vi "AO_master_DM_WFS_v2.vi"() -> ()   [LabVIEW 2018]
uses:
  <userlib>/WaveKit.lib/Controls/Image information.ctl
  <userlib>/WaveKit.lib/Controls/Image general information.ctl
  <userlib>/WaveKit.lib/Controls/Image acquisition information.ctl
  <userlib>/WaveKit.lib/Controls/Point2D.ctl
  <userlib>/WaveKit.lib/Controls/Data alignment enum.ctl
  <userlib>/WaveKit.lib/Controls/StatisticsData.ctl
  <userlib>/WaveKit.lib/Controls/Wavefront Corrector states - ONE.ctl
  Drivers and controls/ASI/ASI_VIs/ASI Library/Shared_Serial/Axis Name.ctl
  <userlib>/WaveKit.lib/Classes/Camera/Camera.lvclass
  <userlib>/WaveKit.lib/Classes/CameraSet/CameraSet.lvclass
  <userlib>/WaveKit.lib/Classes/Image/Image.lvclass
  <userlib>/WaveKit.lib/Classes/Phase/Phase.lvclass
  <userlib>/WaveKit.lib/Controls/HasoSlopes.lvclass
  <userlib>/WaveKit.lib/Controls/Pupil.lvclass
  <userlib>/WaveKit.lib/Classes/WavefrontCorrector/WavefrontCorrector.lvclass
  <userlib>/WaveKit.lib/Classes/WavefrontCorrectorSet/WavefrontCorrectorSet.lvclass
  <userlib>/WaveKit.lib/Classes/HasoEngine/HasoEngine.lvclass
  <userlib>/WaveKit.lib/Controls/SlopesEngineSetup.ctl
  <userlib>/WaveKit.lib/Controls/WavefrontReconstructionMode.ctl
  <vilib>/Utility/file.llb/Read From Spreadsheet File (DBL).vi
  <vilib>/Analysis/1siggen.llb/Ramp Pattern by Delta.vi
  <userlib>/WaveKit.lib/Classes/ModalCoef/ModalCoef.lvclass
  <vilib>/Analysis/NI_AALBase.lvlib
panel:
  in  "File Type":enum16{"TIFF", "Sif"}(ring)
  in  "Spool":bool=TRUE caption="Cameras Live Display"
  in  "Device Status":enum32{"DM", "WFS", "Camera", "Others"}(tab)=enum."Camera"
  out "DM Actuator Values":sgl[](graph)
  out "Initial State":T1[](array[typedef])
  out "ActuatorsNumber":i32
  out "Initial Positions":sgl[](array[numeric])
  out "Final Positions":sgl[](array[numeric])
  in  "Coef Min":dbl=-0.5 min=1.0
  in  "Coef Max":dbl=0.5 min=1.0
  out "Zernike Measured":dbl[](graph)
  out "Phase statistics":T2
  out "Phase values":sgl[][](graph)=[[nan, nan, nan, nan, nan, nan, nan, nan, nan, nan, nan, nan, nan, nan, nan, nan, nan, nan, nan, nan, nan, nan, nan, nan, nan, nan, nan, nan, nan, nan, nan, nan, nan, nan, nan, nan, nan, nan, nan, nan], [nan, nan, nan, nan, nan, nan, nan, nan, nan, nan, nan, nan, nan, nan, nan, nan, nan, nan, nan, nan, nan, nan, nan, nan, nan, nan, nan, nan, nan, nan, nan, nan, nan, nan, nan, nan, nan, nan, nan, nan], [nan, nan, nan, nan, nan, nan, nan, nan, nan, nan, nan, nan, nan, nan, nan, nan, nan, nan, nan, nan, nan, nan, nan, nan, nan, nan, nan, nan, nan, nan, nan, nan, nan, nan, nan, nan, nan, nan, nan, nan], [nan, nan, nan, nan, nan, nan, nan, nan, nan, nan, nan, nan, nan, nan, nan, nan, nan, nan, nan, nan, nan, nan, nan, nan, nan, nan, nan, nan, nan, nan, nan, nan, nan, nan, nan, nan, nan, nan, nan, nan], [nan, nan, nan, nan, nan, nan, nan, nan, nan, nan, nan, nan, nan, nan, -0.14441992, nan, 0.1501734, 0.22490476, 0.2674259, 0.28415325, 0.2792031, 0.2552752, 0.21375881, 0.15405469, nan, nan, nan, nan, nan, nan, nan, nan, nan, nan, nan, nan, nan, nan, nan, nan], [nan, nan, nan, nan, nan, nan, nan, nan, nan, nan, nan, nan, nan, nan, 0.19143742, 0.2795512, 0.33646506, 0.37099743, 0.3877919, 0.3894302, 0.37774685, 0.35447162, 0.3212538, 0.27904776, 0.22675864, 0.15897867, nan, nan, nan, nan, nan, nan, nan, nan, nan, nan, nan, nan, nan, nan], [nan, nan, nan, nan, nan, nan, nan, nan, nan, nan, nan, nan, nan, 0.22618562, 0.290776, 0.33285964, 0.36044422, 0.3767934, 0.38285175, 0.37884915, 0.3652757, 0.3433441, 0.3149789, 0.28229773, 0.2464756, 0.20580466, 0.15268901, 0.06923797, nan, nan, nan, nan, nan, nan, nan, nan, nan, nan, nan, nan], [nan, nan, nan, nan, nan, nan, nan, nan, nan, nan, nan, nan, 0.19992779, 0.24616541, 0.27565512, 0.29675642, 0.31222007, 0.32191983, 0.32467726, 0.31943765, 0.30597392, 0.2852214, 0.25927368, 0.2309889, 0.20308714, 0.17653626, 0.14795627, 0.10568966, 0.024115691, nan, nan, nan, nan, nan, nan, nan, nan, nan, nan, nan], [nan, nan, nan, nan, nan, nan, nan, nan, nan, nan, nan, 0.14862825, 0.18219855, 0.20114602, 0.21551609, 0.22862102, 0.24014233, 0.24817906, 0.2505626, 0.24567793, 0.23295718, 0.21313797, 0.18829979, 0.16161954, 0.1367108, 0.11633411, 0.10019377, 0.081457645, 0.04156301, -0.057204023, nan, nan, nan, nan, nan, nan, nan, nan, nan, nan], [nan, nan, nan, nan, nan, nan, nan, nan, nan, nan, 0.08899155, 0.117771566, 0.12948777, 0.13732892, 0.14631097, 0.15688494, 0.16728252, 0.17497937, 0.17758016, 0.17335457, 0.16157834, 0.14275661, 0.11873307, 0.09261118, 0.06834036, 0.04974218, 0.038678437, 0.031985473, 0.016725859, -0.03676957, nan, nan, nan, nan, nan, nan, nan, nan, nan, nan], [nan, nan, nan, nan, nan, nan, nan, nan, nan, nan, 0.058377307, 0.069048055, 0.0725615, 0.07683456, 0.0840318, 0.09335055, 0.10271386, 0.1097376, 0.11226265, 0.10867052, 0.09812171, 0.08078306, 0.058033932, 0.032565817, 0.008214329, -0.010712444, -0.020921554, -0.022825297, -0.02489755, -0.05023362, -0.14592764, nan, nan, nan, nan, nan, nan, nan, nan, nan], [nan, nan, nan, nan, nan, nan, nan, nan, nan, -0.0018393314, 0.018310271, 0.023098737, 0.024714457, 0.027986258, 0.033823933, 0.041292578, 0.048749834, 0.054400377, 0.056548227, 0.05374936, 0.04499338, 0.029967438, 0.009379062, -0.014759185, -0.03905803, -0.059140373, -0.070816256, -0.0724436, -0.06894927, -0.07806298, -0.1393881, nan, nan, nan, nan, nan, nan, nan, nan, nan], [nan, nan, nan, nan, nan, nan, nan, nan, nan, -0.03322208, -0.017045017, -0.0123043535, -0.010394985, -0.007970343, -0.0042642877, 0.0003761826, 0.005164365, 0.009095938, 0.010986101, 0.009512841, 0.0033822758, -0.008344227, -0.02579559, -0.047820807, -0.071688615, -0.09321856, -0.107681155, -0.11187886, -0.10789668, -0.10908524, -0.14891545, -0.29341945, nan, nan, nan, nan, nan, nan, nan, nan], [nan, nan, nan, nan, nan, nan, nan, nan, nan, nan, -0.043187555, -0.03622458, -0.033755217, -0.03278728, -0.03198469, -0.030707732, -0.028716512, -0.026208155, -0.023933899, -0.023217455, -0.025771504, -0.03328519, -0.04682974, -0.06620631, -0.08943447, -0.1126552, -0.13079928, -0.13944486, -0.13836564, -0.13734597, -0.16491348, -0.2807172, nan, nan, nan, nan, nan, nan, nan, nan], [nan, nan, nan, nan, nan, nan, nan, nan, -0.13038255, -0.08328184, -0.060542934, -0.050779276, -0.048053104, -0.048984695, -0.05126809, -0.053124577, -0.05330209, -0.051303368, -0.04760214, -0.04368073, -0.041799206, -0.04448101, -0.05377527, -0.07043236, -0.09320336, -0.118551016, -0.14113419, -0.15550357, -0.15952203, -0.16009864, -0.18189941, -0.27977645, nan, nan, nan, nan, nan, nan, nan, nan], [nan, nan, nan, nan, nan, nan, nan, nan, -0.15416794, -0.09987456, -0.07151361, -0.05893044, -0.056102008, -0.058817875, -0.063637674, -0.067669004, -0.06878706, -0.06599128, -0.059670344, -0.051622536, -0.044753395, -0.042448726, -0.04769562, -0.062100213, -0.08502676, -0.11315687, -0.14084403, -0.16171429, -0.1720384, -0.17647736, -0.19687745, -0.284868, -0.53908885, -1.12795, nan, nan, nan, nan, nan, nan], [nan, nan, nan, nan, nan, nan, nan, nan, -0.17633308, -0.1131372, -0.07876157, -0.06330658, -0.060116876, -0.063924976, -0.07015394, -0.07493687, -0.07548633, -0.07052183, -0.060539607, -0.047784284, -0.035856243, -0.028966732, -0.030924596, -0.044017438, -0.06802279, -0.099662215, -0.13288532, -0.16044727, -0.17731819, -0.18653797, -0.20820689, -0.29237592, -0.5366785, nan, nan, nan, nan, nan, nan, nan], [nan, nan, nan, nan, nan, nan, nan, nan, -0.19826387, -0.12505035, -0.08430402, -0.06564974, -0.061443567, -0.06527472, -0.07152294, -0.07554153, -0.07411167, -0.0658889, -0.05163869, -0.034133032, -0.017655006, -0.0071354215, -0.007018423, -0.020031396, -0.046107426, -0.08178567, -0.12048963, -0.15415914, -0.17678727, -0.19048853, -0.21480094, -0.2999987, -0.54526997, nan, nan, nan, nan, nan, nan, nan], [nan, nan, nan, nan, nan, nan, nan, nan, -0.2214154, -0.13693352, -0.08914254, -0.06661926, -0.06048554, -0.06317037, -0.0681367, -0.07015528, -0.065784656, -0.053790003, -0.035310905, -0.013662348, 0.0062713036, 0.01901285, 0.01972933, 0.005542416, -0.023349542, -0.06307545, -0.10643376, -0.14466219, -0.17119798, -0.18806857, -0.21562657, -0.30642, -0.5640642, nan, nan, nan, nan, nan, nan, nan], [nan, nan, nan, nan, nan, nan, nan, nan, -0.24718054, -0.14940841, -0.093277775, -0.0658183, -0.056708053, -0.05720259, -0.059951056, -0.05929426, -0.051715773, -0.036192447, -0.014265999, 0.010266874, 0.032073133, 0.04536258, 0.04520398, 0.028878966, -0.0030008797, -0.045963787, -0.092160165, -0.13235793, -0.16002774, -0.17817038, -0.20961209, -0.31157303, -0.5953845, nan, nan, nan, nan, nan, nan, nan], [nan, nan, nan, nan, nan, nan, nan, nan, -0.27748746, -0.16290864, -0.09610232, -0.062047683, -0.048735943, -0.04617936, -0.046241976, -0.042900223, -0.03261665, -0.014586102, 0.009311387, 0.03494107, 0.05674191, 0.068891875, 0.0666744, 0.04783368, 0.0136316735, -0.030755527, -0.0769404, -0.115639456, -0.14119013, -0.15893419, -0.19620675, -0.31774768, nan, nan, nan, nan, nan, nan, nan, nan], [nan, nan, nan, nan, nan, nan, nan, nan, -0.31623095, -0.17884897, -0.09729818, -0.0539262, -0.03469713, -0.028198741, -0.025418447, -0.019910373, -0.008048305, 0.010862423, 0.034768496, 0.05942371, 0.07931873, 0.0889112, 0.08400761, 0.06307276, 0.028166434, -0.014867521, -0.057410896, -0.09080534, -0.111413695, -0.12868427, -0.17697167, -0.3319423, nan, nan, nan, nan, nan, nan, nan, nan], [nan, nan, nan, nan, nan, nan, nan, nan, nan, -0.20170604, -0.09850275, -0.0411539, -0.0131010795, -0.0011654077, 0.0047943285, 0.01185911, 0.023955166, 0.041901454, 0.06374147, 0.08542206, 0.1018104, 0.10796184, 0.10047772, 0.0787158, 0.04554086, 0.007227666, -0.027947046, -0.052963093, -0.06777905, -0.08820889, -0.15871821, nan, nan, nan, nan, nan, nan, nan, nan, nan], [nan, nan, nan, nan, nan, nan, nan, nan, nan, -0.24239759, -0.10614249, -0.026831074, 0.015322472, 0.03581071, 0.046350636, 0.05505173, 0.06651187, 0.08204405, 0.10016226, 0.11737824, 0.12928592, 0.13183476, 0.12261822, 0.10192663, 0.073240966, 0.042765103, 0.017522467, 0.0014635092, -0.0110412, -0.045025453, -0.15884721, nan, nan, nan, nan, nan, nan, nan, nan, nan], [nan, nan, nan, nan, nan, nan, nan, nan, nan, nan, -0.13597216, -0.021381527, 0.04426403, 0.07956008, 0.09847209, 0.110732496, 0.122154154, 0.13505057, 0.14887714, 0.16113368, 0.16849175, 0.16803522, 0.1584293, 0.14075197, 0.118653886, 0.09743117, 0.0815231, 0.06987105, 0.048498146, -0.020404778, nan, nan, nan, nan, nan, nan, nan, nan, nan, nan], [nan, nan, nan, nan, nan, nan, nan, nan, nan, nan, nan, -0.04876471, 0.05625415, 0.117832564, 0.15310521, 0.17423762, 0.18897903, 0.20128381, 0.21210447, 0.22038196, 0.22418612, 0.221881, 0.21311647, 0.19937092, 0.1836943, 0.16922635, 0.15598845, 0.13537171, 0.081669986, nan, nan, nan, nan, nan, nan, nan, nan, nan, nan, nan], [nan, nan, nan, nan, nan, nan, nan, nan, nan, nan, nan, nan, 0.014031529, 0.121263236, 0.18738765, 0.22803904, 0.25380248, 0.2710389, 0.28282017, 0.2899857, 0.29225817, 0.2892868, 0.28139976, 0.26978248, 0.25571787, 0.23844866, 0.21115, 0.15442081, nan, nan, nan, nan, nan, nan, nan, nan, nan, nan, nan, nan], [nan, nan, nan, nan, nan, nan, nan, nan, nan, nan, nan, nan, nan, nan, 0.15212902, 0.2306162, 0.28129596, 0.31381333, 0.33402625, 0.3450995, 0.34855807, 0.34515002, 0.33529556, 0.31882071, 0.29360068, 0.25266168, nan, nan, nan, nan, nan, nan, nan, nan, nan, nan, nan, nan, nan, nan], [nan, nan, nan, nan, nan, nan, nan, nan, nan, nan, nan, nan, nan, nan, nan, nan, 0.1979487, 0.2623494, 0.30271748, 0.32490522, 0.33223343, 0.3261181, 0.30614072, 0.26925305, nan, nan, nan, nan, nan, nan, nan, nan, nan, nan, nan, nan, nan, nan, nan, nan], [nan, nan, nan, nan, nan, nan, nan, nan, nan, nan, nan, nan, nan, nan, nan, nan, nan, nan, nan, nan, nan, nan, nan, nan, nan, nan, nan, nan, nan, nan, nan, nan, nan, nan, nan, nan, nan, nan, nan, nan], [nan, nan, nan, nan, nan, nan, nan, nan, nan, nan, nan, nan, nan, nan, nan, nan, nan, nan, nan, nan, nan, nan, nan, nan, nan, nan, nan, nan, nan, nan, nan, nan, nan, nan, nan, nan, nan, nan, nan, nan], [nan, nan, nan, nan, nan, nan, nan, nan, nan, nan, nan, nan, nan, nan, nan, nan, nan, nan, nan, nan, nan, nan, nan, nan, nan, nan, nan, nan, nan, nan, nan, nan, nan, nan, nan, nan, nan, nan, nan, nan]] caption="Wavefront"
  out "HASO intensity":u32[][](graph)
  out "Intensity Graph":i32[][](graph)
  in  "Intensity Max":dbl=10000.0 min=1.0
  in  "Intensity Min":dbl=200.0 min=1.0
  in  "Auto Scale":bool=TRUE caption="PD Correction"
  out "Detector X Pixels":i32
  out "Detector Y Pixels":i32
  out "Current Temp":i32
  out "FOV X Pixels":i32
  out "FOV Y Pixels":i32
  out "Running Status":T3(ring) caption="Camera FOV"
  out "EMCCD Status":bool
  out "Return from Start Acquisition":u32
  out "Return from GetAcquiredData":u32
  out "Return from SetSpool":i32=1
  out "Return from GetStatus":u32
  out "Get Exposure Time":sgl format="%.4f"
  out "Return from CheckTimings":u32
  out "Get Accum Time":sgl format="%.4f"
  out "Get Kinetic Time":sgl format="%.4f"
  out "Get EMCCD Gain":i32=1
  out "Get Kinetic Num":i32=1
  out "Return from CheckProcess":u32
  in  "error in (no error)":errorcluster
  out "Current error":errorcluster
  out "AO output":path=path "D:/Data"
  out "nb_images (get)":u32=10
  out "exposure_duration_us (get)":u32
  out "Base Path":path=path "D:/Data"
  out "EMCCD output":path=path "D:/Data"
  in  "Current status":string="Test1"
  out "HASO ready":bool
  in  "Live Wavefront":bool
  in  "Update DM":bool
  in  "Tab Control":T4(tab)
  in  "EMCCD trigger port":tag="Dev1/port0/line0"
  in  "strPalette":string="C:\\Program Files\\Andor SOLIS\\GREY.PAL"
  in  "Initial haso file":path=path "D:/SystemAlignment/system_aberration_residual_20220406.has"
  in  "interaction matrix file":path=path "D:/SystemAlignment/IM_20220407_1p5sx2_0p5um.aomi"
  in  "DM configuration file":path=path "C:/Program Files (x86)/Imagine Optic/Configuration Files/WaveFrontCorrector_mirao52-e_0326.dat"
  in  "Haso configuration file":path=path "C:/Program Files (x86)/Imagine Optic/Configuration Files/HASO3_first_7364.dat"
  in  "Main Path":path=path "D:/Data"
  in  "Folder Name":string="Test"
  in  "Abort":bool
  in  "Snap":bool
  in  "Acquire":bool
  in  "Enable EMCCD":bool caption="PD Correction"
  in  "TurnOFFCooler":bool caption="PD Correction"
  in  "Shutdown EMCCD when exit":bool caption="PD Correction"
  in  "VISA Stage":refnum<visa-resource-name>="COM5"
  in  "Update FOV":bool
  in  "Yend":i32=1002
  in  "Xend":i32=1004
  in  "Ystart":i32=2
  in  "Xstart":i32=2
  in  "Ybin":i32=1
  in  "Xbin":i32=1
  in  "Camera FOV":T5(ring)=enum."Full FOV"
  in  "Update AcqSetting":bool
  in  "Exposure time (s)":dbl=0.02
  in  "Kinetic Num":u32=1
  in  "Accum Num":u32=1
  in  "Aquisition Mode":T6(ring)=enum."Single Scan" caption="Camera FOV"
  in  "Trigger Mode":enum16{"Internal", "External"}(ring) caption="Camera FOV"
  in  "Gain Value":sgl=20.0 format="%.2f"
  in  "Gain On":bool=TRUE caption="Cameras Live Display"
  in  "488 shutter":refnum<k7>(container)
  in  "Live EMCCD":bool
  in  "Initialize EMCCD":bool=TRUE caption="PD Correction"
  in  "CoolToTargetTemp":bool=TRUE caption="PD Correction"
  in  "Set Temp":i32=-60
  in  "Current Z as Center":bool=TRUE caption="PD Correction"
  in  "Subfolder EMCCD":string="test"
  in  "File Name":string="test"
  in  "Z Step Num":i32=7
  in  "Z Step Size (um)":dbl=0.2
  in  "right":bool
  in  "left":bool
  in  "front":bool
  in  "back":bool
  in  "XY step":dbl=1.0
  in  "down":bool
  in  "up":bool
  in  "Z step":dbl=1.0
  in  "flip mirror button":bool
  out "Response:":string="0\r"
  out "Position (um)":dbl[](array[numeric])=[0.0, 0.0, 0.0, -92.0, nan, nan] format="%#.1f"
  in  "Axis":T7[](array[typedef])=[enum."X", enum."Y", enum."Z", enum."Z", enum."F", enum."V"]
  in  "Command":string="W X"
  in  "Get Position":bool
  in  "Send":bool
  in  "Record Batch Actuator":bool
  in  "Coef value":dbl=0.5 min=1.0
  in  "Idx end":u32=20 min=1
  in  "Idx start":u32=1 min=1
  in  "Subfolder":string="Test1"
  in  "Net Rp":bool
  in  "Input type":T8(ring)=enum."Zernike Coef"
  in  "Additional Command":bool=TRUE
  in  "Offset command file":path=path "D:/SystemAlignment/system_aberration_20220414.dat"
  in  "Initial offset":bool=TRUE
  in  "Additional file":path=path "D:/SystemAlignment/system_aberration_20191029.dat"
  out "Coef out":sgl[](array[numeric])
  out "Index out":i32[](array[numeric])
  in  "Zern/DM index in":i32[](array[numeric])
  in  "Zern/DM coef in":sgl[](array[numeric])
  in  "idxType":enum16{"Wyant", "ANSI"}(ring)=enum."ANSI"
  in  "Filter":u8[](array[numeric])
  in  "exposure_duration_s (set)":dbl=1.0 min=1.0
  in  "nb_images (set)":u32=1 min=1
  in  "Save File":bool
  in  "File Base Name":string="Test"
  in  "Record Response":bool
  in  "Record Batch Zern":bool
  out "Acquisition information":T9={"Image general information"={"Camera serial number"="", "Smearing removed"=FALSE, "Background image removed"=FALSE, "Time Stamp"=timestamp(0 s since 1904-01-01), "Comment"="", "Camera_MAX_Level"=0}, "Acquisition information"={"Exposure duration (us)"=0, "Exposure duration specified (us)"=0, "Gain"=0.0, "Number of summed images"=0, "Trigger type"=""}, "Number of pixels"={"X"=0, "Y"=0}, "Number of bits"=enum."16"}
  in  "Init":bool
  in  "Reset error":bool
  in  "Exit":bool
  in  "Stop HASO":bool
  in  "Start HASO":bool
  # "AO_master_DM_WFS_v2.vi: (last update: 20220425)\nControl deformable mirror and wavefront sensor, check DM response, EMCCD preview and acquisition\n1, Add ASI stage and laser shutter control;\n2, Incorporate EMCCD control: 1) preview, 2) snap,  3) stack acquisition (by moving relative Z position);\n3,  Current bugs: 1) error --> shut down devices; 2) exit --> next initialization fails\na) DM ocuppied due to last unnormal exit; b) wavefront measure error: no laser, wrong slopes;"
  # "um"
  # "Available only if \"Live Wavefront\" is OFF"
  # "Not work well"
  # "Sample Stage"
  # "It takes some time to cool down the camera before it shutdowns"
  # "WF switch"
  # "Tilt 1/X: +"
  # "Defocus: +"
  # "C"
  # "Tilt 2/Y: -"
  # "1um = 10"
  # "Acquisition Settings"
  # "WFS no tilt: X502, Y520 @EMCCD"
  # "HASO Parameters"
  # "Check DM Response"
  # "Need to turn OFF live wavefront"
  # "Batch Range"
  # "Show in Wyant convention"
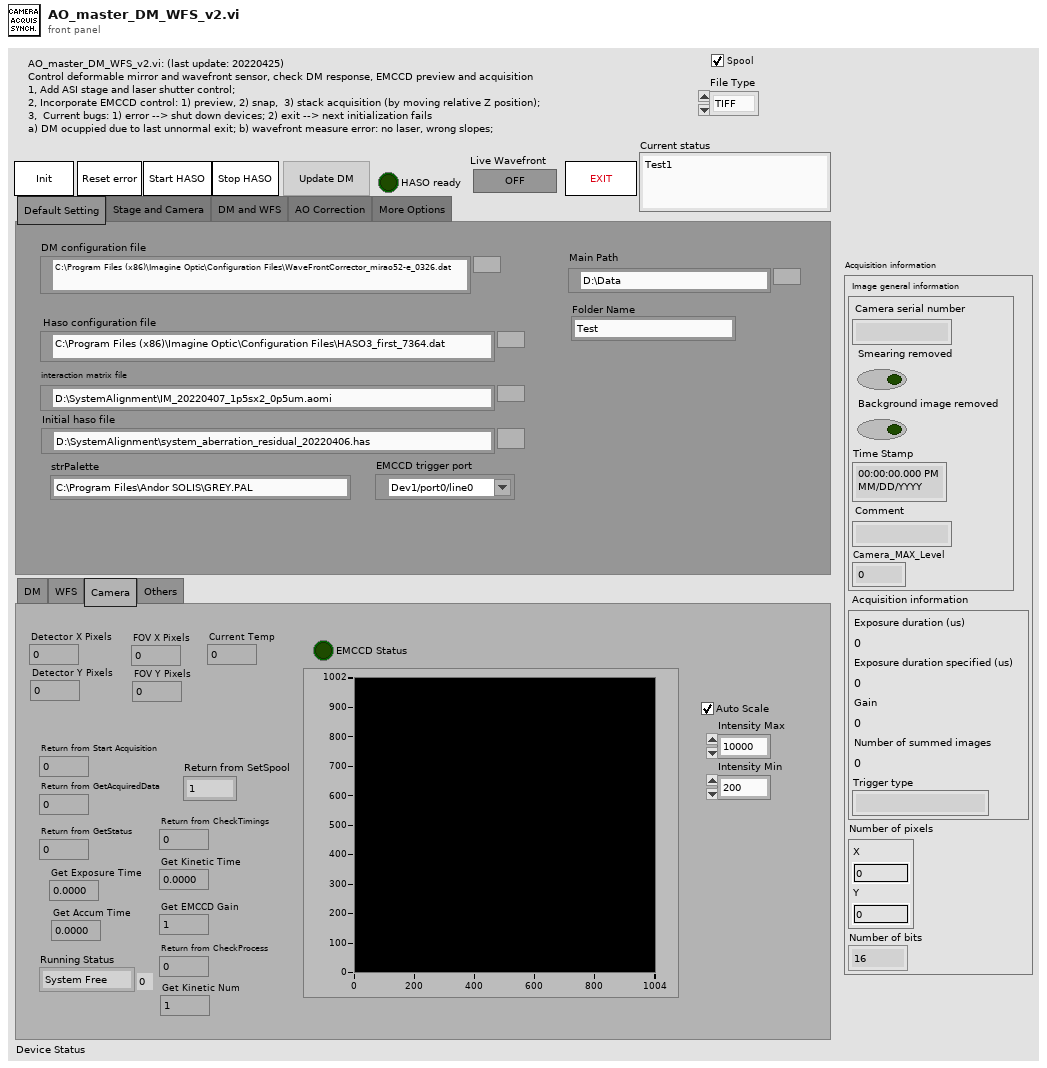
[diagram p1: front panel]
types:
  T1 = typedef "Wavefront Corrector states - ONE.ctl" = cluster{"Max":sgl, "Min":sgl, "Validity":enum16{"valid", "fixed", "invalid"}, "Fixed_Position":sgl}
  T2 = typedef "StatisticsData.ctl" = cluster{"PV":sgl, "RMS":dbl, "Max":sgl, "Min":sgl}
  T3 = enum16{"System Free", "Live Preview", "Snap", " Acquisition", ""}
  T4 = enum32{"Default Setting", "Stage and Camera", "DM and WFS", "AO Correction", "More Options"}
  T5 = enum16{"Custom FOV", "Full FOV", "FOV: 768x768", "FOV: 512x512", "FOV: 320x320", "FOV: 256x256", ""}
  T6 = enum16{"None", "Single Scan", "Accumulate", "Kinetics", "Fast Kinetics", "Run till abort"}
  T7 = typedef "Axis Name.ctl" = enum8{"undefined", "A", "B", "C", "D", "E", "F", "G", "H", "I", "J", "K", "L", "M", "N", "O", "P", "Q", "R", "S", "T", "U", "V", "W", "X", "Y", "Z"}
  T8 = enum16{"Zero Input", "Command File", "Zernike Coef", "Zernike File", "DM actuators"}
  T9 = typedef "Image information.ctl" = cluster{"Image general information":T10, "Acquisition information":T11, "Number of pixels":T12, "Number of bits":T13}
  T10 = typedef "Image general information.ctl" = cluster{"Camera serial number":string, "Smearing removed":bool, "Background image removed":bool, "Time Stamp":timestamp, "Comment":string, "Camera_MAX_Level":i32}
  T11 = typedef "Image acquisition information.ctl" = cluster{"Exposure duration (us)":i32, "Exposure duration specified (us)":i32, "Gain":sgl, "Number of summed images":i32, "Trigger type":string}
  T12 = typedef "Point2D.ctl" = cluster{"X":u32, "Y":u32}
  T13 = typedef "Data alignment enum.ctl" = enum16{"8", "16", "32"}
  T14 = typedef "SlopesEngineSetup.ctl" = cluster{"Start sub-aperture":T12, "Pupil average":dbl}
  T15 = typedef "CameraSpecifications.ctl" = cluster{"Grabber name":string, "Camera name":string, "Camera sn":string, "Pixels_um":T16, "Maximum level":u32, "Data alignment":T13, "Is signed":bool, "Acquisition start":T12, "Acquisition length":T12, "MaxFrameRate_Hz":sgl, "Chip type":enum16{"Progressive scan", "Frame transfert"}}
  T16 = typedef "General dimensions definition.ctl" = cluster{"Size":T12, "Step":T17}
  T17 = typedef "Point2Df.ctl" = cluster{"X":sgl, "Y":sgl}
  T18 = typedef "Wavefront Corrector Position.ctl" = sgl[]
  T19 = typedef "WavefrontReconstructionMode.ctl" = enum16{"None", "Modal_Legendre", "Modal_Zernike", "Zonal", "Modal_Zonal_Zernike", "Modal_Zonal_Legendre"}
  T20 = typedef "Error Code Enum typedef.ctl" = enum32{"N/A (0)", "DRV_ERROR_CODES", "DRV_SUCCESS", "DRV_VXDNOTINSTALLED", "DRV_ERROR_SCAN", "DRV_ERROR_CHECK_SUM", "DRV_ERROR_FILELOAD", "DRV_UNKNOWN_FUNC", "DRV_ERROR_VXD_INIT", "DRV_ERROR_ADDRESS", "DRV_ERROR_PAGELOCK", "DRV_ERROR_PAGEUNLOCK", "DRV_ERROR_BOARDTEST", "DRV_ERROR_ACK", "DRV_ERROR_UP_FIFO", "DRV_ERROR_PATTERN", "N/A (16)", "DRV_ACQUISITION_ERRORS", "DRV_ACQ_BUFFER", "DRV_ACQ_DOWNFIFO_FULL", "DRV_PROC_UNKONWN_INSTRUCTION", "DRV_ILLEGAL_OP_CODE", "DRV_KINETIC_TIME_NOT_MET", "DRV_ACCUM_TIME_NOT_MET", "DRV_NO_NEW_DATA", "N/A (25)", "DRV_SPOOLERROR", "N/A (27)", "N/A (28)", "N/A (29)", "N/A (30)", "N/A (31)", "N/A (32)", "DRV_TEMPERATURE_CODES", "DRV_TEMPERATURE_OFF", "DRV_TEMPERATURE_NOT_STABILIZED", "DRV_TEMPERATURE_STABILIZED", "DRV_TEMPERATURE_NOT_REACHED", "DRV_TEMPERATURE_OUT_RANGE", "DRV_TEMPERATURE_NOT_SUPPORTED", "DRV_TEMPERATURE_DRIFT", "N/A (41)", "N/A (42)", "N/A (43)", "N/A (44)", "N/A (45)", "N/A (46)", "N/A (47)", "N/A (48)", "DRV_GENERAL_ERRORS", "DRV_INVALID_AUX", "DRV_COF_NOTLOADED", "DRV_FPGAPROG", "DRV_FLEXERROR", "DRV_GPIBERROR", "N/A (55)", "N/A (56)", "N/A (57)", "N/A (58)", "N/A (59)", "N/A (60)", "N/A (61)", "N/A (62)", "N/A (63)", "DRV_DATATYPE", "DRV_DRIVER_ERRORS", "DRV_P1INVALID", "DRV_P2INVALID", "DRV_P3INVALID", "DRV_P4INVALID", "DRV_INIERROR", "DRV_COFERROR", "DRV_ACQUIRING", "DRV_IDLE", "DRV_TEMPCYCLE", "DRV_NOT_INITIALIZED", "DRV_P5INVALID", "DRV_P6INVALID", "DRV_INVALID_MODE", "DRV_INVALID_FILTER", "DRV_I2CERRORS", "DRV_I2CDEVNOTFOUND", "DRV_I2CTIMEOUT", "DRV_P7INVALID", "N/A (84)", "N/A (85)", "N/A (86)", "N/A (87)", "N/A (88)", "N/A (89)", "DRV_IOCERROR", "DRV_VRMVERSIONERROR"}
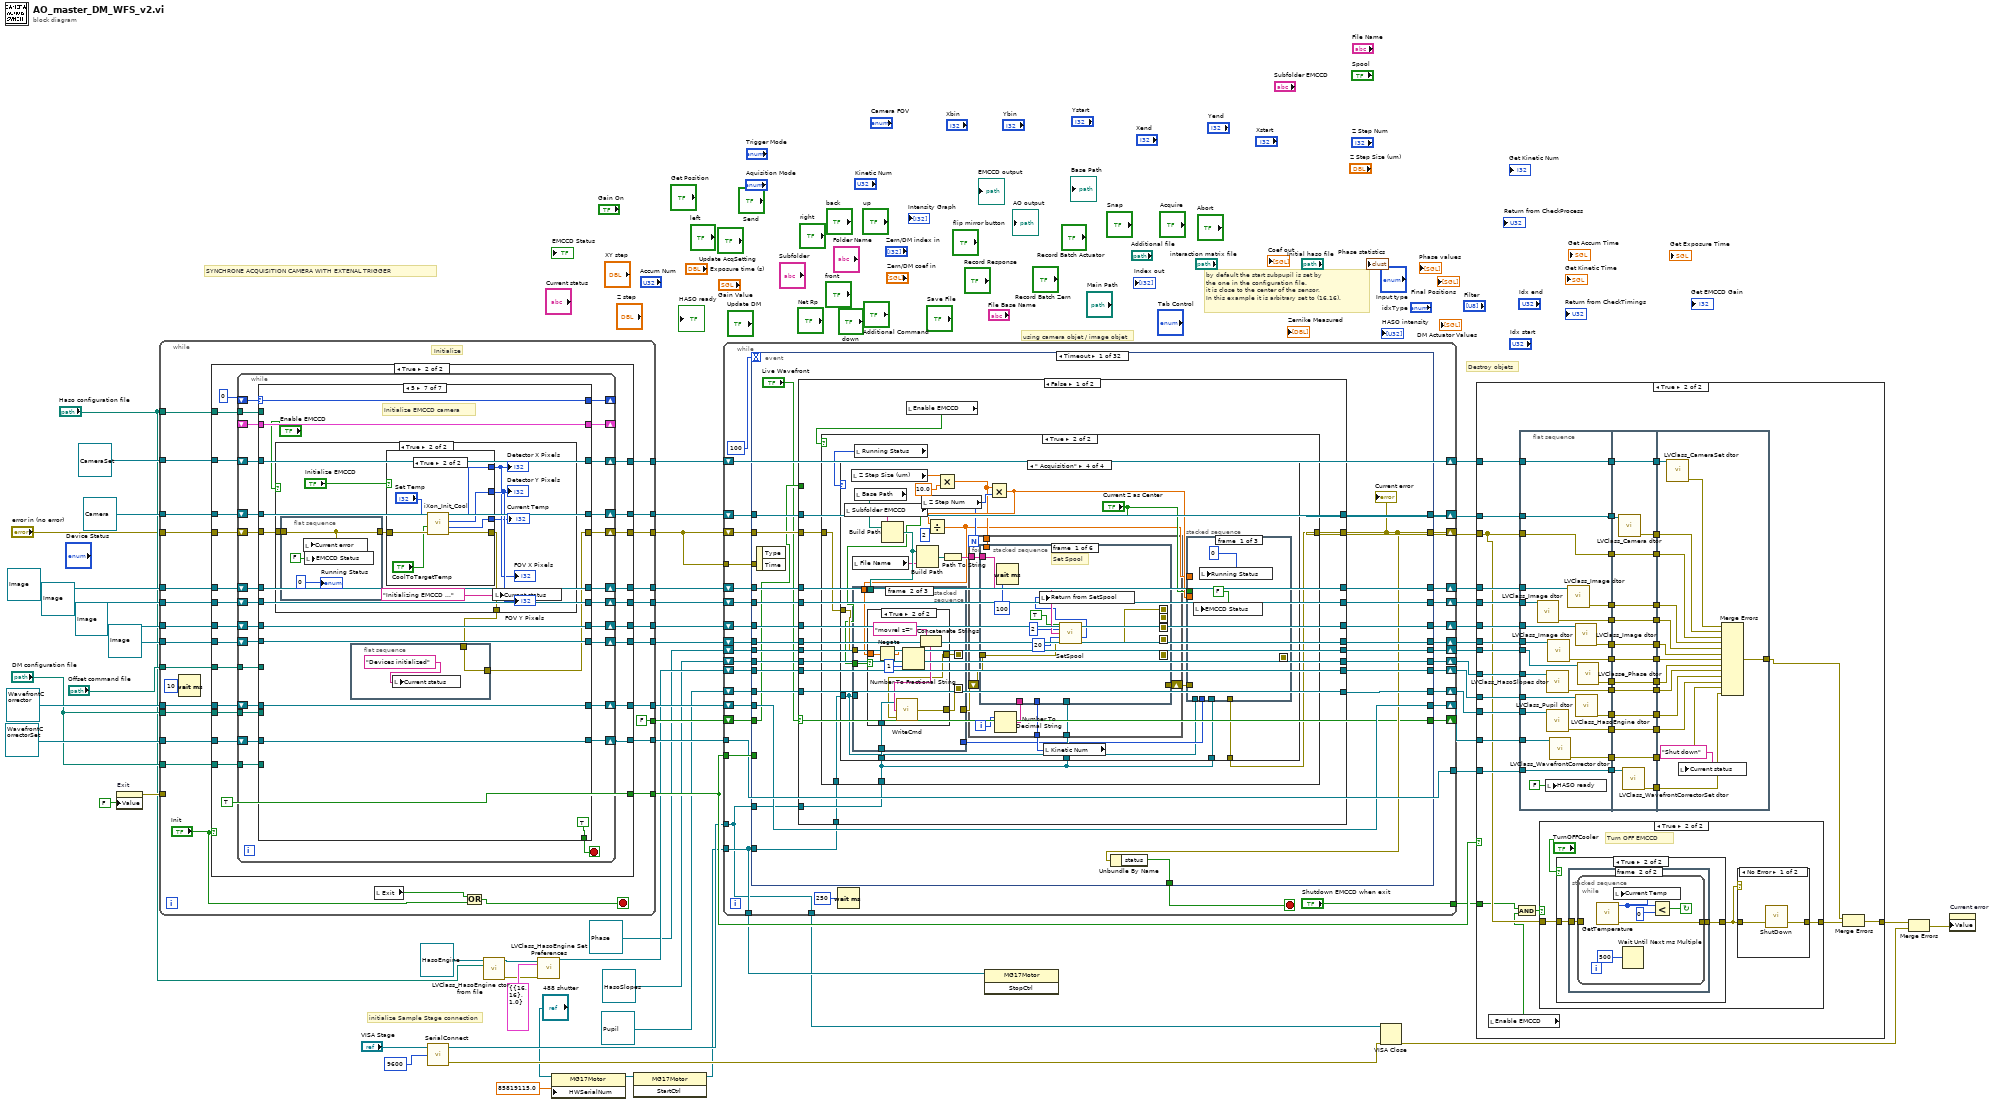
[diagram p0: block diagram]
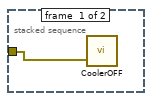
[diagram p5: hidden frame]
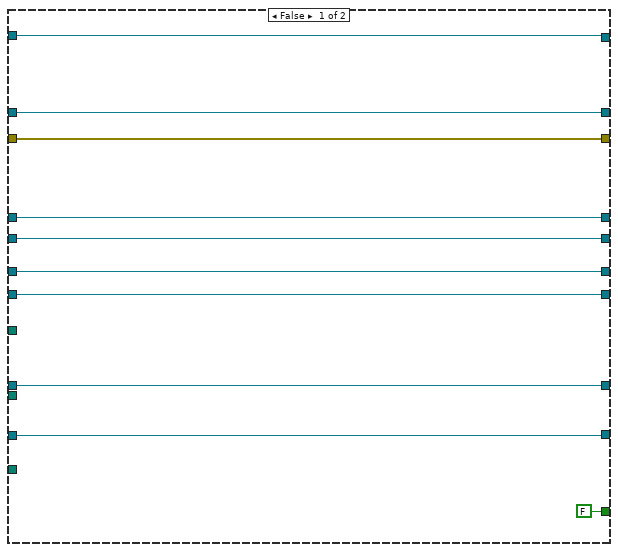
[diagram p7: hidden frame]
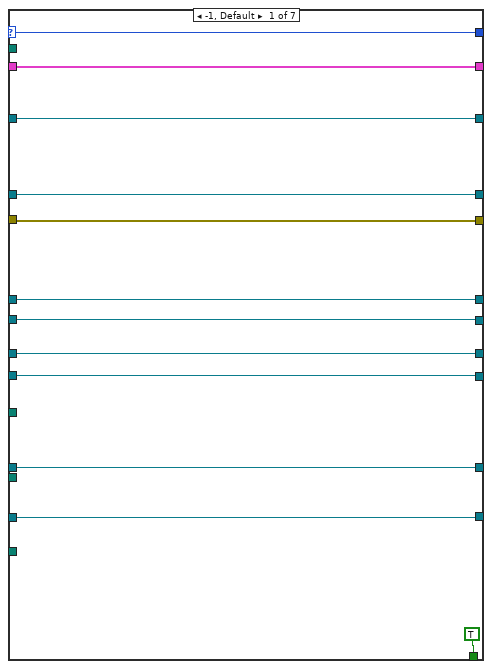
[diagram p8: hidden frame]
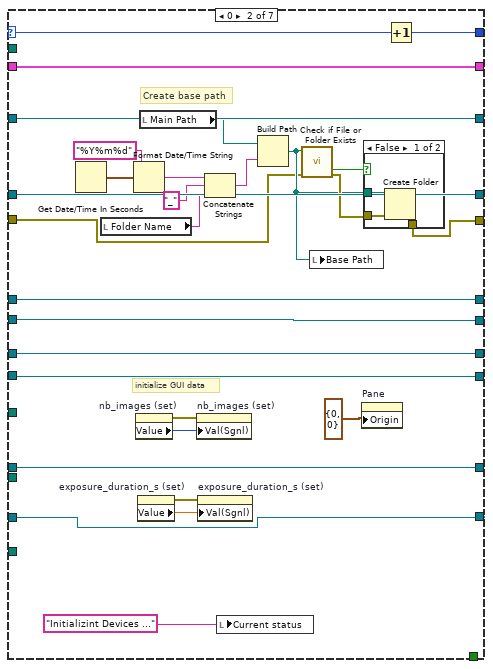
[diagram p9: hidden frame]
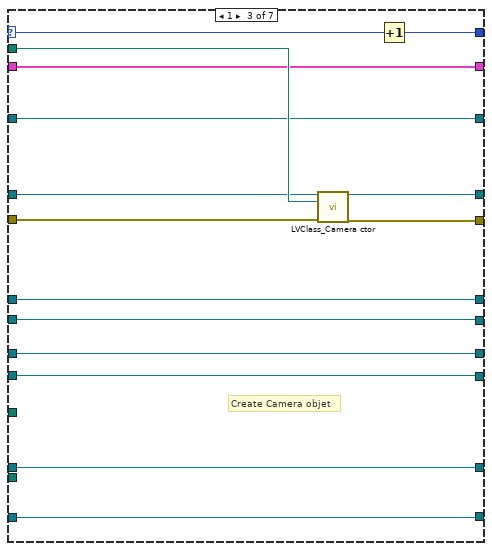
[diagram p11: hidden frame]
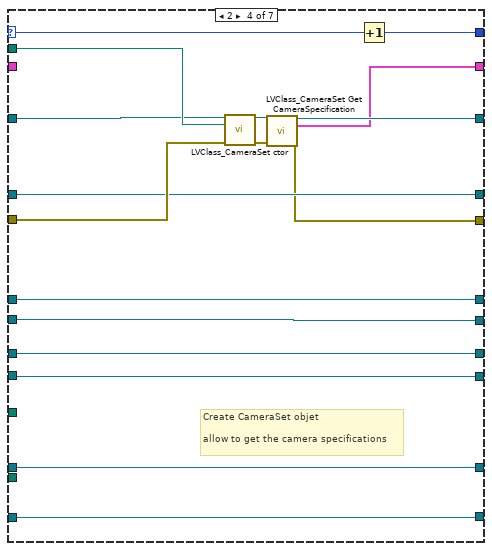
[diagram p12: hidden frame]
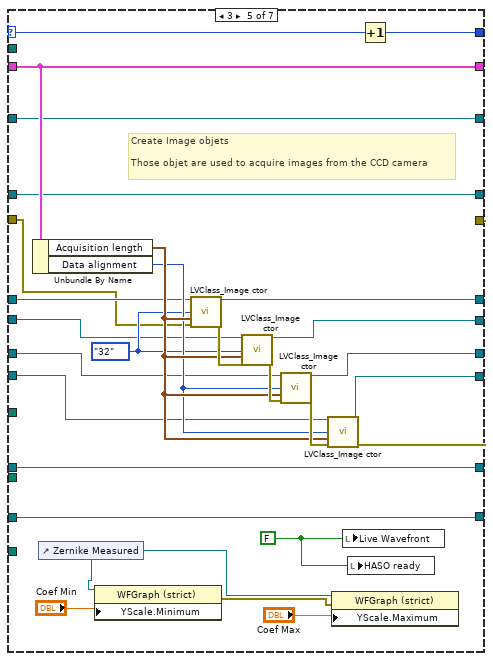
[diagram p13: hidden frame]
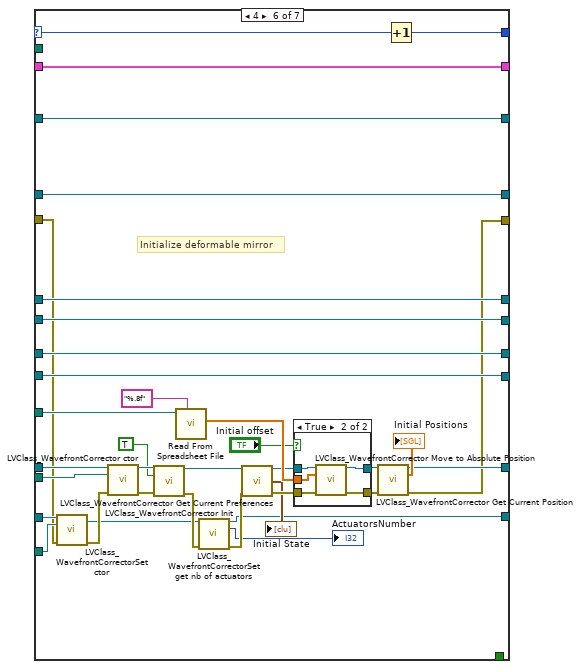
[diagram p14: hidden frame]
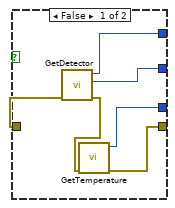
[diagram p17: hidden frame]
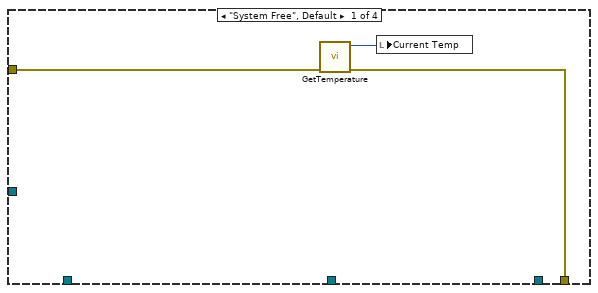
[diagram p19: hidden frame]
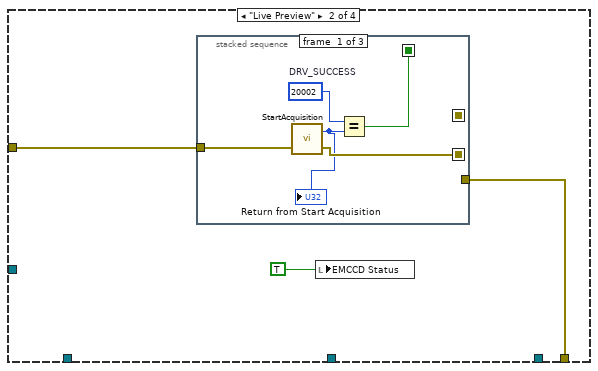
[diagram p20: hidden frame]
diagram:
  # "initialize Sample Stage connection"
  # "by default the start subpupil is set by \nthe one in the configuration file. \nit is close to the center of the sensor.\nIn this example it is arbitrary set to (16,16)."
  # "Destroy objets"
  # "using camera objet / image objet"
  # "SYNCHRONE ACQUISITION CAMERA WITH EXTENAL TRIGGER"
  n1 = property on="Exit" class="Bool (strict)"("Value"=FALSE ("Exit")) -> (error out=w37:errorcluster)  [unwired: 2 in, 1 out]
  n2 = while {
    tunnel: [FALSE] -> w53
    tunnel: [w87] -> w52
    tunnel: [w86] -> w51
    tunnel: [w85] -> w50
    tunnel: [w84] -> w49
    tunnel: [w83] -> w48
    tunnel: [w82] -> w47
    tunnel: refnum<class "Camera.lvclass"> refnum ("Camera.lvclass") -> [w81]
    tunnel: refnum<class "CameraSet.lvclass"> refnum ("CameraSet.lvclass") -> [w80]
    tunnel: refnum<class "Image.lvclass"> refnum ("Image in") -> [w79]
    tunnel: refnum<class "Image.lvclass"> refnum ("Image in") -> [w78]
    tunnel: refnum<class "Image.lvclass"> refnum ("Image in") -> [w77]
    tunnel: refnum<class "Image.lvclass"> refnum ("Image in") -> [w76]
    tunnel: "error in (no error)" -> [w75]
    tunnel: [w74] -> w40
    tunnel: [w72] -> w39
    tunnel: w37 -> [_]
    tunnel: "Haso configuration file" -> [w68]
    tunnel: "Offset command file" -> [w67]
    tunnel: refnum<class "WavefrontCorrectorSet.lvclass"> refnum ("WavefrontCorrectorSet in") -> [w66]
    tunnel: "DM configuration file" -> [w65]
    tunnel: refnum<class "WavefrontCorrector.lvclass"> refnum ("WavefrontCorrector in") -> [w64]
    tunnel: "DM configuration file" -> [w63]
    tunnel: [w62] -> w32
    tunnel: [w61] -> w31
    stop <- w69 stop-if-true
    # "Initialize"
    n3 = Wait (ms)(milliseconds to wait=u32 10) -> ()  [unwired: 1 out]
    n4 = case shown="True" "Init" {
      tunnel: [w98 w122] -> w87
      tunnel: [w97 w121] -> w86
      tunnel: [w95 w120] -> w85
      tunnel: [w94 w119] -> w84
      tunnel: [w93 w118] -> w83
      tunnel: [w92 w117] -> w82
      tunnel: w81 -> [w98 w116]
      tunnel: w80 -> [w97 w114]
      tunnel: w79 -> [w95 w113]
      tunnel: w78 -> [w94 w112]
      tunnel: w77 -> [w93 w111]
      tunnel: w76 -> [w92 w110]
      tunnel: w75 -> [w96 w109]
      tunnel: [w96 w108] -> w74
      tunnel: [FALSE TRUE] -> w72
      tunnel: w68 -> [_ w106]
      tunnel: w67 -> [_ w105]
      tunnel: w66 -> [w89 w99]
      tunnel: w65 -> [_ w104]
      tunnel: w64 -> [w90 w100]
      tunnel: w63 -> [_ w103]
      tunnel: [w90 w102] -> w62
      tunnel: [w89 w101] -> w61
      frame False {
      }
      frame True {
        n5 = while {
          tunnel: w106 -> [w147]
          shift-right: [w149] -> w122
          shift-left: w116 -> [w141]
          shift-right: [w131] -> _
          shift-left: 0 -> [w130]
          shift-right: [w148] -> w121
          shift-left: w114 -> [w140]
          shift-right: [w139] -> _
          shift-left: _ -> [w137]
          shift-right: [w146] -> w120
          shift-left: w113 -> [w138]
          shift-right: [w145] -> w119
          shift-left: w112 -> [w136]
          shift-right: [w144] -> w118
          shift-left: w111 -> [w134]
          shift-right: [w143] -> w117
          shift-left: w110 -> [w135]
          shift-right: [w142] -> w108
          shift-left: w109 -> [w132]
          tunnel: w105 -> [w129]
          tunnel: w104 -> [w128]
          tunnel: w103 -> [w127]
          shift-right: [w126] -> w102
          shift-left: w100 -> [w124]
          shift-right: [w125] -> w101
          shift-left: w99 -> [w123]
          stop <- w133 stop-if-true
          n6 = case shown="5" w130 {
            tunnel: [w161 w177 w209 w219 w241 w290 w312] -> w149
            tunnel: w147 -> [_ _ w208 w223 _ _ _]
            tunnel: [w160 w181 w206 w224 w242 w289 w311] -> w148
            tunnel: [w153 w182 w200 w214 w248 w284 w305] -> w146
            tunnel: [w154 w183 w201 w215 w247 w285 w306] -> w145
            tunnel: [w155 w184 w202 w216 w246 w286 w307] -> w144
            tunnel: [w156 w185 w203 w217 w245 w287 w308] -> w143
            tunnel: [w157 w163 w205 w218 w244 w258 w298] -> w142
            selector: w130 -> [w152 w179 w198 w213 w236 w256 w304]
            tunnel: w141 -> [w161 w177 w207 w219 w241 w290 w312]
            tunnel: w140 -> [w160 w181 w206 w222 w242 w289 w311]
            tunnel: [w158 w178 w204 w221 w243 w288 w309] -> w139
            tunnel: w138 -> [w153 w182 w200 w214 w240 w284 w305]
            tunnel: w137 -> [w158 w178 w204 _ w243 w288 w309]
            tunnel: w136 -> [w154 w183 w201 w215 w239 w285 w306]
            tunnel: w135 -> [w156 w185 w203 w217 w238 w287 w308]
            tunnel: w134 -> [w155 w184 w202 w216 w237 w286 w307]
            tunnel: [TRUE _ _ _ _ _ TRUE] -> w133
            tunnel: w132 -> [w157 w164 w197 w220 w234 w259 w301]
            tunnel: [w152 w180 w199 w212 w235 w255 w304] -> w131
            tunnel: w129 -> [_ _ _ _ _ w266 _]
            tunnel: w123 -> [w150 w175 w195 w210 w232 w264 w302]
            tunnel: w128 -> [_ _ _ _ _ w263 _]
            tunnel: w124 -> [w151 w176 w196 w211 w233 w262 w303]
            tunnel: w127 -> [_ _ _ _ _ w261 _]
            tunnel: [w151 w176 w196 w211 w233 w260 w303] -> w126
            tunnel: [w150 w175 w195 w210 w232 w257 w302] -> w125
            frame -1, Default {
            }
            frame 0 {
              # "Create base path"
              # "initialize GUI data"
              n7 = Get Date/Time In Seconds() -> (seconds since 1Jan1904=w169:timestamp)
              n8 = local read "Folder Name"() -> (w173:string)
              n9 = Format Date/Time String(time format string (%c)="%Y%m%d", seconds (now)=w169) -> (date/time string=w170:string)  [unwired: 1 in]
              n10 = property on="nb_images (set)" class="DigNum (strict)"() -> (error out=w190:errorcluster, "Value"=w189:u32)  [unwired: 2 in, 1 out]
              n11 = property on="exposure_duration_s (set)" class="DigNum (strict)"() -> (error out=w186:errorcluster, "Value"=w188:dbl)  [unwired: 2 in, 1 out]
              n12 = local read "Main Path"() -> (w172:path)
              n13 = property on="nb_images (set)" class="DigNum (strict)"(error in=w190, "Val(Sgnl)"=w189) -> ()  [unwired: 1 in, 2 out]
              n14 = property on="exposure_duration_s (set)" class="DigNum (strict)"(error in=w186, "Val(Sgnl)"=w188) -> ()  [unwired: 1 in, 2 out]
              n15 = Concatenate Strings(w170, "_", w173) -> (w171:string)
              n16 = local write "Current status"("Initializint Devices ...") -> ()
              n17 = Build Path(base path=w172, name or relative path=w171) -> (appended path=w165:path)
              n18 = call <vilib>:"Check if File or Folder Exists.vi"("error in (no error)"=w164, "path"=w165) -> ("error out"=w174:errorcluster, "file or folder exists?"=w168:bool)  [unwired: 7 in, 1 out]
              n19 = local write "Base Path"(w165) -> ()
              n20 = property on="Pane" class="Pane"("Origin"=cluster{"Horizontal":i16, "Vertical":i16} {"Horizontal"=0, "Vertical"=0} ("Front Panel Window:Origin")) -> ()  [unwired: 2 in, 2 out]
              n21 = case shown="False" w168 {
                tunnel: w165 -> [w193 _]
                tunnel: w174 -> [w192 w194]
                tunnel: [w191 w194] -> w163
                frame False {
                  n22 = Create Folder(path (use dialog)=w193, error in=w192) -> (error out=w191:errorcluster)  [unwired: 1 in, 2 out]
                }
                frame True {
                }
              }
              n23 = Increment(x=w179) -> (x+1=w180:i32)
            }
            frame 1 {
              # "Create Camera objet"
              n24 = call <userlib>:"LVClass_Camera ctor.vi"("Camera"=w207, "Configuration file path"=w208, "error in (no error)"=w197) -> ("Camera (new)"=w209:refnum<class "Camera.lvclass">, "error out"=w205:errorcluster)  [unwired: 11 in]
              n25 = Increment(x=w198) -> (x+1=w199:i32)
            }
            frame 2 {
              # "Create CameraSet objet\n\nallow to get the camera specifications"
              n26 = call <userlib>:"LVClass_CameraSet ctor.vi"("CameraSet.lvclass"=w222, "Configuration file path"=w223, "error in (no error)"=w220) -> ("CameraSet.lvclass"=w226:refnum<class "CameraSet.lvclass">, "error out"=w225:errorcluster)  [unwired: 11 in]
              n27 = call <userlib>:"LVClass_CameraSet Get CameraSpecification.vi"("CameraSet.lvclass"=w226, "error in (no error)"=w225) -> ("CameraSet.lvclass"=w224:refnum<class "CameraSet.lvclass">, "Camera Config"=w221:T15, "error out"=w218:errorcluster)  [unwired: 11 in]
              n28 = Increment(x=w213) -> (x+1=w212:i32)
            }
            frame 3 {
              w231 = FALSE
              w249 = Data_alignment_enum."32" ("Data alignment")
              # "Create Image objets\n\nThose objet are used to acquire images from the CCD camera"
              n29 = Unbundle By Name(w243) -> ("Acquisition length"=w251:T12, "Data alignment"=w250:T13)
              n30 = control-ref of="Zernike Measured"() -> (w228:refnum<vi>)
              n31 = property on="Property Node" class="WFGraph (strict)"(reference=w228, "YScale.Minimum"="Coef Min") -> (error out=w227:errorcluster)  [unwired: 1 in, 1 out]
              n32 = call <userlib>:"LVClass_Image ctor.vi"("Image in"=w240, "Data alignment"=w249, "Size"=w251, "error in (no error)"=w234) -> ("Image out"=w248:refnum<class "Image.lvclass">, "error out"=w252:errorcluster)  [unwired: 10 in]
              n33 = call <userlib>:"LVClass_Image ctor.vi"("Image in"=w239, "Data alignment"=w249, "Size"=w251, "error in (no error)"=w252) -> ("Image out"=w247:refnum<class "Image.lvclass">, "error out"=w253:errorcluster)  [unwired: 10 in]
              n34 = call <userlib>:"LVClass_Image ctor.vi"("Image in"=w237, "Data alignment"=w250, "Size"=w251, "error in (no error)"=w253) -> ("Image out"=w246:refnum<class "Image.lvclass">, "error out"=w254:errorcluster)  [unwired: 10 in]
              n35 = call <userlib>:"LVClass_Image ctor.vi"("Image in"=w238, "Data alignment"=w250, "Size"=w251, "error in (no error)"=w254) -> ("Image out"=w245:refnum<class "Image.lvclass">, "error out"=w244:errorcluster)  [unwired: 10 in]
              n36 = property on="Property Node" class="WFGraph (strict)"(reference=w228, error in=w227, "YScale.Maximum"="Coef Max") -> ()  [unwired: 2 out]
              n37 = local write "Live Wavefront"(w231) -> ()
              n38 = local write "HASO ready"(w231) -> ()
              n39 = Increment(x=w236) -> (x+1=w235:i32)
            }
            frame 4 {
              (unwired) "DM "
              (unwired) "DM "
              # "Initialize deformable mirror"
              n40 = call <userlib>:"LVClass_WavefrontCorrectorSet ctor.vi"("WavefrontCorrectorSet in"=w264, "PathToWavefrontCorrectorSetupFile"=w263, "error in (no error)"=w259) -> ("WavefrontCorrectorSet out"=w271:refnum<class "WavefrontCorrectorSet.lvclass">, "error out"=w280:errorcluster)  [unwired: 11 in]
              n41 = call <userlib>:"LVClass_WavefrontCorrector ctor.vi"("WavefrontCorrector in"=w262, "PathToWavefrontCorrectorSetupFile"=w261, "error in (no error)"=w280) -> ("WavefrontCorrector out"=w268:refnum<class "WavefrontCorrector.lvclass">, "error out"=w269:errorcluster)  [unwired: 11 in]
              n42 = call <userlib>:"LVClass_WavefrontCorrector Init.vi"("WavefrontCorrector in"=w268, "set_init_state_from_config_file"=TRUE, "error in (no error)"=w269) -> ("WavefrontCorrector out"=w272:refnum<class "WavefrontCorrector.lvclass">, "error out"=w281:errorcluster)  [unwired: 11 in]
              n43 = call-poly <vilib>:"Read From Spreadsheet File.vi"("format (%.3f)"="%.8f", "file path (dialog if empty)"=w266) -> ("first row"=w283:dbl[])  [unwired: 5 in, 4 out]
              n44 = call <userlib>:"LVClass_WavefrontCorrectorSet get nb of actuators.vi"("WavefrontCorrectorSet in"=w271, "error in (no error)"=w281) -> ("WavefrontCorrectorSet out"=w257:refnum<class "WavefrontCorrectorSet.lvclass">, "ActuatorsNumber"=→"ActuatorsNumber":i32, "error out"=w282:errorcluster)  [unwired: 11 in]
              n45 = call <userlib>:"LVClass_WavefrontCorrector Get Current Preferences.vi"("WavefrontCorrector in"=w272, "error in (no error)"=w282) -> ("WavefrontCorrector out"=w277:refnum<class "WavefrontCorrector.lvclass">, "Mirror preferences.Wavefront Corrector State"=→"Initial State":T1[], "error out"=w278:errorcluster)  [unwired: 10 in, 1 out]
              n46 = case shown="True" "Initial offset" {
                tunnel: w283 -> [_ w297]
                tunnel: [w292 w296] -> w275
                tunnel: [w291 w295] -> w276
                tunnel: w277 -> [w292 w294]
                tunnel: w278 -> [w291 w293]
                frame False {
                }
                frame True {
                  n47 = call <userlib>:"LVClass_WavefrontCorrector Move to Absolute Position.vi"("WavefrontCorrector in"=w294, "Absolute Positions"=w297, "error in (no error)"=w293) -> ("WavefrontCorrector out"=w296:refnum<class "WavefrontCorrector.lvclass">, "error out"=w295:errorcluster)  [unwired: 11 in]
                }
              }
              n48 = call <userlib>:"LVClass_WavefrontCorrector Get Current Position.vi"("WavefrontCorrector in"=w275, "error in (no error)"=w276) -> ("WavefrontCorrector out"=w260:refnum<class "WavefrontCorrector.lvclass">, "Wavefront Corrector Position"=→"Initial Positions":T18, "error out"=w258:errorcluster)  [unwired: 11 in]
              n49 = Increment(x=w256) -> (x+1=w255:i32)
            }
            frame 5 {
              # "Initialize EMCCD camera"
              n50 = case shown="True" "Enable EMCCD" {
                tunnel: w301 -> [w315 w318]
                tunnel: [w315 w316] -> w299
                frame False {
                }
                frame True {
                  n51 = flat-sequence {
                    tunnel: w318 -> [w326]
                    tunnel: [w326] -> w323
                    frame #0 {
                      n52 = local write "Current error"(w326) -> ()
                      n53 = local write "EMCCD Status"(FALSE) -> ()
                      "Running Status" <- u16 0
                    }
                  }
                  n54 = case shown="True" "Initialize EMCCD" {
                    tunnel: w323 -> [w331 w338]
                    tunnel: [w329 w336] -> w321
                    tunnel: [w328 w335] -> w322
                    tunnel: [w332 w334] -> w320
                    tunnel: [w327 w333] -> w316
                    frame False {
                      n55 = call <userlib>:"GetDetector.vi"("error in (no error)"=w331) -> ("error out"=w330:errorcluster, "ypixels"=w328:i32, "xpixels"=w329:i32)  [unwired: 3 in, 1 out]
                      n56 = call <userlib>:"GetTemperature.vi"("error in (no error)"=w330) -> ("error out"=w327:errorcluster, "temperature"=w332:i32)  [unwired: 3 in, 2 out]
                    }
                    frame True {
                      n57 = call "iXon_Init_Cool.vi"("error in (no error)"=w338, "CoolToTargetTemp"="CoolToTargetTemp", "Set Temp"="Set Temp") -> ("error out"=w333:errorcluster, "Current Temp"=w334:i32, "Detector Y Pixels"=w335:i32, "Detector X Pixels"=w336:i32)  [unwired: 5 in]
                    }
                  }
                  "Detector X Pixels" <- w321
                  "Detector Y Pixels" <- w322
                  "Current Temp" <- w320
                  "FOV X Pixels" <- w321
                  "FOV Y Pixels" <- w322
                  n58 = local write "Current status"("Initializing EMCCD ...") -> ()
                }
              }
              n59 = flat-sequence {
                tunnel: w299 -> [w313]
                tunnel: [w313] -> w298
                frame #0 {
                  n60 = local write "Current status"("Devices initialized") -> ()
                }
              }
            }
          }
        }
      }
    }
    n61 = local read "Exit"() -> (w71:bool)
    n62 = Or(x=w71, y="Init") -> (x .or. y?=w69:bool)
  }
  n63 = call "SerialConnect.vi"("baud rate (9600)"=9600, "VISA resource name"="VISA Stage") -> ("error out"=w6:errorcluster, "VISA out"=w12:refnum<visa-resource-name>)  [unwired: 1 in, 1 out]
  n64 = call <userlib>:"LVClass_HasoEngine ctor from file.vi"("HasoEngine in"=refnum<class "HasoEngine.lvclass"> refnum, "Configuration file path"="Haso configuration file") -> ("HasoEngine out"=w28:refnum<class "HasoEngine.lvclass">, "error out"=w29:errorcluster)  [unwired: 12 in]
  n65 = call <userlib>:"LVClass_HasoEngine Set Preferences.vi"("HasoEngine in"=w28, "Slopes_HasoEngine_Setup"=T14 {"Start sub-aperture"={"X"=16, "Y"=16}, "Pupil average"=1.0}, "error in (no error)"=w29) -> ("HasoEngine out"=w25:refnum<class "HasoEngine.lvclass">)  [unwired: 11 in, 1 out]
  n66 = property class="MG17Motor"(reference="488 shutter", "HWSerialNum"=85819115.0) -> (reference out=w4:refnum<k7>)  [unwired: 1 in, 1 out]
  n67 = invoke class="MG17Motor" method="StartCtrl"(reference=w4) -> (reference out=w1:refnum<k7>)  [unwired: 2 in, 2 out]
  n68 = while {
    shift-right: [w370] -> w60
    shift-left: w40 -> [w372]
    shift-right: [w368] -> w59
    shift-left: w52 -> [w369]
    shift-right: [w362] -> w58
    shift-left: w50 -> [w367]
    shift-right: [w361] -> w57
    shift-left: w49 -> [w366]
    shift-right: [w360] -> w56
    shift-left: w48 -> [w365]
    shift-right: [w359] -> w55
    shift-left: w47 -> [w364]
    shift-right: [w358] -> _
    shift-left: w53 -> [w363]
    shift-right: [w357] -> w54
    shift-left: w51 -> [w357]
    tunnel: w40 -> [w356]
    tunnel: w39 -> [w355]
    tunnel: w31 -> [w344]
    shift-right: [w352] -> w24
    shift-left: refnum<class "HasoSlopes.lvclass"> refnum ("HasoSlopes in") -> [w351]
    shift-right: [w350] -> w19
    shift-left: w25 -> [w353]
    shift-right: [w347] -> w20
    shift-left: refnum<class "Phase.lvclass"> refnum ("Phase in") -> [w349]
    shift-right: [w346] -> w18
    shift-left: refnum<class "Pupil.lvclass"> refnum ("Pupil in") -> [w348]
    tunnel: [w344] -> w17
    shift-right: [w343] -> w16
    shift-left: w32 -> [w345]
    tunnel: w12 -> [w341]
    tunnel: w1 -> [w342]
    tunnel: [w342] -> w11
    tunnel: [w341] -> w10
    tunnel: ["Shutdown EMCCD when exit"] -> w5
    stop <- w371 stop-if-true
    n69 = event shown="[0] Timeout" {
      selector: _ -> [_ _ _ _ _ _ _ _ _ _ _ _ _ _ _ _ _ _ _ _ _ _ _ _ _ _ _ _ _ _ _ _]
      dyn-events: _ -> [_ _ _ _ _ _ _ _ _ _ _ _ _ _ _ _ _ _ _ _ _ _ _ _ _ _ _ _ _ _ _ _]
      timeout: 100 -> [_ _ _ _ _ _ _ _ _ _ _ _ _ _ _ _ _ _ _ _ _ _ _ _ _ _ _ _ _ _ _ _]
      tunnel: w372 -> [w391 w780 w783 w796 _ w843 w859 w877 w905 w1025 w1067 w1180 w1201 w1209 w1217 w1225 w1233 w1241 w1250 w1264 w1278 w1292 w1306 w1320 w1333 w1363 w1376 w1404 w1961 w2490 _ w3244]
      tunnel: [w378 _ _ _ _ _ _ _ w906 _ _ _ _ _ _ _ _ _ _ _ _ _ _ _ _ _ _ w1405 w1962 w2491 "Exit" TRUE ("Exit")] -> w371
      tunnel: [w379 w778 w783 w796 w814 w838 w857 w883 w904 w1024 w1068 w1179 w1201 w1209 w1217 w1225 w1233 w1241 w1249 w1263 w1277 w1291 w1305 w1319 w1332 w1362 w1375 w1403 w1960 w2489 w3228 w3249] -> w370
      tunnel: w369 -> [w396 w779 w784 w797 w816 w842 w860 w884 w900 w1023 w1089 w1178 w1203 w1211 w1219 w1227 w1235 w1243 w1253 w1267 w1281 w1295 w1309 w1323 w1340 w1369 w1382 w1392 w1949 w2478 w3229 w3251]
      tunnel: [w395 w777 w784 w797 w816 w839 w858 w885 w900 w1023 w1089 w1178 w1203 w1211 w1219 w1227 w1235 w1243 w1253 w1267 w1281 w1295 w1309 w1323 w1340 w1369 w1382 w1392 w1949 w2478 w3227 w3250] -> w368
      tunnel: w367 -> [w399 w770 w791 w804 w818 w832 w855 w879 w916 w1048 w1094 w1188 w1207 w1215 w1223 w1231 w1239 w1247 w1261 w1275 w1289 w1303 w1317 w1331 w1344 w1373 w1386 w1399 w1956 w2485 w3223 w3245]
      tunnel: w366 -> [w398 w771 w792 w805 w819 w833 w854 w880 w915 w1047 w1093 w1187 w1206 w1214 w1222 w1230 w1238 w1246 w1260 w1274 w1288 w1302 w1316 w1330 w1343 w1372 w1385 w1398 w1955 w2484 w3224 w3246]
      tunnel: w365 -> [w397 w772 w793 w806 w820 w834 w853 w881 w914 w1046 w1092 w1186 w1205 w1213 w1221 w1229 w1237 w1245 w1259 w1273 w1287 w1301 w1315 w1329 w1342 w1371 w1384 w1397 w1954 w2483 w3225 w3247]
      tunnel: w364 -> [w392 w773 w794 w807 w821 w835 w852 w882 w913 w1045 w1091 w1185 w1204 w1212 w1220 w1228 w1236 w1244 w1258 w1272 w1286 w1300 w1314 w1328 w1341 w1370 w1383 w1396 w1953 w2482 w3226 w3248]
      tunnel: w363 -> [w377 w769 w790 w803 w817 w831 _ _ w901 w1022 w1090 w1177 w1202 w1210 w1218 w1226 w1234 w1242 w1251 w1265 w1279 w1293 w1307 w1321 w1339 w1368 w1381 w1401 w1958 w2487 _ _]
      tunnel: [w394 w770 w791 w804 w818 w832 w855 w879 w916 w1048 w1094 w1188 w1207 w1215 w1223 w1231 w1239 w1247 w1261 w1275 w1289 w1303 w1317 w1331 w1344 w1373 w1386 w1399 w1956 w2485 w3223 w3245] -> w362
      tunnel: [w393 w771 w792 w805 w819 w833 w854 w880 w915 w1047 w1093 w1187 w1206 w1214 w1222 w1230 w1238 w1246 w1260 w1274 w1288 w1302 w1316 w1330 w1343 w1372 w1385 w1398 w1955 w2484 w3224 w3246] -> w361
      tunnel: [w390 w772 w793 w806 w820 w834 w853 w881 w914 w1046 w1092 w1186 w1205 w1213 w1221 w1229 w1237 w1245 w1259 w1273 w1287 w1301 w1315 w1329 w1342 w1371 w1384 w1397 w1954 w2483 w3225 w3247] -> w360
      tunnel: [w389 w773 w794 w807 w821 w835 w852 w882 w913 w1045 w1091 w1185 w1204 w1212 w1220 w1228 w1236 w1244 w1258 w1272 w1286 w1300 w1314 w1328 w1341 w1370 w1383 w1396 w1953 w2482 w3226 w3248] -> w359
      tunnel: ["Live Wavefront" w769 w790 w803 w817 w831 TRUE FALSE w901 w1022 w1090 w1177 w1202 w1210 w1218 w1226 w1234 w1242 w1251 w1265 w1279 w1293 w1307 w1321 w1339 w1368 w1381 w1401 w1958 w2487 FALSE FALSE] -> w358
      tunnel: w356 -> [_ _ _ _ w813 _ _ _ _ _ _ _ _ _ _ _ _ _ _ _ _ _ _ _ _ _ _ _ _ _ _ _]
      tunnel: w355 -> [_ _ _ _ _ _ _ _ _ _ _ _ _ _ _ _ _ _ _ _ _ _ _ _ _ _ _ _ _ _ w3221 _]
      tunnel: w351 -> [w388 w767 w788 w801 w811 w825 w850 w875 w897 _ _ _ _ _ _ _ _ _ _ _ _ _ _ _ _ _ _ w1394 w1951 w2480 w3219 w3241]
      tunnel: w353 -> [w387 w766 w787 w800 w810 w824 w849 w874 w896 _ _ _ _ _ _ _ _ _ _ _ _ _ _ _ _ _ _ w1393 w1950 w2479 w3218 w3240]
      tunnel: [w386 w767 w788 w801 w811 w825 w850 w875 w897 _ _ _ _ _ _ _ _ _ _ _ _ _ _ _ _ _ _ w1391 w1948 w2477 w3219 w3241] -> w352
      tunnel: [w385 w766 w787 w800 w810 w824 w849 w874 w896 _ _ _ _ _ _ _ _ _ _ _ _ _ _ _ _ _ _ w1393 w1950 w2479 w3218 w3240] -> w350
      tunnel: w349 -> [w384 w768 w789 w802 w812 w826 w851 w876 w898 _ _ _ _ _ _ _ _ _ _ _ _ _ _ _ _ _ _ w1395 w1952 w2481 w3220 w3242]
      tunnel: w348 -> [w383 w765 w786 w799 w809 w823 w848 w873 w895 _ _ _ _ _ _ _ _ _ _ _ _ _ _ _ _ _ _ w1389 w1946 w2475 w3217 w3239]
      tunnel: [w382 w768 w789 w802 w812 w826 w851 w876 w898 _ _ _ _ _ _ _ _ _ _ _ _ _ _ _ _ _ _ w1390 w1947 w2476 w3220 w3242] -> w347
      tunnel: [w381 w765 w786 w799 w809 w823 w848 w873 w895 _ _ _ _ _ _ _ _ _ _ _ _ _ _ _ _ _ _ w1388 w1945 w2474 w3217 w3239] -> w346
      tunnel: w345 -> [w380 w764 w785 w798 w808 w822 w847 w872 w903 _ _ _ _ _ _ _ _ _ _ _ _ _ _ _ _ _ _ w1402 w1959 w2488 w3216 w3238]
      tunnel: [w380 w764 w785 w798 w808 w822 w847 w872 w899 _ _ _ _ _ _ _ _ _ _ _ _ _ _ _ _ _ _ w1400 w1957 w2486 w3216 w3238] -> w343
      tunnel: w341 -> [w375 _ _ _ _ _ _ _ _ _ _ _ _ _ _ _ _ _ w1252 w1266 w1280 w1294 w1308 w1322 _ w1361 w1374 _ _ _ _ _]
      tunnel: w342 -> [w374 _ _ _ _ _ _ _ _ _ _ _ _ _ _ _ _ _ _ _ _ _ _ _ _ _ _ _ _ _ _ _]
      event Timeout {
        n70 = event-data() -> ()  [unwired: 1 in, 2 out]
        n71 = case shown="False" "Live Wavefront" {
          tunnel: [w402 w676] -> w379
          tunnel: w399 -> [w413 w679]
          tunnel: [w413 w679] -> w394
          tunnel: [w409 w675] -> w393
          tunnel: w397 -> [w412 w678]
          tunnel: w392 -> [w411 w677]
          tunnel: [w412 w678] -> w390
          tunnel: [w411 w677] -> w389
          tunnel: w398 -> [w409 w675]
          tunnel: w396 -> [w410 w673]
          tunnel: [w410 w674] -> w395
          tunnel: w391 -> [w403 w672]
          tunnel: w388 -> [w407 w671]
          tunnel: w387 -> [w406 w670]
          tunnel: [w407 w669] -> w386
          tunnel: [w406 w668] -> w385
          tunnel: w384 -> [w408 w667]
          tunnel: w383 -> [w405 w666]
          tunnel: [w408 w665] -> w382
          tunnel: [w405 w664] -> w381
          tunnel: w377 -> [_ w661]
          tunnel: w375 -> [w401 _]
          tunnel: w374 -> [w400 _]
          frame False {
            n72 = local read "Enable EMCCD"() -> (w404:bool)
            n73 = case shown="True" w404 {
              tunnel: w403 -> [w414 w418]
              tunnel: [w414 w417] -> w402
              tunnel: w401 -> [_ w416]
              tunnel: w400 -> [_ w415]
              frame False {
              }
              frame True {
                n74 = local read "Running Status"() -> (w419:T3)
                n75 = case shown="\" Acquisition\"" w419 {
                  tunnel: [w420 w425 w460 w541] -> w417
                  tunnel: w418 -> [w421 w424 w459 w540]
                  tunnel: w416 -> [_ _ _ w529]
                  tunnel: w416 -> [_ _ _ w527]
                  tunnel: w416 -> [_ _ _ w526]
                  tunnel: w415 -> [_ _ _ w521]
                  frame "System Free", Default {
                    n76 = call <userlib>:"GetTemperature.vi"("error in (no error)"=w421) -> ("error out"=w420:errorcluster, "temperature"=w422:i32)  [unwired: 3 in, 2 out]
                    n77 = local write "Current Temp"(w422) -> ()
                  }
                  frame "Live Preview" {
                    n78 = stacked-sequence {
                      seq-local: [w428 _ _] -> [_ w433 _]
                      seq-local: [_ w432 _] -> [_ _ w447]
                      seq-local: [w427 _ _] -> [_ w431 _]
                      tunnel: w424 -> [w429 _ _]
                      tunnel: [_ _ w446] -> w425
                      frame #0 {
                        w430 = 20002  # DRV_SUCCESS
                        n79 = call <userlib>:"StartAcquisition.vi"("error in (no error)"=w429) -> ("error out"=w428:errorcluster, "DLL error code"=w426:u32)  [unwired: 1 in]
                        "Return from Start Acquisition" <- w426
                        n80 = Equal?(x=w430, y=w426) -> (x = y?=w427:bool)
                      }
                      frame #1 {
                        n81 = case shown="False" w431 {
                          tunnel: w433 -> [w434 w436]
                          tunnel: [w434 w435] -> w432
                          frame False {
                          }
                          frame True {
                            n82 = while {
                              tunnel: w436 -> [w438]
                              tunnel: [w437] -> w435
                              stop <- w439 continue-if-true
                              w441 = u16 72  # DRV ACQUIRING
                              n83 = call <userlib>:"GetStatus.vi"("error in (no error)"=w438) -> ("error out"=w437:errorcluster, "status"=w440:T20)  [unwired: 2 in, 1 out]
                              n84 = Equal?(x=w440, y=w441) -> (x = y?=w439:bool)
                            }
                          }
                        }
                      }
                      frame #2 {
                        n85 = local read "FOV X Pixels"() -> (w450:i32)
                        n86 = local read "FOV Y Pixels"() -> (w449:i32)
                        n87 = Multiply(x=w449, y=w450) -> (x*y=w451:i32)
                        n88 = call <userlib>:"GetAcquiredData.vi"("error in (no error)"=w447, "size"=w451) -> ("error out"=w446:errorcluster, "DLL error code"=→"Return from GetAcquiredData":u32, "array"=w442:i32[])  [unwired: 1 in]
                        n89 = Multiply(x=1, y=w442) -> (x*y=w443:i32[])
                        n90 = Reshape Array(w443, w449, w450) -> (w448:i32[][])
                        n91 = local write "Intensity Graph"(w448) -> ()
                      }
                    }
                    n92 = local write "EMCCD Status"(TRUE) -> ()
                  }
                  frame "Snap" {
                    n93 = flat-sequence {
                      tunnel: [w506] -> w462
                      tunnel: w459 -> [w508]
                      tunnel: w461 -> [w509]
                      frame #0 {
                        # "Create folder"
                        n94 = local write "EMCCD Status"(TRUE) -> ()
                        n95 = call <vilib>:"Check if File or Folder Exists.vi"("error in (no error)"=w508, "path"=w509) -> ("error out"=w507:errorcluster, "file or folder exists?"=w511:bool, "dup path"=w510:path)  [unwired: 7 in]
                        n96 = case shown="False" w511 {
                          tunnel: w510 -> [w516 w518]
                          tunnel: [w515 w518] -> _
                          tunnel: w507 -> [w514 w517]
                          tunnel: [w513 w517] -> w506
                          frame False {
                            n97 = Create Folder(path (use dialog)=w516, error in=w514) -> (created path=w515:path, error out=w513:errorcluster)  [unwired: 1 in, 1 out]
                          }
                          frame True {
                          }
                        }
                      }
                    }
                    n98 = local read "File Name"() -> (w452:string)
                    n99 = local read "Base Path"() -> (w454:path)
                    n100 = local read "Subfolder EMCCD"() -> (w453:string)
                    n101 = Build Path(base path=w454, name or relative path=w453) -> (appended path=w461:path)
                    n102 = Build Path(base path=w461, name or relative path=w452) -> (appended path=w458:path)
                    n103 = Path To String(path=w458) -> (string=w457:string)
                    n104 = local read "Kinetic Num"() -> (w456:u32)
                    n105 = stacked-sequence {
                      seq-local: [_ w472 _ _ _] -> [_ _ w475 _ _]
                      seq-local: [_ _ w474 _ _] -> [_ _ _ w481 _]
                      seq-local: [w467 _ _ _ _] -> [_ w471 _ _ _]
                      seq-local: [_ _ _ w482 _] -> [_ _ _ _ w501]
                      tunnel: w462 -> [w468 _ _ _ _]
                      tunnel: w457 -> [w469 _ _ w483 w499]
                      tunnel: w456 -> [_ _ _ _ w502]
                      tunnel: [_ _ _ _ w500] -> w455
                      frame #0 {
                        # "Set Spool"
                        n106 = call <userlib>:"SetSpool.vi"("active"=TRUE, "method"=2, "name"=w469, "framebuffersize (10)"=20, "error in (no error)"=w468) -> ("DLL error code"=→"Return from SetSpool":u32, "error out"=w467:errorcluster)  [unwired: 9 in]
                      }
                      frame #1 {
                        w473 = 20002  # DRV_SUCCESS
                        n107 = call <userlib>:"StartAcquisition.vi"("error in (no error)"=w471) -> ("error out"=w472:errorcluster, "DLL error code"=w470:u32)  [unwired: 1 in]
                        n108 = local write "Return from Start Acquisition"(w470) -> ()
                        n109 = Equal?(x=w473, y=w470) -> ()  [unwired: 1 out]
                      }
                      frame #2 {
                        n110 = while {
                          tunnel: w475 -> [w478]
                          tunnel: [w477] -> w474
                          stop <- w479 continue-if-true
                          w480 = u16 72  # DRV ACQUIRING
                          n111 = call <userlib>:"GetStatus.vi"("error in (no error)"=w478) -> ("error out"=w477:errorcluster, "status"=w476:T20)  [unwired: 2 in, 1 out]
                          "Return from GetStatus" <- w476
                          n112 = Equal?(x=w476, y=w480) -> (x = y?=w479:bool)
                        }
                      }
                      frame #3 {
                        # "Save acquisition"
                        n113 = case shown="\"TIFF\", Default" "File Type" {
                          tunnel: "C:\\Program Files\\Andor SOLIS\\GREY.PAL" -> [w489 _]
                          tunnel: w483 -> [w492 w498]
                          tunnel: w481 -> [w490 w495]
                          tunnel: [w491 w494] -> w482
                          frame "TIFF", Default {
                            w486 = 1
                            n114 = Concatenate Strings(w492, ".tif") -> (w488:string)
                            n115 = call <userlib>:"SaveAsTiffEx.vi"("path"=w488, "palette"=w489, "position"=0, "type"=w486, "mode"=w486, "error in (no error)"=w490) -> ("error out"=w491:errorcluster)  [unwired: 12 in, 1 out]
                          }
                          frame "Sif" {
                            n116 = Concatenate Strings(w498, ".sif") -> (w496:string)
                            n117 = call <userlib>:"SaveAsSif.vi"("error in (no error)"=w495, "path"=w496) -> ("error out"=w494:errorcluster)  [unwired: 1 out]
                          }
                        }
                      }
                      frame #4 {
                        # "Clearn Spool Files"
                        n118 = call "cleanSpool.vi"("error in (no error)"=w501, "Total Img Num"=w502, "strPath"=w499) -> ("error out"=w500:errorcluster)  [unwired: 8 in]
                      }
                    }
                    n119 = flat-sequence {
                      tunnel: w455 -> [w504]
                      tunnel: [w504] -> w460
                      frame #0 {
                        n120 = local write "EMCCD Status"(FALSE) -> ()
                        n121 = local write "Running Status"(0) -> ()
                      }
                    }
                  }
                  frame " Acquisition" {
                    n122 = local read "Subfolder EMCCD"() -> (w535:string)
                    n123 = local read "Z Step Size (um)"() -> (w533:dbl)
                    n124 = local read "File Name"() -> (w534:string)
                    n125 = local read "Base Path"() -> (w536:path)
                    n126 = Build Path(base path=w536, name or relative path=w535) -> (appended path=w542:path)
                    n127 = Build Path(base path=w542, name or relative path=w534) -> (appended path=w539:path)
                    n128 = local read "Z Step Num"() -> (w523:i32)
                    n129 = Multiply(x=w533, y=10.0) -> (x*y=w520:dbl)
                    n130 = Path To String(path=w539) -> (string=w538:string)
                    n131 = Multiply(x=w520, y=w523) -> (x*y=w530:dbl)
                    n132 = Divide(x=w530, y=2) -> (x/y=w519:dbl)
                    n133 = stacked-sequence {
                      seq-local: [w627 _ _] -> [_ w641 _]
                      seq-local: [_ w640 _] -> [_ _ w659]
                      tunnel: w540 -> [w629 _ _]
                      tunnel: w542 -> [w630 _ _]
                      tunnel: [_ _ w657] -> w528
                      tunnel: w519 -> [_ w644 _]
                      tunnel: w527 -> [_ w643 _]
                      tunnel: "Current Z as Center" -> [_ w642 _]
                      tunnel: w521 -> [_ _ w658]
                      tunnel: [_ _ w656] -> w522
                      frame #0 {
                        # "Create folder"
                        n134 = local write "EMCCD Status"(TRUE) -> ()
                        n135 = call <vilib>:"Check if File or Folder Exists.vi"("error in (no error)"=w629, "path"=w630) -> ("error out"=w628:errorcluster, "file or folder exists?"=w632:bool, "dup path"=w631:path)  [unwired: 7 in]
                        n136 = case shown="True" w632 {
                          tunnel: w631 -> [w637 w639]
                          tunnel: [w636 w639] -> _
                          tunnel: w628 -> [w635 w638]
                          tunnel: [w634 w638] -> w627
                          frame False {
                            n137 = Create Folder(path (use dialog)=w637, error in=w635) -> (created path=w636:path, error out=w634:errorcluster)  [unwired: 1 in, 1 out]
                          }
                          frame True {
                          }
                        }
                      }
                      frame #1 {
                        n138 = case shown="True" w642 {
                          tunnel: [w645 w650] -> w640
                          tunnel: w644 -> [_ w649]
                          tunnel: w643 -> [_ w648]
                          tunnel: w641 -> [w645 w647]
                          frame False {
                          }
                          frame True {
                            n139 = Negate(x=w649) -> (-x=w654:dbl)
                            n140 = Number To Fractional String(number=w654, precision (6)=1) -> (F-format string=w653:string)  [unwired: 2 in]
                            n141 = Concatenate Strings("movrel z=", w653) -> (w652:string)
                            n142 = call "WriteCmd.vi"("error IO"=w647, "Command"=w652, "VISA resource name"=w648) -> ("error"=w650:errorcluster)
                          }
                        }
                      }
                      frame #2 {
                        # "Turn on laser"
                        n143 = invoke class="MG17Motor" method="SC_Enable"(reference=w658, error in=w659, "lChanID"=0) -> (error out=w657:errorcluster, "lChanID"=w656:i32)  [unwired: 1 in, 2 out]
                        n144 = Wait (ms)(milliseconds to wait=u32 1000) -> ()  [unwired: 1 out]
                      }
                    }
                    n145 = local read "Kinetic Num"() -> (w537:u32)
                    n146 = for {
                      N: w523 -> [_]
                      tunnel: w538 -> [w550]
                      tunnel: w537 -> [w549]
                      tunnel: w526 -> [w547]
                      tunnel: w520 -> [w545]
                      shift-right: [w546] -> w525
                      shift-left: w528 -> [w548]
                      i -> [w544]
                      n147 = Number To Decimal String(number=w544) -> (decimal integer string=w543:string)  [unwired: 1 in]
                      n148 = stacked-sequence {
                        seq-local: [_ w560 _ _ _ _] -> [_ _ w564 _ _ _]
                        seq-local: [_ _ w563 _ _ _] -> [_ _ _ w570 _ _]
                        seq-local: [w556 _ _ _ _ _] -> [_ w559 _ _ _ _]
                        seq-local: [_ _ _ w576 _ _] -> [_ _ _ _ w596 _]
                        seq-local: [_ _ _ _ w595 _] -> [_ _ _ _ _ w598]
                        tunnel: w548 -> [w557 _ _ _ _ _]
                        tunnel: w550 -> [w558 _ _ w573 w592 _]
                        tunnel: w549 -> [_ _ _ _ w597 _]
                        tunnel: w547 -> [_ _ _ _ _ w603]
                        tunnel: [_ _ _ _ _ w602] -> w546
                        tunnel: w545 -> [_ _ _ _ _ w601]
                        tunnel: w543 -> [_ _ _ w571 w593 _]
                        frame #0 {
                          # "Set Spool"
                          n149 = Wait (ms)(milliseconds to wait=u32 100) -> ()  [unwired: 1 out]
                          n150 = call <userlib>:"SetSpool.vi"("active"=TRUE, "method"=2, "name"=w558, "framebuffersize (10)"=20, "error in (no error)"=w557) -> ("DLL error code"=w551:u32, "error out"=w556:errorcluster)  [unwired: 9 in]
                          n151 = local write "Return from SetSpool"(w551) -> ()
                        }
                        frame #1 {
                          w561 = 20002  # DRV_SUCCESS
                          n152 = call <userlib>:"StartAcquisition.vi"("error in (no error)"=w559) -> ("error out"=w560:errorcluster, "DLL error code"=w562:u32)  [unwired: 1 in]
                          n153 = Equal?(x=w561, y=w562) -> ()  [unwired: 1 out]
                        }
                        frame #2 {
                          n154 = while {
                            tunnel: w564 -> [w566]
                            tunnel: [w565] -> w563
                            stop <- w567 continue-if-true
                            w569 = u16 72  # DRV ACQUIRING
                            n155 = call <userlib>:"GetStatus.vi"("error in (no error)"=w566) -> ("error out"=w565:errorcluster, "status"=w568:T20)  [unwired: 2 in, 1 out]
                            n156 = Equal?(x=w568, y=w569) -> (x = y?=w567:bool)
                          }
                        }
                        frame #3 {
                          # "Save acquisition"
                          n157 = local read "File Type"() -> (w575:enum16{"TIFF", "Sif"})
                          n158 = Concatenate Strings(w573, "_", w571) -> (w574:string)
                          n159 = case shown="\"TIFF\", Default" w575 {
                            tunnel: "C:\\Program Files\\Andor SOLIS\\GREY.PAL" -> [w581 _]
                            tunnel: w574 -> [w584 w590]
                            tunnel: w570 -> [w582 w587]
                            tunnel: [w583 w586] -> w576
                            frame "TIFF", Default {
                              w578 = 1
                              n160 = Concatenate Strings(w584, ".tif") -> (w580:string)
                              n161 = call <userlib>:"SaveAsTiffEx.vi"("path"=w580, "palette"=w581, "position"=0, "type"=w578, "mode"=w578, "error in (no error)"=w582) -> ("error out"=w583:errorcluster)  [unwired: 12 in, 1 out]
                            }
                            frame "Sif" {
                              n162 = Concatenate Strings(w590, ".sif") -> (w588:string)
                              n163 = call <userlib>:"SaveAsSif.vi"("error in (no error)"=w587, "path"=w588) -> ("error out"=w586:errorcluster)  [unwired: 1 out]
                            }
                          }
                        }
                        frame #4 {
                          # "Clearn Spool Files"
                          n164 = Concatenate Strings(w592, "_", w593) -> (w594:string)
                          n165 = call "cleanSpool.vi"("error in (no error)"=w596, "Total Img Num"=w597, "strPath"=w594) -> ("error out"=w595:errorcluster)  [unwired: 8 in]
                        }
                        frame #5 {
                          n166 = Wait (ms)(milliseconds to wait=u32 100) -> ()  [unwired: 1 out]
                          n167 = Number To Fractional String(number=w601, precision (6)=1) -> (F-format string=w606:string)  [unwired: 2 in]
                          n168 = Concatenate Strings("movrel z=", w606) -> (w604:string)
                          n169 = call "WriteCmd.vi"("Command"=w604, "VISA resource name"=w603) -> ("error"=w602:errorcluster)  [unwired: 1 in]
                          n170 = local write "Current error"(w598) -> ()
                        }
                      }
                    }
                    n171 = stacked-sequence {
                      seq-local: [_ w610 _] -> [_ _ w626]
                      tunnel: [_ _ w625] -> w541
                      tunnel: w530 -> [_ w614 _]
                      tunnel: w529 -> [_ w617 _]
                      tunnel: w525 -> [_ w615 _]
                      tunnel: "Current Z as Center" -> [_ w612 _]
                      tunnel: w519 -> [_ w611 _]
                      tunnel: w522 -> [_ _ w624]
                      tunnel: w521 -> [_ _ w623]
                      frame #0 {
                        n172 = local write "EMCCD Status"(FALSE) -> ()
                        n173 = local write "Running Status"(0) -> ()
                      }
                      frame #1 {
                        n174 = case shown="True" w612 {
                          tunnel: w614 -> [w621 _]
                          tunnel: [w621 w622] -> w613
                          tunnel: w611 -> [_ w622]
                          frame False {
                          }
                          frame True {
                          }
                        }
                        n175 = Negate(x=w613) -> (-x=w616:dbl)
                        n176 = Number To Fractional String(number=w616, precision (6)=1) -> (F-format string=w619:string)  [unwired: 2 in]
                        n177 = Concatenate Strings("movrel z=", w619) -> (w620:string)
                        n178 = call "WriteCmd.vi"("error IO"=w615, "Command"=w620, "VISA resource name"=w617) -> ("error"=w610:errorcluster)
                      }
                      frame #2 {
                        # "Turn off laser"
                        n179 = invoke class="MG17Motor" method="SC_Disable"(reference=w623, error in=w626, "lChanID"=w624) -> (error out=w625:errorcluster)  [unwired: 1 in, 3 out]
                      }
                    }
                  }
                }
              }
            }
          }
          frame True {
            # "Acqure Wavefront Images"
            n180 = local read "HASO ready"() -> (w662:bool)
            n181 = And(x=w661, y=w662) -> (x .and. y?=w663:bool)
            n182 = case shown="True" w663 {
              tunnel: w679 -> [_ w709]
              tunnel: w678 -> [_ w708]
              tunnel: w677 -> [_ w707]
              tunnel: [w680 w704] -> w676
              tunnel: w675 -> [_ w701]
              tunnel: [w685 w700] -> w674
              tunnel: w673 -> [w685 w686]
              tunnel: w672 -> [w680 w687]
              tunnel: w671 -> [w683 w699]
              tunnel: w670 -> [w682 w698]
              tunnel: [w683 w697] -> w669
              tunnel: [w682 w696] -> w668
              tunnel: w667 -> [w684 w695]
              tunnel: w666 -> [w681 w694]
              tunnel: [w684 w693] -> w665
              tunnel: [w681 w692] -> w664
              frame False {
              }
              frame True {
                n183 = property on="nb_images (set)" class="DigNum (strict)"() -> ("Value"=w710:u32)  [unwired: 2 in, 2 out]
                n184 = case shown="1" w710 {
                  tunnel: [w761 w763] -> w711
                  tunnel: w701 -> [w760 _]
                  tunnel: w709 -> [w761 _]
                  tunnel: [w760 w762] -> w706
                  tunnel: w708 -> [_ w763]
                  tunnel: w707 -> [_ w762]
                  frame 2, Default {
                  }
                  frame 1 {
                  }
                }
                n185 = while {
                  tunnel: w686 -> [w716]
                  tunnel: [w715] -> w688
                  tunnel: w687 -> [w713]
                  tunnel: [w712] -> w689
                  stop <- w714 stop-if-true
                  n186 = call <userlib>:"LVClass_Camera asynchroneImageReady.vi"("Camera in"=w716, "error in (no error)"=w713) -> ("Camera out"=w715:refnum<class "Camera.lvclass">, "ready"=w714:bool, "error out"=w712:errorcluster)  [unwired: 11 in]
                }
                n187 = call <userlib>:"LVClass_Camera get image.vi"("Camera in"=w688, "Image"=w711, "Image RAW"=w706, "remove_background"=FALSE, "error in (no error)"=w689) -> ("Camera out"=w700:refnum<class "Camera.lvclass">, "Image (dup)"=w705:refnum<class "Image.lvclass">, "error out"=w702:errorcluster)  [unwired: 7 in, 1 out]
                n188 = case shown="No Error" w702 {
                  selector: w702 -> [w757 w758]
                  tunnel: w705 -> [w754 w759]
                  tunnel: [w752 w759] -> w691
                  tunnel: [w751 w758] -> w690
                  frame No Error {
                    # "get image"
                    n189 = call <userlib>:"LVClass_Image get image data.vi"("Image in"=w754, "error in (no error)"=w757) -> ("Image out"=w756:refnum<class "Image.lvclass">, "Image data out"=w750:u32[][], "error out"=w755:errorcluster)  [unwired: 11 in]
                    n190 = call <userlib>:"LVClass_Image get image information.vi"("Image in"=w756, "error in (no error)"=w755) -> ("Image out"=w752:refnum<class "Image.lvclass">, "Acquisition information"=→"Acquisition information":T9, "error out"=w751:errorcluster)  [unwired: 11 in]
                    n191 = local write "HASO intensity"(w750) -> ()
                  }
                  frame Error {
                  }
                }
                n192 = case shown="No Error" w690 {
                  selector: w690 -> [w737 w749]
                  tunnel: [w743 w749] -> w704
                  tunnel: w691 -> [w736 _]
                  tunnel: [w741 w745] -> w692
                  tunnel: [w740 w748] -> w693
                  tunnel: w699 -> [w733 w747]
                  tunnel: w698 -> [w732 w746]
                  tunnel: [w721 w747] -> w697
                  tunnel: [w731 w746] -> w696
                  tunnel: w695 -> [w729 w748]
                  tunnel: w694 -> [w727 w745]
                  frame No Error {
                    # "phaseout"
                    n193 = call "image2slopes.vi"("error in (no error)"=w737, "Image in"=w736, "HasoEngine in"=w732, "HasoSlopes in"=w733) -> ("error out"=w730:errorcluster, "HasoEngine out"=w731:refnum<class "HasoEngine.lvclass">, "HasoSlopes out"=w723:refnum<class "HasoSlopes.lvclass">)  [unwired: 4 in, 1 out]
                    n194 = local read "Filter"() -> (w726:u8[])
                    n195 = call "slopes2phase.vi"("TypePhase"=WavefrontReconstructionMode."Modal_Zernike", "Number of coefficients"=u8 32, "error in (no error)"=w730, "Filter"=w726, "HasoSlopes in"=w723, "Phase in"=w729) -> ("error out"=w720:errorcluster, "HasoSlopes out"=w722:refnum<class "HasoSlopes.lvclass">, "Phase out"=w728:refnum<class "Phase.lvclass">)  [unwired: 3 in]
                    n196 = local read "idxType"() -> (w717:enum16{"Wyant", "ANSI"})
                    n197 = call "slopes2zern.vi"("HasoSlopes in"=w722, "error in (no error)"=w720, "idxType"=w717) -> ("HasoSlopes out"=w721:refnum<class "HasoSlopes.lvclass">, "Zernike Coefficients"=w718:dbl[], "error out"=w719:errorcluster)  [unwired: 3 in, 2 out]
                    n198 = call <userlib>:"LVClass_Pupil ctor from HasoSlopes.vi"("Pupil in"=w727, "HasoSlopes.lvclass"=w723, "error in (no error)"=w719) -> ("Pupil out"=w738:refnum<class "Pupil.lvclass">, "error out"=w739:errorcluster)  [unwired: 11 in]
                    n199 = call <userlib>:"LVClasse_Phase GetStatisticDatas.vi"("Phase in"=w728, "error in (no error)"=w739) -> ("Phase out"=w744:refnum<class "Phase.lvclass">, "StatisticsData"=w724:T2, "error out"=w742:errorcluster)  [unwired: 11 in]
                    n200 = local write "Phase statistics"(w724) -> ()
                    n201 = call <userlib>:"LVClasse_Phase Get Data.vi"("Phase in"=w744, "Pupil"=w738, "error in (no error)"=w742) -> ("Phase out"=w740:refnum<class "Phase.lvclass">, "data"=w725:sgl[][], "Pupil (dup)"=w741:refnum<class "Pupil.lvclass">, "error out"=w743:errorcluster)  [unwired: 9 in]
                    n202 = local write "Zernike Measured"(w718) -> ()
                    n203 = local write "Phase values"(w725) -> ()
                  }
                  frame Error {
                  }
                }
              }
            }
          }
        }
        "Current error" <- w379
        n204 = Unbundle By Name(w379) -> ("status"=w378:bool)
      }
      event "nb_images (set)": Value Change {
        # "SET IMAGE NUMBER"
        n205 = event-data() -> ("NewVal"=w781:u32)  [unwired: 1 in]
        n206 = call <userlib>:"LVClass_Camera set nbImagesToSum.vi"("Camera in"=w779, "nb_image"=w781, "error in (no error)"=w780) -> ("Camera out"=w776:refnum<class "Camera.lvclass">, "error out"=w775:errorcluster)  [unwired: 11 in]
        n207 = call <userlib>:"LVClass_Camera get nbImagesToSum.vi"("Camera in"=w776, "error in (no error)"=w775) -> ("Camera out"=w777:refnum<class "Camera.lvclass">, "nb_image"=→"nb_images (get)":u32, "error out"=w778:errorcluster)  [unwired: 11 in]
      }
      event "Coef Min": Value Change {
        # "Set coeff display scale: min"
        n208 = event-data() -> ()  [unwired: 1 in, 1 out]
        n209 = local read "Coef Min"() -> (w782:dbl)
        n210 = property on="Zernike Measured" class="WFGraph (strict)"("YScale.Minimum"=w782) -> ()  [unwired: 2 in, 2 out]
      }
      event "Coef Max": Value Change {
        # "Set coeff display scale: min"
        n211 = event-data() -> ()  [unwired: 1 in, 1 out]
        n212 = local read "Coef Max"() -> (w795:dbl)
        n213 = property on="Zernike Measured" class="WFGraph (strict)"("YScale.Maximum"=w795) -> ()  [unwired: 2 in, 2 out]
      }
      event "Reset error": Mouse Up {
        n214 = event-data() -> ()  [unwired: 1 in, 8 out]
        n215 = Select(t=w813, s=w813, f=errorcluster {"status"=FALSE, "code"=0, "source"=""} ("error out")) -> (s? t:f=w814:errorcluster)
      }
      event "exposure_duration_s (set)": Value Change {
        # "CHANGE EXPOSURE DURATION"
        n216 = event-data() -> ()  [unwired: 1 in, 1 out]
        n217 = Multiply(x=1000000.0, y="exposure_duration_s (set)") -> (x*y=w829:dbl)
        n218 = To Unsigned Long Integer(number=w829) -> (unsigned 32bit integer=w828:u32)
        n219 = call <userlib>:"LVClass_Camera set Parameter Int.vi"("Camera in"=w842, "parameter_name"="exposure_duration_us", "value"=w828, "error in (no error)"=w843) -> ("Camera out"=w841:refnum<class "Camera.lvclass">, "error out"=w840:errorcluster)  [unwired: 10 in]
        n220 = call <userlib>:"LVClass_Camera get Parameter Int.vi"("Camera in"=w841, "parameter_name"="exposure_duration_us", "error in (no error)"=w840) -> ("Camera out"=w839:refnum<class "Camera.lvclass">, "value"=→"exposure_duration_us (get)":i32, "error out"=w838:errorcluster)  [unwired: 10 in]
      }
      event "Start HASO": Mouse Up {
        # "Start acquisition in SYNCRHONOUS mode\n\nonly one acquisition mode is available :\nLast image"
        n221 = event-data() -> ()  [unwired: 1 in, 8 out]
        n222 = flat-sequence {
          tunnel: w860 -> [w866]
          tunnel: w859 -> [w865]
          tunnel: [w864] -> w846
          tunnel: [w863] -> w845
          tunnel: [w868] -> w857
          tunnel: [w869] -> w858
          tunnel: w846 -> [w869]
          tunnel: w845 -> [w868]
          frame #0 {
            n223 = call <userlib>:"LVClass_Camera start acquisition.vi"("Camera in"=w866, "synchronisation_mode"=enum16{"synchronous", "asynchronous"}."asynchronous", "acquisition_mode"=enum16{"last_image", "new_image"}."last_image", "error in (no error)"=w865) -> ("Camera out"=w864:refnum<class "Camera.lvclass">, "error out"=w863:errorcluster)  [unwired: 10 in]
          }
          frame #1 {
            n224 = local write "HASO ready"(TRUE) -> ()
          }
        }
      }
      event "Stop HASO": Mouse Up {
        n225 = event-data() -> ()  [unwired: 1 in, 8 out]
        n226 = flat-sequence {
          tunnel: w884 -> [w888]
          tunnel: w877 -> [w886]
          tunnel: [w889] -> w871
          tunnel: [w887] -> w870
          tunnel: [w891] -> w883
          tunnel: [w892] -> w885
          tunnel: w871 -> [w892]
          tunnel: w870 -> [w891]
          frame #0 {
            n227 = call <userlib>:"LVClass_Camera stop acquisition.vi"("Camera in"=w888, "error in (no error)"=w886) -> ("Camera out"=w889:refnum<class "Camera.lvclass">, "error out"=w887:errorcluster)  [unwired: 12 in]
          }
          frame #1 {
            n228 = local write "HASO ready"(FALSE) -> ()
          }
        }
      }
      event "Update DM": Mouse Up {
        n229 = event-data() -> ()  [unwired: 1 in, 8 out]
        n230 = local read "Initial offset"() -> (w902:bool)
        n231 = case shown="True" w902 {
          tunnel: [w917 w922] -> w907
          frame False {
            n232 = Initialize Array(0.0, 52) -> (w917:dbl[])
          }
          frame True {
            n233 = local read "Offset command file"() -> (w921:path)
            n234 = call-poly <vilib>:"Read From Spreadsheet File.vi"("format (%.3f)"="%.8f", "file path (dialog if empty)"=w921) -> ("first row"=w922:dbl[])  [unwired: 5 in, 4 out]
          }
        }
        n235 = local read "Additional Command"() -> (w912:bool)
        n236 = case shown="True" w912 {
          tunnel: [w924 w930] -> w908
          tunnel: [w923 w929] -> w909
          tunnel: w905 -> [w923 w928]
          frame False {
            n237 = Initialize Array(0.0, 52) -> (w924:dbl[])
          }
          frame True {
            n238 = local read "Input type"() -> (w927:T8)
            n239 = case shown="\"DM actuators\"" w927 {
              tunnel: w928 -> [w931 w936 w979 w993 w1002]
              tunnel: [w932 w938 w980 w991 w1004] -> w930
              tunnel: [w931 w935 w979 w990 w1001] -> w929
              frame "Zero Input" {
                n240 = Initialize Array(0.0, 52) -> (w932:dbl[])
              }
              frame "DM actuators" {
                w942 = 1
                w943 = 52
                n241 = local read "Zern/DM index in"() -> (w939:i32[])
                n242 = local read "Zern/DM coef in"() -> (w937:sgl[])
                n243 = Array Size(array=w939) -> (size(s)=w947:i32)
                n244 = Initialize Array(0.0, w943) -> (w945:dbl[])
                n245 = call-poly <vilib>:"Ramp Pattern.vi"("start"=w942, "end"=w943, "delta"=w942) -> ("Ramp Pattern"=w944:dbl[])  [unwired: 6 in, 2 out]
                n246 = Less Or Equal?(x=w947, y=w943) -> (x <= y?=w946:bool)
                n247 = case shown="True" w946 {
                  tunnel: w947 -> [_ w958]
                  tunnel: w945 -> [w951 w957]
                  tunnel: [w951 w956] -> w938
                  tunnel: w939 -> [_ w955]
                  tunnel: w937 -> [_ w954]
                  tunnel: [w948 w952] -> w935
                  tunnel: w943 -> [_ w953]
                  tunnel: w936 -> [w950 w952]
                  frame False {
                    n248 = Merge Errors(w950, errorcluster {"status"=FALSE, "code"=0, "source"="Wrong Zern index size"} ("error out")) -> (w948:errorcluster)
                  }
                  frame True {
                    n249 = for {
                      N: w958 -> [_]
                      shift-right: [w971] -> w956
                      shift-left: w957 -> [w972]
                      tunnel: w955 -> [w968] mode=indexing
                      tunnel: w954 -> [w962] mode=indexing
                      tunnel: w953 -> [w969]
                      n250 = Greater Than 0?(x=w968) -> (x > 0?=w967:bool)
                      n251 = Less Or Equal?(x=w968, y=w969) -> (x <= y?=w959:bool)
                      n252 = And(x=w967, y=w959) -> (x .and. y?=w966:bool)
                      n253 = In Range and Coerce(upper limit=0.8, x=w962, lower limit=-0.8) -> (coerced(x)=w963:dbl, In Range?=w965:bool)
                      n254 = And(x=w966, y=w965) -> (x .and. y?=w964:bool)
                      n255 = Decrement(x=w968) -> (x-1=w970:i32)
                      n256 = case shown="True" w964 {
                        tunnel: w970 -> [_ w977]
                        tunnel: w972 -> [w973 w976]
                        tunnel: [w973 w975] -> w971
                        tunnel: w963 -> [_ w974]
                        frame False {
                        }
                        frame True {
                          n257 = Replace Array Subset(array=w976, new element=w974, index=w977) -> (w975:dbl[])
                        }
                      }
                    }
                  }
                }
                n258 = local write "Coef out"(w938) -> ()
                n259 = To Long Integer(number=w944) -> (32bit integer=w940:i32[])
                n260 = local write "Index out"(w940) -> ()
              }
              frame "Command File" {
                n261 = local read "Additional file"() -> (w978:path)
                n262 = call-poly <vilib>:"Read From Spreadsheet File.vi"("format (%.3f)"="%.8f", "file path (dialog if empty)"=w978) -> ("first row"=w980:dbl[])  [unwired: 5 in, 4 out]
              }
              frame "Zernike Coef", Default {
                n263 = local read "Zern/DM index in"() -> (w982:i32[])
                n264 = local read "Zern/DM coef in"() -> (w983:sgl[])
                n265 = local read "idxType"() -> (w989:enum16{"Wyant", "ANSI"})
                n266 = local read "Initial haso file"() -> (w987:path)
                n267 = local read "Haso configuration file"() -> (w988:path)
                n268 = local read "interaction matrix file"() -> (w986:path)
                n269 = call "zern2command.vi"("Haso configuration file"=w988, "idxType"=w989, "interaction matrix file"=w986, "error in (no error)"=w993, "Zern coef in"=w983, "Zern index in"=w982, "Initial haso file"=w987) -> ("error out"=w992:errorcluster, "Offset Positions"=w991:sgl[], "Zern pupil out"=w994:refnum<class "Pupil.lvclass">, "ModalCoef out"=w995:refnum<class "ModalCoef.lvclass">)  [unwired: 1 in]
                n270 = call <userlib>:"LVClass_ModalCoef GetData.vi"("ModalCoef in"=w995, "Pupil.lvclass"=w994, "error in (no error)"=w992) -> ("ModalCoef out"=w999:refnum<class "ModalCoef.lvclass">, "coef"=w985:sgl[], "index"=w984:u32[], "Pupil.lvclass (dup)"=w998:refnum<class "Pupil.lvclass">, "error out"=w997:errorcluster)  [unwired: 8 in]
                n271 = local write "Index out"(w984) -> ()
                n272 = call <userlib>:"LVClass_Pupil dtor.vi"("Pupil in"=w998, "error in (no error)"=w997) -> ("error out"=w996:errorcluster)  [unwired: 12 in, 1 out]
                n273 = local write "Coef out"(w985) -> ()
                n274 = call <userlib>:"LVClass_ModalCoef dtor.vi"("ModalCoef in"=w999, "error in (no error)"=w996) -> ("error out"=w990:errorcluster)  [unwired: 12 in, 1 out]
              }
              frame "Zernike File" {
                w1007 = 1
                n275 = local read "interaction matrix file"() -> (w1011:path)
                n276 = local read "Initial haso file"() -> (w1009:path)
                n277 = local read "Haso configuration file"() -> (w1010:path)
                n278 = local read "Additional file"() -> (w1020:path)
                n279 = call-poly <vilib>:"Ramp Pattern.vi"("start"=w1007, "end"=32, "delta"=w1007) -> ("Ramp Pattern"=w1008:dbl[])  [unwired: 6 in, 2 out]
                n280 = To Long Integer(number=w1008) -> (32bit integer=w1005:i32[])
                n281 = local read "idxType"() -> (w1000:enum16{"Wyant", "ANSI"})
                n282 = call-poly <vilib>:"Read From Spreadsheet File.vi"("format (%.3f)"="%.8f", "file path (dialog if empty)"=w1020) -> ("first row"=w1012:dbl[])  [unwired: 5 in, 4 out]
                n283 = call "zern2command.vi"("Haso configuration file"=w1010, "idxType"=w1000, "interaction matrix file"=w1011, "Zern coef in"=w1012, "Zern index in"=w1005, "Initial haso file"=w1009) -> ("error out"=w1013:errorcluster, "Offset Positions"=w1004:sgl[], "Zern pupil out"=w1014:refnum<class "Pupil.lvclass">, "ModalCoef out"=w1015:refnum<class "ModalCoef.lvclass">)  [unwired: 2 in]
                n284 = call <userlib>:"LVClass_ModalCoef GetData.vi"("ModalCoef in"=w1015, "Pupil.lvclass"=w1014, "error in (no error)"=w1013) -> ("ModalCoef out"=w1019:refnum<class "ModalCoef.lvclass">, "Pupil.lvclass (dup)"=w1018:refnum<class "Pupil.lvclass">, "error out"=w1017:errorcluster)  [unwired: 8 in, 2 out]
                n285 = call <userlib>:"LVClass_Pupil dtor.vi"("Pupil in"=w1018, "error in (no error)"=w1017) -> ("error out"=w1016:errorcluster)  [unwired: 12 in, 1 out]
                n286 = call <userlib>:"LVClass_ModalCoef dtor.vi"("ModalCoef in"=w1019, "error in (no error)"=w1016) -> ("error out"=w1003:errorcluster)  [unwired: 12 in, 1 out]
                n287 = Merge Errors(w1003, w1002) -> (w1001:errorcluster)
              }
            }
          }
        }
        n288 = local write "Initial Positions"(w907) -> ()
        n289 = Add(x=w908, y=w907) -> (x+y=w893:dbl[])
        n290 = call <userlib>:"LVClass_WavefrontCorrector Move to Absolute Position.vi"("WavefrontCorrector in"=w903, "Absolute Positions"=w893, "error in (no error)"=w909) -> ("WavefrontCorrector out"=w910:refnum<class "WavefrontCorrector.lvclass">, "error out"=w911:errorcluster)  [unwired: 11 in]
        n291 = call <userlib>:"LVClass_WavefrontCorrector Get Current Position.vi"("WavefrontCorrector in"=w910, "error in (no error)"=w911) -> ("WavefrontCorrector out"=w899:refnum<class "WavefrontCorrector.lvclass">, "Wavefront Corrector Position"=w894:T18, "error out"=w904:errorcluster)  [unwired: 11 in]
        n292 = local write "Final Positions"(w893) -> ()
        n293 = local write "DM Actuator Values"(w894) -> ()
        n294 = Unbundle By Name(w904) -> ("status"=w906:bool)
      }
      event "Update AcqSetting": Mouse Up {
        n295 = event-data() -> ()  [unwired: 1 in, 8 out]
        n296 = local read "Gain On"() -> (w1041:bool)
        n297 = local read "Aquisition Mode"() -> (w1032:T6)
        n298 = local read "Accum Num"() -> (w1031:u32)
        n299 = To Unsigned Word Integer(number=w1032) -> (unsigned 16bit integer=w1026:u16)
        n300 = local read "Kinetic Num"() -> (w1043:u32)
        n301 = local read "Trigger Mode"() -> (w1033:enum16{"Internal", "External"})
        n302 = call <userlib>:"SetAcquisitionMode.vi"("error in (no error)"=w1025, "mode"=w1026) -> ("error out"=w1027:errorcluster)  [unwired: 1 out]
        n303 = To Unsigned Word Integer(number=w1033) -> (unsigned 16bit integer=w1028:u16)
        n304 = local read "Exposure time (s)"() -> (w1034:dbl)
        n305 = call <userlib>:"SetTriggerMode.vi"("error in (no error)"=w1027, "mode"=w1028) -> ("error out"=w1029:errorcluster)  [unwired: 1 out]
        n306 = call <userlib>:"SetExposureTime.vi"("error in (no error)"=w1029, "time"=w1034) -> ("error out"=w1030:errorcluster)  [unwired: 1 out]
        n307 = case shown="\"None\", Default" w1032 {
          tunnel: w1031 -> [_ _ w1061 w1066]
          tunnel: w1030 -> [w1057 w1058 w1060 w1065]
          tunnel: [w1057 w1058 w1059 w1063] -> w1044
          tunnel: w1043 -> [_ _ _ w1062]
          frame "None", Default {
          }
          frame "Single Scan" {
          }
          frame "Accumulate" {
            n308 = call <userlib>:"SetNumberAccumulations.vi"("error in (no error)"=w1060, "number"=w1061) -> ("error out"=w1059:errorcluster)  [unwired: 1 out]
          }
          frame "Kinetics" {
            n309 = call <userlib>:"SetNumberAccumulations.vi"("error in (no error)"=w1065, "number"=w1066) -> ("error out"=w1064:errorcluster)  [unwired: 1 out]
            n310 = call <userlib>:"SetNumberKinetics.vi"("error in (no error)"=w1064, "number"=w1062) -> ("error out"=w1063:errorcluster)  [unwired: 1 out]
          }
        }
        n311 = case shown="False" w1041 {
          tunnel: w1044 -> [w1050 w1056]
          tunnel: [w1049 w1053] -> w1042
          frame False {
            n312 = call <userlib>:"SetEMCCDGain.vi"("error in (no error)"=w1050, "gain"=0) -> ("error out"=w1049:errorcluster)  [unwired: 1 out]
          }
          frame True {
            # "0-255"
            n313 = call <userlib>:"SetEMGainMode.vi"("error in (no error)"=w1056, "mode"=0) -> ("error out"=w1054:errorcluster)  [unwired: 1 out]
            n314 = local read "Gain Value"() -> (w1052:sgl)
            n315 = call <userlib>:"SetEMCCDGain.vi"("error in (no error)"=w1054, "gain"=w1052) -> ("error out"=w1053:errorcluster)  [unwired: 1 out]
          }
        }
        n316 = call <userlib>:"GetEMCCDGain.vi"("error in (no error)"=w1042) -> ("error out"=w1039:errorcluster, "gain"=w1040:u32)  [unwired: 2 in, 1 out]
        n317 = local write "Get EMCCD Gain"(w1040) -> ()
        n318 = call <userlib>:"GetAcquisitionTimings.vi"("error in (no error)"=w1039) -> ("exposure"=w1035:sgl, "accumulate"=w1037:sgl, "kinetic"=w1038:sgl, "DLL error code"=w1036:u32, "error out"=w1024:errorcluster)  [unwired: 10 in]
        n319 = local write "Return from CheckTimings"(w1036) -> ()
        n320 = local write "Get Exposure Time"(w1035) -> ()
        n321 = local write "Get Kinetic Time"(w1038) -> ()
        n322 = local write "Get Accum Time"(w1037) -> ()
      }
      event "Update FOV": Mouse Up {
        n323 = event-data() -> ()  [unwired: 1 in, 8 out]
        n324 = local read "Detector Y Pixels"() -> (w1069:i32)
        n325 = local read "Detector X Pixels"() -> (w1088:i32)
        n326 = local read "Camera FOV"() -> (w1087:T5)
        n327 = case shown="\"Custom FOV\"" w1087 {
          tunnel: [w1100 w1124 w1140 w1156 w1172 w1175] -> w1073
          tunnel: [w1099 w1124 w1140 w1156 w1172 w1175] -> w1072
          tunnel: [w1098 w1114 w1130 w1146 w1162 w1175] -> w1071
          tunnel: [w1097 w1111 w1127 w1143 w1159 w1173] -> w1070
          tunnel: [w1095 w1113 w1129 w1145 w1161 w1175] -> w1074
          tunnel: [w1096 w1110 w1126 w1142 w1158 w1174] -> w1075
          tunnel: w1088 -> [_ w1123 w1139 w1155 w1171 w1173]
          tunnel: w1069 -> [_ w1122 w1138 w1154 w1170 w1174]
          tunnel: [w1101 w1109 w1125 w1141 w1157 w1174] -> w1077
          tunnel: [w1103 w1109 w1125 w1141 w1157 w1173] -> w1076
          frame "Custom FOV" {
            n328 = local read "Xstart"() -> (w1098:i32)
            n329 = local read "Xend"() -> (w1097:i32)
            n330 = local read "Xstart"() -> (w1095:i32)
            n331 = local read "Yend"() -> (w1096:i32)
            n332 = Subtract(x=w1096, y=w1095) -> (x-y=w1107:i32)
            n333 = Subtract(x=w1097, y=w1098) -> (x-y=w1108:i32)
            n334 = local read "Xbin"() -> (w1100:i32)
            n335 = local read "Ybin"() -> (w1099:i32)
            n336 = Increment(x=w1107) -> (x+1=w1106:i32)
            n337 = Increment(x=w1108) -> (x+1=w1105:i32)
            n338 = Divide(x=w1106, y=w1099) -> (x/y=w1102:dbl)
            n339 = Divide(x=w1105, y=w1100) -> (x/y=w1104:dbl)
            n340 = To Long Integer(number=w1102) -> (32bit integer=w1101:i32)
            n341 = To Long Integer(number=w1104) -> (32bit integer=w1103:i32)
          }
          frame "FOV: 768x768" {
            w1109 = 768
            w1119 = 2.0
            w1124 = 1
            n342 = Subtract(x=w1123, y=w1109) -> (x-y=w1121:i32)
            n343 = Subtract(x=w1122, y=w1109) -> (x-y=w1120:i32)
            n344 = Divide(x=w1120, y=w1119) -> (x/y=w1117:dbl)
            n345 = Divide(x=w1121, y=w1119) -> (x/y=w1118:dbl)
            n346 = Decrement(x=w1109) -> (x-1=w1112:i32)
            n347 = Round To Nearest(number=w1118) -> (nearest integer value=w1116:dbl)
            n348 = Round To Nearest(number=w1117) -> (nearest integer value=w1115:dbl)
            n349 = To Long Integer(number=w1116) -> (32bit integer=w1114:i32)
            n350 = To Long Integer(number=w1115) -> (32bit integer=w1113:i32)
            n351 = Add(x=w1112, y=w1114) -> (x+y=w1111:i32)
            n352 = Add(x=w1112, y=w1113) -> (x+y=w1110:i32)
          }
          frame "FOV: 512x512" {
            w1125 = 512
            w1135 = 2.0
            w1140 = 1
            n353 = Subtract(x=w1139, y=w1125) -> (x-y=w1137:i32)
            n354 = Subtract(x=w1138, y=w1125) -> (x-y=w1136:i32)
            n355 = Divide(x=w1136, y=w1135) -> (x/y=w1133:dbl)
            n356 = Divide(x=w1137, y=w1135) -> (x/y=w1134:dbl)
            n357 = Decrement(x=w1125) -> (x-1=w1128:i32)
            n358 = Round To Nearest(number=w1134) -> (nearest integer value=w1132:dbl)
            n359 = Round To Nearest(number=w1133) -> (nearest integer value=w1131:dbl)
            n360 = To Long Integer(number=w1132) -> (32bit integer=w1130:i32)
            n361 = To Long Integer(number=w1131) -> (32bit integer=w1129:i32)
            n362 = Add(x=w1128, y=w1130) -> (x+y=w1127:i32)
            n363 = Add(x=w1128, y=w1129) -> (x+y=w1126:i32)
          }
          frame "FOV: 320x320" {
            w1141 = 320
            w1151 = 2.0
            w1156 = 1
            n364 = Subtract(x=w1155, y=w1141) -> (x-y=w1153:i32)
            n365 = Subtract(x=w1154, y=w1141) -> (x-y=w1152:i32)
            n366 = Divide(x=w1152, y=w1151) -> (x/y=w1149:dbl)
            n367 = Divide(x=w1153, y=w1151) -> (x/y=w1150:dbl)
            n368 = Decrement(x=w1141) -> (x-1=w1144:i32)
            n369 = Round To Nearest(number=w1150) -> (nearest integer value=w1148:dbl)
            n370 = Round To Nearest(number=w1149) -> (nearest integer value=w1147:dbl)
            n371 = To Long Integer(number=w1148) -> (32bit integer=w1146:i32)
            n372 = To Long Integer(number=w1147) -> (32bit integer=w1145:i32)
            n373 = Add(x=w1144, y=w1146) -> (x+y=w1143:i32)
            n374 = Add(x=w1144, y=w1145) -> (x+y=w1142:i32)
          }
          frame "FOV: 256x256" {
            w1157 = 256
            w1167 = 2.0
            w1172 = 1
            n375 = Subtract(x=w1171, y=w1157) -> (x-y=w1169:i32)
            n376 = Subtract(x=w1170, y=w1157) -> (x-y=w1168:i32)
            n377 = Divide(x=w1168, y=w1167) -> (x/y=w1165:dbl)
            n378 = Divide(x=w1169, y=w1167) -> (x/y=w1166:dbl)
            n379 = Decrement(x=w1157) -> (x-1=w1160:i32)
            n380 = Round To Nearest(number=w1166) -> (nearest integer value=w1164:dbl)
            n381 = Round To Nearest(number=w1165) -> (nearest integer value=w1163:dbl)
            n382 = To Long Integer(number=w1164) -> (32bit integer=w1162:i32)
            n383 = To Long Integer(number=w1163) -> (32bit integer=w1161:i32)
            n384 = Add(x=w1160, y=w1162) -> (x+y=w1159:i32)
            n385 = Add(x=w1160, y=w1161) -> (x+y=w1158:i32)
          }
          frame "Full FOV", Default {
            w1175 = 1
          }
        }
        n386 = local write "FOV X Pixels"(w1076) -> ()
        n387 = local write "FOV Y Pixels"(w1077) -> ()
        n388 = call <userlib>:"SetImage.vi"("hbin"=w1073, "vbin"=w1072, "hstart"=w1071, "hend"=w1070, "vstart"=w1074, "vend"=w1075, "error in (no error)"=w1067) -> ("error out"=w1078:errorcluster)  [unwired: 19 in, 1 out]
        n389 = call <userlib>:"GetAcquisitionTimings.vi"("error in (no error)"=w1078) -> ("exposure"=w1080:sgl, "accumulate"=w1081:sgl, "kinetic"=w1082:sgl, "DLL error code"=w1083:u32, "error out"=w1079:errorcluster)  [unwired: 10 in]
        n390 = call <userlib>:"GetAcquisitionProgress.vi"("error in (no error)"=w1079) -> ("error out"=w1068:errorcluster, "DLL error code"=w1086:u32, "series"=w1085:i32, "accum"=w1084:i32)  [unwired: 3 in]
        n391 = local write "Get Exposure Time"(w1080) -> ()
        n392 = local write "Get Accum Time"(w1081) -> ()
        n393 = local write "Get Kinetic Time"(w1082) -> ()
        n394 = local write "Return from CheckTimings"(w1083) -> ()
        n395 = local write "Return from CheckProcess"(w1086) -> ()
        n396 = local write "Get Kinetic Num"(w1084) -> ()
        n397 = local write "Get Kinetic Num"(w1085) -> ()
      }
      event "Live EMCCD": Value Change {
        # "Set Acquisition Mode: Single Scan or original"
        n398 = event-data() -> ()  [unwired: 1 in, 6 out]
        n399 = case shown="True" "Live EMCCD" {
          tunnel: [0 w1191] -> w1183
          tunnel: [w1189 w1191] -> w1176
          frame False {
            n400 = local read "Aquisition Mode"() -> (w1189:T6)
          }
          frame True {
            w1191 = 1
          }
        }
        n401 = flat-sequence {
          tunnel: w1180 -> [w1193]
          tunnel: [w1193] -> w1184
          tunnel: w1183 -> [w1192]
          tunnel: w1184 -> [w1197]
          tunnel: [w1196] -> w1182
          tunnel: w1176 -> [w1194]
          tunnel: [w1199] -> w1179
          tunnel: w1182 -> [w1199]
          tunnel: "Live EMCCD" -> [w1198]
          frame #0 {
            n402 = local write "Running Status"(w1192) -> ()
          }
          frame #1 {
            n403 = To Unsigned Word Integer(number=w1194) -> (unsigned 16bit integer=w1195:u16)
            n404 = call <userlib>:"SetAcquisitionMode.vi"("error in (no error)"=w1197, "mode"=w1195) -> ("error out"=w1196:errorcluster)  [unwired: 1 out]
          }
          frame #2 {
            n405 = local write "EMCCD Status"(w1198) -> ()
          }
        }
      }
      event "Snap": Mouse Up {
        n406 = event-data() -> ()  [unwired: 1 in, 8 out]
        n407 = local write "Running Status"(2) -> ()
      }
      event "Acquire": Mouse Up {
        n408 = event-data() -> ()  [unwired: 1 in, 8 out]
        n409 = local write "Running Status"(3) -> ()
      }
      event "Abort": Mouse Up {
        n410 = event-data() -> ()  [unwired: 1 in, 8 out]
        n411 = local write "Running Status"(0) -> ()
      }
      event "Intensity Min": Value Change {
        n412 = event-data() -> ()  [unwired: 1 in, 6 out]
        n413 = property on="Intensity Graph" class="IntGraph (strict)"("ZScale.Minimum"="Intensity Min") -> ()  [unwired: 2 in, 2 out]
      }
      event "Intensity Max": Value Change {
        n414 = event-data() -> ()  [unwired: 1 in, 6 out]
        n415 = property on="Intensity Graph" class="IntGraph (strict)"("ZScale.Maximum"="Intensity Max") -> ()  [unwired: 2 in, 2 out]
      }
      event "Auto Scale": Value Change {
        n416 = event-data() -> ()  [unwired: 1 in, 6 out]
        n417 = property on="Intensity Graph" class="IntGraph (strict)"("ZScale.LooseFit"="Auto Scale") -> ()  [unwired: 2 in, 2 out]
      }
      event "left": Mouse Up {
        n418 = event-data() -> ()  [unwired: 1 in, 8 out]
        n419 = local read "XY step"() -> (w1248:dbl)
        n420 = Number To Fractional String(number=w1248, precision (6)=1) -> (F-format string=w1254:string)  [unwired: 2 in]
        n421 = Concatenate Strings("movrel x=", w1254) -> (w1256:string)
        n422 = call "WriteCmd.vi"("error IO"=w1250, "Command"=w1256, "VISA resource name"=w1252) -> ("error"=w1249:errorcluster)
      }
      event "right": Mouse Up {
        n423 = event-data() -> ()  [unwired: 1 in, 8 out]
        n424 = local read "XY step"() -> (w1262:dbl)
        n425 = Number To Fractional String(number=w1262, precision (6)=1) -> (F-format string=w1268:string)  [unwired: 2 in]
        n426 = Concatenate Strings("movrel x=-", w1268) -> (w1270:string)
        n427 = call "WriteCmd.vi"("error IO"=w1264, "Command"=w1270, "VISA resource name"=w1266) -> ("error"=w1263:errorcluster)
      }
      event "front": Mouse Up {
        n428 = event-data() -> ()  [unwired: 1 in, 8 out]
        n429 = local read "XY step"() -> (w1276:dbl)
        n430 = Number To Fractional String(number=w1276, precision (6)=1) -> (F-format string=w1282:string)  [unwired: 2 in]
        n431 = Concatenate Strings("movrel y=-", w1282) -> (w1284:string)
        n432 = call "WriteCmd.vi"("error IO"=w1278, "Command"=w1284, "VISA resource name"=w1280) -> ("error"=w1277:errorcluster)
      }
      event "back": Mouse Up {
        n433 = event-data() -> ()  [unwired: 1 in, 8 out]
        n434 = local read "XY step"() -> (w1290:dbl)
        n435 = Number To Fractional String(number=w1290, precision (6)=1) -> (F-format string=w1296:string)  [unwired: 2 in]
        n436 = Concatenate Strings("movrel y=", w1296) -> (w1298:string)
        n437 = call "WriteCmd.vi"("error IO"=w1292, "Command"=w1298, "VISA resource name"=w1294) -> ("error"=w1291:errorcluster)
      }
      event "up": Mouse Up {
        n438 = event-data() -> ()  [unwired: 1 in, 8 out]
        n439 = local read "Z step"() -> (w1304:dbl)
        n440 = Number To Fractional String(number=w1304, precision (6)=1) -> (F-format string=w1310:string)  [unwired: 2 in]
        n441 = Concatenate Strings("movrel z=", w1310) -> (w1312:string)
        n442 = call "WriteCmd.vi"("error IO"=w1306, "Command"=w1312, "VISA resource name"=w1308) -> ("error"=w1305:errorcluster)
      }
      event "down": Mouse Up {
        n443 = event-data() -> ()  [unwired: 1 in, 8 out]
        n444 = local read "Z step"() -> (w1318:dbl)
        n445 = Number To Fractional String(number=w1318, precision (6)=1) -> (F-format string=w1324:string)  [unwired: 2 in]
        n446 = Concatenate Strings("movrel z=-", w1324) -> (w1326:string)
        n447 = call "WriteCmd.vi"("error IO"=w1320, "Command"=w1326, "VISA resource name"=w1322) -> ("error"=w1319:errorcluster)
      }
      event "flip mirror button": Mouse Up {
        w1334 = tag "Dev1/ao5" ("physical channels")
        n448 = event-data() -> ()  [unwired: 1 in, 8 out]
        n449 = flat-sequence {
          tunnel: [w1348] -> w1338
          tunnel: w1334 -> [w1346]
          tunnel: w1333 -> [w1345]
          tunnel: [w1349] -> w1337
          tunnel: w1338 -> [w1349]
          tunnel: w1337 -> [w1353]
          tunnel: [w1352] -> w1336
          tunnel: w1334 -> [w1351]
          tunnel: [w1355] -> w1335
          tunnel: w1336 -> [w1355]
          tunnel: w1335 -> [w1359]
          tunnel: w1334 -> [w1358]
          tunnel: [w1357] -> w1332
          frame #0 {
            n450 = call "AO single value.vi"("error in"=w1345, "data"=0.0, "physical channels"=w1346) -> ("error out"=w1348:errorcluster)
          }
          frame #1 {
            n451 = Wait (ms)(milliseconds to wait=u32 100) -> ()  [unwired: 1 out]
          }
          frame #2 {
            n452 = call "AO single value.vi"("error in"=w1353, "data"=5.0, "physical channels"=w1351) -> ("error out"=w1352:errorcluster)
          }
          frame #3 {
            n453 = Wait (ms)(milliseconds to wait=u32 100) -> ()  [unwired: 1 out]
          }
          frame #4 {
            n454 = call "AO single value.vi"("error in"=w1359, "data"=0.0, "physical channels"=w1358) -> ("error out"=w1357:errorcluster)
          }
        }
      }
      event "Send": Mouse Up {
        n455 = event-data() -> ()  [unwired: 1 in, 8 out]
        n456 = call "WriteCmd.vi"("error IO"=w1363, "Command"="Command", "VISA resource name"=w1361) -> ("error"=w1365:errorcluster)
        n457 = VISA Read(VISA resource name=w1361, byte count=u32 4096, error in (no error)=w1365) -> (read buffer=→"Response:":string, error out=w1362:errorcluster)  [unwired: 2 out]
      }
      event "Get Position": Mouse Up {
        n458 = event-data() -> ()  [unwired: 1 in, 8 out]
        n459 = call "Get Current Position.vi"("error in (no error)"=w1376, "Array of axes"="Axis", "VISA in"=w1374) -> ("error out"=w1375:errorcluster, "Array of positions [internal units]"=w1378:dbl[])  [unwired: 6 in, 1 out]
        n460 = Multiply(x=w1378, y=0.1) -> (x*y=→"Position (um)":dbl[])
      }
      event "Record Response": Mouse Up {
        n461 = event-data() -> ()  [unwired: 1 in, 8 out]
        n462 = local read "Net Rp"() -> (w1387:bool)
        n463 = stacked-sequence {
          seq-local: [_ _ _ w1759 _] -> [_ _ _ _ w1784]
          seq-local: [_ _ w1626 _ _] -> [_ _ _ w1758 _]
          seq-local: [_ w1421 _ _ _] -> [_ _ w1627 _ _]
          seq-local: [_ _ w1625 _ _] -> [_ _ _ _ w1780]
          tunnel: [_ _ _ _ w1783] -> w1405
          tunnel: w1404 -> [_ w1434 _ _ _]
          tunnel: [_ _ _ _ w1782] -> w1403
          tunnel: w1402 -> [_ w1433 _ w1760 _]
          tunnel: [_ w1431 _ _ _] -> w1400
          tunnel: w1399 -> [_ _ w1639 _ w1792]
          tunnel: w1398 -> [_ _ w1638 _ w1791]
          tunnel: w1397 -> [_ _ w1637 _ w1790]
          tunnel: w1396 -> [_ _ w1636 _ w1789]
          tunnel: w1395 -> [_ _ w1635 _ w1788]
          tunnel: w1394 -> [_ _ w1634 _ _]
          tunnel: w1393 -> [_ _ w1633 _ w1787]
          tunnel: w1389 -> [_ _ w1632 _ w1786]
          tunnel: w1392 -> [_ _ w1631 _ w1785]
          tunnel: [_ _ _ _ w1779] -> w1391
          tunnel: [_ _ w1629 _ _] -> w1390
          tunnel: [_ _ w1628 _ _] -> w1388
          tunnel: w1387 -> [_ _ _ w1757 w1781]
          frame #0 {
            # "Create output folder path"
            n464 = local read "Base Path"() -> (w1406:path)
            n465 = local read "Subfolder"() -> (w1409:string)
            n466 = local write "Current status"("Check single response") -> ()
            n467 = Build Path(base path=w1406, name or relative path=w1409) -> (appended path=w1408:path)
            n468 = call <vilib>:"Check if File or Folder Exists.vi"("path"=w1408) -> ("error out"=w1410:errorcluster, "file or folder exists?"=w1411:bool)  [unwired: 8 in, 1 out]
            n469 = case shown="True" w1411 {
              tunnel: w1408 -> [w1414 w1419]
              tunnel: w1410 -> [w1413 w1420]
              tunnel: [w1412 w1415] -> _
              frame False {
                n470 = Create Folder(path (use dialog)=w1414, error in=w1413) -> (error out=w1412:errorcluster)  [unwired: 1 in, 2 out]
              }
              frame True {
                n471 = Delete(path (use dialog)=w1419, entire hierarchy (F)=TRUE, error in=w1420) -> (deleted path=w1417:path, error out=w1416:errorcluster)  [unwired: 2 in, 1 out]
                n472 = Create Folder(path (use dialog)=w1417, error in=w1416) -> (error out=w1415:errorcluster)  [unwired: 1 in, 2 out]
              }
            }
            n473 = local write "AO output"(w1408) -> ()
          }
          frame #1 {
            # "Delay for DM response"
            # "Apply command to DM"
            n474 = local read "Initial offset"() -> (w1432:bool)
            n475 = case shown="True" w1432 {
              tunnel: [w1520 w1525] -> w1423
              frame False {
                n476 = Initialize Array(0.0, 52) -> (w1520:dbl[])
              }
              frame True {
                n477 = local read "Offset command file"() -> (w1524:path)
                n478 = call-poly <vilib>:"Read From Spreadsheet File.vi"("format (%.3f)"="%.8f", "file path (dialog if empty)"=w1524) -> ("first row"=w1525:dbl[])  [unwired: 5 in, 4 out]
              }
            }
            n479 = local read "Additional Command"() -> (w1438:bool)
            n480 = case shown="True" w1438 {
              tunnel: [w1527 w1533] -> w1424
              tunnel: [w1526 w1532] -> w1435
              tunnel: w1434 -> [w1526 w1531]
              frame False {
                n481 = Initialize Array(0.0, 52) -> (w1527:dbl[])
              }
              frame True {
                n482 = local read "Input type"() -> (w1530:T8)
                n483 = case shown="\"DM actuators\"" w1530 {
                  tunnel: w1531 -> [w1534 w1540 w1582 w1596 w1605]
                  tunnel: [w1535 w1538 w1583 w1594 w1607] -> w1533
                  tunnel: [w1534 w1539 w1582 w1593 w1604] -> w1532
                  frame "Zero Input" {
                    n484 = Initialize Array(0.0, 52) -> (w1535:dbl[])
                  }
                  frame "DM actuators" {
                    w1542 = 1
                    w1543 = 52
                    n485 = local read "Zern/DM index in"() -> (w1549:i32[])
                    n486 = local read "Zern/DM coef in"() -> (w1550:sgl[])
                    n487 = Array Size(array=w1549) -> (size(s)=w1544:i32)
                    n488 = Initialize Array(0.0, w1543) -> (w1546:dbl[])
                    n489 = call-poly <vilib>:"Ramp Pattern.vi"("start"=w1542, "end"=w1543, "delta"=w1542) -> ("Ramp Pattern"=w1547:dbl[])  [unwired: 6 in, 2 out]
                    n490 = Less Or Equal?(x=w1544, y=w1543) -> (x <= y?=w1545:bool)
                    n491 = case shown="True" w1545 {
                      tunnel: w1544 -> [_ w1561]
                      tunnel: w1546 -> [w1554 w1560]
                      tunnel: [w1554 w1559] -> w1538
                      tunnel: w1549 -> [_ w1558]
                      tunnel: w1550 -> [_ w1557]
                      tunnel: [w1551 w1555] -> w1539
                      tunnel: w1543 -> [_ w1556]
                      tunnel: w1540 -> [w1553 w1555]
                      frame False {
                        n492 = Merge Errors(w1553, errorcluster {"status"=FALSE, "code"=0, "source"="Wrong Zern index size"} ("error out")) -> (w1551:errorcluster)
                      }
                      frame True {
                        n493 = for {
                          N: w1561 -> [_]
                          shift-right: [w1574] -> w1559
                          shift-left: w1560 -> [w1575]
                          tunnel: w1558 -> [w1571] mode=indexing
                          tunnel: w1557 -> [w1565] mode=indexing
                          tunnel: w1556 -> [w1572]
                          n494 = Greater Than 0?(x=w1571) -> (x > 0?=w1570:bool)
                          n495 = Less Or Equal?(x=w1571, y=w1572) -> (x <= y?=w1562:bool)
                          n496 = And(x=w1570, y=w1562) -> (x .and. y?=w1569:bool)
                          n497 = In Range and Coerce(upper limit=0.8, x=w1565, lower limit=-0.8) -> (coerced(x)=w1566:dbl, In Range?=w1568:bool)
                          n498 = And(x=w1569, y=w1568) -> (x .and. y?=w1567:bool)
                          n499 = Decrement(x=w1571) -> (x-1=w1573:i32)
                          n500 = case shown="True" w1567 {
                            tunnel: w1573 -> [_ w1580]
                            tunnel: w1575 -> [w1576 w1579]
                            tunnel: [w1576 w1578] -> w1574
                            tunnel: w1566 -> [_ w1577]
                            frame False {
                            }
                            frame True {
                              n501 = Replace Array Subset(array=w1579, new element=w1577, index=w1580) -> (w1578:dbl[])
                            }
                          }
                        }
                      }
                    }
                    n502 = local write "Coef out"(w1538) -> ()
                    n503 = To Long Integer(number=w1547) -> (32bit integer=w1548:i32[])
                    n504 = local write "Index out"(w1548) -> ()
                  }
                  frame "Command File" {
                    n505 = local read "Additional file"() -> (w1581:path)
                    n506 = call-poly <vilib>:"Read From Spreadsheet File.vi"("format (%.3f)"="%.8f", "file path (dialog if empty)"=w1581) -> ("first row"=w1583:dbl[])  [unwired: 5 in, 4 out]
                  }
                  frame "Zernike Coef", Default {
                    n507 = local read "Zern/DM index in"() -> (w1585:i32[])
                    n508 = local read "Zern/DM coef in"() -> (w1586:sgl[])
                    n509 = local read "idxType"() -> (w1592:enum16{"Wyant", "ANSI"})
                    n510 = local read "Initial haso file"() -> (w1590:path)
                    n511 = local read "Haso configuration file"() -> (w1591:path)
                    n512 = local read "interaction matrix file"() -> (w1589:path)
                    n513 = call "zern2command.vi"("Haso configuration file"=w1591, "idxType"=w1592, "interaction matrix file"=w1589, "error in (no error)"=w1596, "Zern coef in"=w1586, "Zern index in"=w1585, "Initial haso file"=w1590) -> ("error out"=w1595:errorcluster, "Offset Positions"=w1594:sgl[], "Zern pupil out"=w1597:refnum<class "Pupil.lvclass">, "ModalCoef out"=w1598:refnum<class "ModalCoef.lvclass">)  [unwired: 1 in]
                    n514 = call <userlib>:"LVClass_ModalCoef GetData.vi"("ModalCoef in"=w1598, "Pupil.lvclass"=w1597, "error in (no error)"=w1595) -> ("ModalCoef out"=w1602:refnum<class "ModalCoef.lvclass">, "coef"=w1588:sgl[], "index"=w1587:u32[], "Pupil.lvclass (dup)"=w1601:refnum<class "Pupil.lvclass">, "error out"=w1600:errorcluster)  [unwired: 8 in]
                    n515 = local write "Index out"(w1587) -> ()
                    n516 = call <userlib>:"LVClass_Pupil dtor.vi"("Pupil in"=w1601, "error in (no error)"=w1600) -> ("error out"=w1599:errorcluster)  [unwired: 12 in, 1 out]
                    n517 = local write "Coef out"(w1588) -> ()
                    n518 = call <userlib>:"LVClass_ModalCoef dtor.vi"("ModalCoef in"=w1602, "error in (no error)"=w1599) -> ("error out"=w1593:errorcluster)  [unwired: 12 in, 1 out]
                  }
                  frame "Zernike File" {
                    w1610 = 1
                    n519 = local read "interaction matrix file"() -> (w1614:path)
                    n520 = local read "Initial haso file"() -> (w1612:path)
                    n521 = local read "Haso configuration file"() -> (w1613:path)
                    n522 = local read "Additional file"() -> (w1623:path)
                    n523 = call-poly <vilib>:"Ramp Pattern.vi"("start"=w1610, "end"=32, "delta"=w1610) -> ("Ramp Pattern"=w1611:dbl[])  [unwired: 6 in, 2 out]
                    n524 = To Long Integer(number=w1611) -> (32bit integer=w1608:i32[])
                    n525 = local read "idxType"() -> (w1603:enum16{"Wyant", "ANSI"})
                    n526 = call-poly <vilib>:"Read From Spreadsheet File.vi"("format (%.3f)"="%.8f", "file path (dialog if empty)"=w1623) -> ("first row"=w1615:dbl[])  [unwired: 5 in, 4 out]
                    n527 = call "zern2command.vi"("Haso configuration file"=w1613, "idxType"=w1603, "interaction matrix file"=w1614, "Zern coef in"=w1615, "Zern index in"=w1608, "Initial haso file"=w1612) -> ("error out"=w1616:errorcluster, "Offset Positions"=w1607:sgl[], "Zern pupil out"=w1617:refnum<class "Pupil.lvclass">, "ModalCoef out"=w1618:refnum<class "ModalCoef.lvclass">)  [unwired: 2 in]
                    n528 = call <userlib>:"LVClass_ModalCoef GetData.vi"("ModalCoef in"=w1618, "Pupil.lvclass"=w1617, "error in (no error)"=w1616) -> ("ModalCoef out"=w1622:refnum<class "ModalCoef.lvclass">, "Pupil.lvclass (dup)"=w1621:refnum<class "Pupil.lvclass">, "error out"=w1620:errorcluster)  [unwired: 8 in, 2 out]
                    n529 = call <userlib>:"LVClass_Pupil dtor.vi"("Pupil in"=w1621, "error in (no error)"=w1620) -> ("error out"=w1619:errorcluster)  [unwired: 12 in, 1 out]
                    n530 = call <userlib>:"LVClass_ModalCoef dtor.vi"("ModalCoef in"=w1622, "error in (no error)"=w1619) -> ("error out"=w1606:errorcluster)  [unwired: 12 in, 1 out]
                    n531 = Merge Errors(w1606, w1605) -> (w1604:errorcluster)
                  }
                }
              }
            }
            n532 = local read "File Base Name"() -> (w1425:string)
            n533 = local read "AO output"() -> (w1429:path)
            n534 = local read "Input type"() -> (w1426:T8)
            n535 = local read "Save File"() -> (w1430:bool)
            n536 = local write "Initial Positions"(w1423) -> ()
            n537 = Add(x=w1424, y=w1423) -> (x+y=w1427:dbl[])
            n538 = call <userlib>:"LVClass_WavefrontCorrector Move to Absolute Position.vi"("WavefrontCorrector in"=w1433, "Absolute Positions"=w1427, "error in (no error)"=w1435) -> ("WavefrontCorrector out"=w1436:refnum<class "WavefrontCorrector.lvclass">, "error out"=w1437:errorcluster)  [unwired: 11 in]
            n539 = call <userlib>:"LVClass_WavefrontCorrector Get Current Position.vi"("WavefrontCorrector in"=w1436, "error in (no error)"=w1437) -> ("WavefrontCorrector out"=w1431:refnum<class "WavefrontCorrector.lvclass">, "Wavefront Corrector Position"=w1428:T18, "error out"=w1422:errorcluster)  [unwired: 11 in]
            n540 = case shown="True" w1430 {
              tunnel: w1429 -> [_ w1447]
              tunnel: w1425 -> [_ w1446]
              tunnel: w1423 -> [_ w1445]
              tunnel: w1424 -> [_ w1444]
              tunnel: w1427 -> [_ w1443]
              tunnel: w1426 -> [_ w1442]
              tunnel: w1428 -> [_ w1441]
              frame False {
              }
              frame True {
                n541 = stacked-sequence {
                  tunnel: w1447 -> [w1452 w1461 w1470 w1479 w1486 w1498 w1510]
                  tunnel: w1446 -> [w1450 w1459 w1468 w1477 w1485 w1497 w1509]
                  tunnel: w1445 -> [w1448 _ _ _ _ _ _]
                  tunnel: w1444 -> [_ w1457 _ _ _ _ _]
                  tunnel: w1443 -> [_ _ w1466 _ _ _ _]
                  tunnel: w1442 -> [_ _ _ _ w1484 w1496 w1508]
                  tunnel: w1441 -> [_ _ _ w1475 _ _ _]
                  frame #0 {
                    n542 = Concatenate Strings(w1450, "_cmdOffset", ".dat") -> (w1453:string)
                    n543 = Build Path(base path=w1452, name or relative path=w1453) -> (appended path=w1454:path)
                    n544 = Array To Spreadsheet String(array=w1448, 3:"%f") -> (spreadsheet string=w1455:string)  [unwired: 1 in]
                    n545 = Write to Text File(file (use dialog)=w1454, text=w1455) -> ()  [unwired: 2 in, 3 out]
                  }
                  frame #1 {
                    n546 = Concatenate Strings(w1459, "_cmdAdd", ".dat") -> (w1462:string)
                    n547 = Build Path(base path=w1461, name or relative path=w1462) -> (appended path=w1463:path)
                    n548 = Array To Spreadsheet String(array=w1457, 3:"%f") -> (spreadsheet string=w1464:string)  [unwired: 1 in]
                    n549 = Write to Text File(file (use dialog)=w1463, text=w1464) -> ()  [unwired: 2 in, 3 out]
                  }
                  frame #2 {
                    n550 = Concatenate Strings(w1468, "_cmdFinal", ".dat") -> (w1471:string)
                    n551 = Build Path(base path=w1470, name or relative path=w1471) -> (appended path=w1472:path)
                    n552 = Array To Spreadsheet String(array=w1466, 3:"%f") -> (spreadsheet string=w1473:string)  [unwired: 1 in]
                    n553 = Write to Text File(file (use dialog)=w1472, text=w1473) -> ()  [unwired: 2 in, 3 out]
                  }
                  frame #3 {
                    n554 = Concatenate Strings(w1477, "_cmdFinalMirror", ".dat") -> (w1480:string)
                    n555 = Build Path(base path=w1479, name or relative path=w1480) -> (appended path=w1481:path)
                    n556 = Array To Spreadsheet String(array=w1475, 3:"%f") -> (spreadsheet string=w1482:string)  [unwired: 1 in]
                    n557 = Write to Text File(file (use dialog)=w1481, text=w1482) -> ()  [unwired: 2 in, 3 out]
                  }
                  frame #4 {
                    n558 = case shown="\"Zero Input\"" w1484 {
                      tunnel: w1486 -> [_ w1491]
                      tunnel: w1485 -> [_ w1489]
                      frame "Zero Input" {
                      }
                      frame "Zernike Coef", Default {
                        n559 = local read "Zern/DM coef in"() -> (w1487:sgl[])
                        n560 = Concatenate Strings(w1489, "_zernCoef", ".txt") -> (w1492:string)
                        n561 = Build Path(base path=w1491, name or relative path=w1492) -> (appended path=w1493:path)
                        n562 = Array To Spreadsheet String(array=w1487, 3:"%f") -> (spreadsheet string=w1494:string)  [unwired: 1 in]
                        n563 = Write to Text File(file (use dialog)=w1493, text=w1494) -> ()  [unwired: 2 in, 3 out]
                      }
                    }
                  }
                  frame #5 {
                    n564 = case shown="\"Zernike Coef\", Default" w1496 {
                      tunnel: w1498 -> [_ w1503]
                      tunnel: w1497 -> [_ w1501]
                      frame "Zero Input" {
                      }
                      frame "Zernike Coef", Default {
                        n565 = local read "Zern/DM index in"() -> (w1499:i32[])
                        n566 = Concatenate Strings(w1501, "_zernIdx", ".txt") -> (w1504:string)
                        n567 = Build Path(base path=w1503, name or relative path=w1504) -> (appended path=w1505:path)
                        n568 = Array To Spreadsheet String(array=w1499, 3:"%d") -> (spreadsheet string=w1506:string)  [unwired: 1 in]
                        n569 = Write to Text File(file (use dialog)=w1505, text=w1506) -> ()  [unwired: 2 in, 3 out]
                      }
                    }
                  }
                  frame #6 {
                    n570 = case shown="\"Zernike Coef\", Default" w1508 {
                      tunnel: w1510 -> [_ w1515]
                      tunnel: w1509 -> [_ w1513]
                      frame "Zero Input" {
                      }
                      frame "Zernike Coef", Default {
                        n571 = Concatenate Strings(w1513, "_zernCoefWyant", ".txt") -> (w1516:string)
                        n572 = local read "Coef out"() -> (w1511:sgl[])
                        n573 = Build Path(base path=w1515, name or relative path=w1516) -> (appended path=w1517:path)
                        n574 = Array To Spreadsheet String(array=w1511, 3:"%f") -> (spreadsheet string=w1518:string)  [unwired: 1 in]
                        n575 = Write to Text File(file (use dialog)=w1517, text=w1518) -> ()  [unwired: 2 in, 3 out]
                      }
                    }
                  }
                }
              }
            }
            n576 = local write "Final Positions"(w1427) -> ()
            n577 = local write "DM Actuator Values"(w1428) -> ()
            n578 = flat-sequence {
              tunnel: [w1439] -> w1421
              tunnel: w1422 -> [w1439]
              frame #0 {
                n579 = Wait (ms)(milliseconds to wait=u32 50) -> ()  [unwired: 1 out]
              }
            }
          }
          frame #2 {
            n580 = local read "HASO ready"() -> (w1630:bool)
            n581 = case shown="True" w1630 {
              tunnel: w1639 -> [_ w1665]
              tunnel: w1637 -> [_ w1664]
              tunnel: w1636 -> [_ w1663]
              tunnel: [w1640 w1662] -> w1626
              tunnel: w1638 -> [_ w1661]
              tunnel: w1631 -> [_ w1647]
              tunnel: w1627 -> [w1640 w1648]
              tunnel: w1634 -> [w1643 w1660]
              tunnel: w1633 -> [w1642 w1659]
              tunnel: [w1643 w1658] -> w1625
              tunnel: [w1642 w1657] -> _
              tunnel: w1635 -> [w1644 w1656]
              tunnel: w1632 -> [w1641 w1655]
              tunnel: [w1644 w1654] -> w1629
              tunnel: [w1641 w1653] -> w1628
              frame False {
              }
              frame True {
                n582 = property on="nb_images (set)" class="DigNum (strict)"() -> ("Value"=w1666:u32)  [unwired: 2 in, 2 out]
                n583 = case shown="2, Default" w1666 {
                  tunnel: [w1754 w1756] -> w1649
                  tunnel: w1661 -> [w1753 _]
                  tunnel: w1665 -> [w1754 _]
                  tunnel: [w1753 w1755] -> w1650
                  tunnel: w1664 -> [_ w1756]
                  tunnel: w1663 -> [_ w1755]
                  frame 2, Default {
                  }
                  frame 1 {
                  }
                }
                n584 = stacked-sequence {
                  tunnel: w1649 -> [_ w1684]
                  tunnel: w1650 -> [_ w1683]
                  tunnel: [_ w1682] -> w1646
                  tunnel: [_ w1680] -> w1645
                  tunnel: [_ w1679] -> _
                  tunnel: w1647 -> [_ w1676]
                  tunnel: w1648 -> [_ w1675]
                  frame #0 {
                    # "Delay until MD gets stable"
                    n585 = local read "exposure_duration_s (set)"() -> (w1667:dbl)
                    n586 = local read "nb_images (set)"() -> (w1668:u32)
                    n587 = Multiply(x=w1667, y=w1668) -> (x*y=w1669:dbl)
                    n588 = Add(x=w1669, y=1.0) -> (x+y=w1670:dbl)
                    n589 = Multiply(x=w1670, y=1000.0) -> (x*y=w1674:dbl)
                    n590 = To Unsigned Long Integer(number=w1674) -> (unsigned 32bit integer=w1673:u32)
                    n591 = Wait (ms)(milliseconds to wait=w1673) -> ()  [unwired: 1 out]
                  }
                  frame #1 {
                    n592 = while {
                      tunnel: w1676 -> [w1689]
                      tunnel: [w1688] -> w1678
                      tunnel: w1675 -> [w1686]
                      tunnel: [w1685] -> w1677
                      stop <- w1687 stop-if-true
                      n593 = call <userlib>:"LVClass_Camera asynchroneImageReady.vi"("Camera in"=w1689, "error in (no error)"=w1686) -> ("Camera out"=w1688:refnum<class "Camera.lvclass">, "ready"=w1687:bool, "error out"=w1685:errorcluster)  [unwired: 11 in]
                    }
                    n594 = call <userlib>:"LVClass_Camera get image.vi"("Camera in"=w1678, "Image"=w1684, "Image RAW"=w1683, "remove_background"=FALSE, "error in (no error)"=w1677) -> ("Camera out"=w1679:refnum<class "Camera.lvclass">, "Image (dup)"=w1682:refnum<class "Image.lvclass">, "error out"=w1680:errorcluster)  [unwired: 7 in, 1 out]
                  }
                }
                n595 = case shown="No Error" w1645 {
                  selector: w1645 -> [w1750 w1751]
                  tunnel: w1646 -> [w1749 w1752]
                  tunnel: [w1746 w1752] -> w1652
                  tunnel: [w1747 w1751] -> w1651
                  frame No Error {
                    # "get image"
                    n596 = call <userlib>:"LVClass_Image get image data.vi"("Image in"=w1749, "error in (no error)"=w1750) -> ("Image out"=w1746:refnum<class "Image.lvclass">, "Image data out"=w1748:u32[][], "error out"=w1747:errorcluster)  [unwired: 11 in]
                    n597 = local write "HASO intensity"(w1748) -> ()
                  }
                  frame Error {
                  }
                }
                n598 = case shown="No Error" w1651 {
                  selector: w1651 -> [w1713 w1745]
                  tunnel: [w1719 w1745] -> w1662
                  tunnel: w1652 -> [w1712 _]
                  tunnel: [w1717 w1741] -> w1653
                  tunnel: [w1716 w1744] -> w1654
                  tunnel: w1660 -> [w1709 w1743]
                  tunnel: w1659 -> [w1708 w1742]
                  tunnel: [w1696 w1743] -> w1658
                  tunnel: [w1707 w1742] -> w1657
                  tunnel: w1656 -> [w1705 w1744]
                  tunnel: w1655 -> [w1703 w1741]
                  frame No Error {
                    # "phaseout"
                    n599 = local read "File Base Name"() -> (w1694:string)
                    n600 = local read "Save File"() -> (w1695:bool)
                    n601 = local read "AO output"() -> (w1693:path)
                    n602 = call "image2slopes.vi"("error in (no error)"=w1713, "Image in"=w1712, "HasoEngine in"=w1708, "HasoSlopes in"=w1709) -> ("error out"=w1706:errorcluster, "HasoEngine out"=w1707:refnum<class "HasoEngine.lvclass">, "HasoSlopes out"=w1690:refnum<class "HasoSlopes.lvclass">)  [unwired: 4 in, 1 out]
                    n603 = local read "Filter"() -> (w1702:u8[])
                    n604 = call "slopes2phase.vi"("TypePhase"=WavefrontReconstructionMode."Modal_Zernike", "Number of coefficients"=u8 32, "error in (no error)"=w1706, "Filter"=w1702, "HasoSlopes in"=w1690, "Phase in"=w1705) -> ("error out"=w1698:errorcluster, "HasoSlopes out"=w1699:refnum<class "HasoSlopes.lvclass">, "Phase out"=w1704:refnum<class "Phase.lvclass">)  [unwired: 3 in]
                    n605 = local read "idxType"() -> (w1692:enum16{"Wyant", "ANSI"})
                    n606 = call "slopes2zern.vi"("HasoSlopes in"=w1699, "error in (no error)"=w1698, "idxType"=w1692) -> ("HasoSlopes out"=w1696:refnum<class "HasoSlopes.lvclass">, "Zernike Coefficients"=w1691:dbl[], "error out"=w1697:errorcluster)  [unwired: 3 in, 2 out]
                    n607 = call <userlib>:"LVClass_Pupil ctor from HasoSlopes.vi"("Pupil in"=w1703, "HasoSlopes.lvclass"=w1690, "error in (no error)"=w1697) -> ("Pupil out"=w1714:refnum<class "Pupil.lvclass">, "error out"=w1715:errorcluster)  [unwired: 11 in]
                    n608 = case shown="True" w1695 {
                      tunnel: w1694 -> [_ w1724]
                      tunnel: w1693 -> [_ w1723]
                      tunnel: w1691 -> [_ w1722]
                      tunnel: w1690 -> [_ w1721]
                      frame False {
                      }
                      frame True {
                        n609 = stacked-sequence {
                          tunnel: w1724 -> [w1728 w1734]
                          tunnel: w1723 -> [w1727 w1733]
                          tunnel: w1722 -> [_ w1732]
                          tunnel: w1721 -> [w1725 _]
                          frame #0 {
                            n610 = Concatenate Strings(w1728, "_slopesMeas", ".has") -> (w1731:string)
                            n611 = Build Path(base path=w1727, name or relative path=w1731) -> (appended path=w1726:path)
                            n612 = call <userlib>:"LVClass_HasoSlopes Save.vi"("HasoSlopes in"=w1725, "path"=w1726) -> ()  [unwired: 12 in, 2 out]
                          }
                          frame #1 {
                            n613 = Concatenate Strings(w1734, "_zernCoefMeas", ".txt") -> (w1737:string)
                            n614 = Build Path(base path=w1733, name or relative path=w1737) -> (appended path=w1738:path)
                            n615 = Array To Spreadsheet String(array=w1732, 3:"%f") -> (spreadsheet string=w1739:string)  [unwired: 1 in]
                            n616 = Write to Text File(file (use dialog)=w1738, text=w1739) -> ()  [unwired: 2 in, 3 out]
                          }
                        }
                      }
                    }
                    n617 = call <userlib>:"LVClasse_Phase GetStatisticDatas.vi"("Phase in"=w1704, "error in (no error)"=w1715) -> ("Phase out"=w1720:refnum<class "Phase.lvclass">, "StatisticsData"=w1700:T2, "error out"=w1718:errorcluster)  [unwired: 11 in]
                    n618 = local write "Phase statistics"(w1700) -> ()
                    n619 = call <userlib>:"LVClasse_Phase Get Data.vi"("Phase in"=w1720, "Pupil"=w1714, "error in (no error)"=w1718) -> ("Phase out"=w1716:refnum<class "Phase.lvclass">, "data"=w1701:sgl[][], "Pupil (dup)"=w1717:refnum<class "Pupil.lvclass">, "error out"=w1719:errorcluster)  [unwired: 9 in]
                    n620 = local write "Zernike Measured"(w1691) -> ()
                    n621 = local write "Phase values"(w1701) -> ()
                  }
                  frame Error {
                  }
                }
              }
            }
          }
          frame #3 {
            # "Apply offset to DM"
            n622 = case shown="True" w1757 {
              tunnel: w1760 -> [_ w1768]
              tunnel: [w1761 w1762] -> w1759
              tunnel: w1758 -> [w1761 w1764]
              frame False {
              }
              frame True {
                # "Delay for DM response"
                n623 = local read "Initial offset"() -> (w1767:bool)
                n624 = case shown="True" w1767 {
                  tunnel: [w1773 w1778] -> w1765
                  frame False {
                    n625 = Initialize Array(0.0, 52) -> (w1773:dbl[])
                  }
                  frame True {
                    n626 = local read "Offset command file"() -> (w1777:path)
                    n627 = call-poly <vilib>:"Read From Spreadsheet File.vi"("format (%.3f)"="%.8f", "file path (dialog if empty)"=w1777) -> ("first row"=w1778:dbl[])  [unwired: 5 in, 4 out]
                  }
                }
                n628 = local write "Initial Positions"(w1765) -> ()
                n629 = call <userlib>:"LVClass_WavefrontCorrector Move to Absolute Position.vi"("WavefrontCorrector in"=w1768, "Absolute Positions"=w1765, "error in (no error)"=w1764) -> ("WavefrontCorrector out"=w1769:refnum<class "WavefrontCorrector.lvclass">, "error out"=w1770:errorcluster)  [unwired: 11 in]
                n630 = call <userlib>:"LVClass_WavefrontCorrector Get Current Position.vi"("WavefrontCorrector in"=w1769, "error in (no error)"=w1770) -> ("Wavefront Corrector Position"=w1766:T18, "error out"=w1763:errorcluster)  [unwired: 11 in, 1 out]
                n631 = local write "Initial Positions"(w1766) -> ()
                n632 = flat-sequence {
                  tunnel: [w1771] -> w1762
                  tunnel: w1763 -> [w1771]
                  frame #0 {
                    n633 = Wait (ms)(milliseconds to wait=u32 50) -> ()  [unwired: 1 out]
                  }
                }
              }
            }
          }
          frame #4 {
            n634 = case shown="True" w1781 {
              tunnel: w1792 -> [_ w1807]
              tunnel: w1791 -> [_ w1806]
              tunnel: w1790 -> [_ w1805]
              tunnel: w1789 -> [_ w1804]
              tunnel: w1788 -> [_ w1803]
              tunnel: w1780 -> [w1793 w1802]
              tunnel: w1787 -> [_ w1801]
              tunnel: w1786 -> [_ w1800]
              tunnel: w1785 -> [_ w1799]
              tunnel: w1784 -> [w1794 w1797]
              tunnel: [w1794 w1796] -> w1782
              tunnel: [w1793 w1795] -> w1779
              frame False {
              }
              frame True {
                n635 = local read "HASO ready"() -> (w1798:bool)
                n636 = case shown="True" w1798 {
                  tunnel: w1807 -> [_ w1835]
                  tunnel: w1805 -> [_ w1834]
                  tunnel: w1804 -> [_ w1833]
                  tunnel: [w1808 w1832] -> w1796
                  tunnel: w1806 -> [_ w1831]
                  tunnel: w1799 -> [_ w1815]
                  tunnel: w1797 -> [w1808 w1814]
                  tunnel: w1802 -> [w1811 w1819]
                  tunnel: w1801 -> [w1810 w1830]
                  tunnel: [w1811 w1821] -> w1795
                  tunnel: [w1810 w1829] -> _
                  tunnel: w1803 -> [w1812 w1828]
                  tunnel: w1800 -> [w1809 w1827]
                  tunnel: [w1812 w1826] -> _
                  tunnel: [w1809 w1825] -> _
                  frame False {
                  }
                  frame True {
                    n637 = property on="nb_images (set)" class="DigNum (strict)"() -> ("Value"=w1836:u32)  [unwired: 2 in, 2 out]
                    n638 = case shown="2, Default" w1836 {
                      tunnel: [w1938 w1940] -> w1817
                      tunnel: w1831 -> [w1937 _]
                      tunnel: w1835 -> [w1938 _]
                      tunnel: [w1937 w1939] -> w1816
                      tunnel: w1834 -> [_ w1940]
                      tunnel: w1833 -> [_ w1939]
                      frame 2, Default {
                      }
                      frame 1 {
                      }
                    }
                    n639 = stacked-sequence {
                      tunnel: w1817 -> [_ w1854]
                      tunnel: w1816 -> [_ w1853]
                      tunnel: [_ w1852] -> w1818
                      tunnel: [_ w1850] -> w1813
                      tunnel: [_ w1849] -> _
                      tunnel: w1815 -> [_ w1846]
                      tunnel: w1814 -> [_ w1845]
                      frame #0 {
                        # "Delay until MD gets stable"
                        n640 = local read "exposure_duration_s (set)"() -> (w1837:dbl)
                        n641 = local read "nb_images (set)"() -> (w1838:u32)
                        n642 = Multiply(x=w1837, y=w1838) -> (x*y=w1839:dbl)
                        n643 = Add(x=w1839, y=1.0) -> (x+y=w1840:dbl)
                        n644 = Multiply(x=w1840, y=1000.0) -> (x*y=w1844:dbl)
                        n645 = To Unsigned Long Integer(number=w1844) -> (unsigned 32bit integer=w1843:u32)
                        n646 = Wait (ms)(milliseconds to wait=w1843) -> ()  [unwired: 1 out]
                      }
                      frame #1 {
                        n647 = while {
                          tunnel: w1846 -> [w1859]
                          tunnel: [w1858] -> w1848
                          tunnel: w1845 -> [w1856]
                          tunnel: [w1855] -> w1847
                          stop <- w1857 stop-if-true
                          n648 = call <userlib>:"LVClass_Camera asynchroneImageReady.vi"("Camera in"=w1859, "error in (no error)"=w1856) -> ("Camera out"=w1858:refnum<class "Camera.lvclass">, "ready"=w1857:bool, "error out"=w1855:errorcluster)  [unwired: 11 in]
                        }
                        n649 = call <userlib>:"LVClass_Camera get image.vi"("Camera in"=w1848, "Image"=w1854, "Image RAW"=w1853, "remove_background"=FALSE, "error in (no error)"=w1847) -> ("Camera out"=w1849:refnum<class "Camera.lvclass">, "Image (dup)"=w1852:refnum<class "Image.lvclass">, "error out"=w1850:errorcluster)  [unwired: 7 in, 1 out]
                      }
                    }
                    n650 = case shown="No Error" w1813 {
                      selector: w1813 -> [w1934 w1935]
                      tunnel: w1818 -> [w1931 w1936]
                      tunnel: [w1930 w1936] -> w1824
                      tunnel: [w1929 w1935] -> w1823
                      frame No Error {
                        # "get image"
                        n651 = call <userlib>:"LVClass_Image get image data.vi"("Image in"=w1931, "error in (no error)"=w1934) -> ("Image out"=w1933:refnum<class "Image.lvclass">, "Image data out"=w1928:u32[][], "error out"=w1932:errorcluster)  [unwired: 11 in]
                        n652 = call <userlib>:"LVClass_Image get image information.vi"("Image in"=w1933, "error in (no error)"=w1932) -> ("Image out"=w1930:refnum<class "Image.lvclass">, "error out"=w1929:errorcluster)  [unwired: 11 in, 1 out]
                        n653 = local write "HASO intensity"(w1928) -> ()
                      }
                      frame Error {
                      }
                    }
                    n654 = case shown="No Error" w1823 {
                      selector: w1823 -> [w1886 w1927]
                      tunnel: [w1892 w1927] -> w1832
                      tunnel: w1824 -> [w1885 _]
                      tunnel: [w1890 w1924] -> w1825
                      tunnel: [w1889 w1926] -> w1826
                      tunnel: refnum<class "HasoSlopes.lvclass"> refnum ("HasoSlopes in") -> [w1882 w1923]
                      tunnel: w1830 -> [w1881 w1925]
                      tunnel: [w1880 w1925] -> w1829
                      tunnel: w1828 -> [w1879 w1926]
                      tunnel: w1827 -> [w1877 w1924]
                      tunnel: [w1862 w1922] -> w1821
                      tunnel: [w1860 w1923] -> w1820
                      tunnel: w1819 -> [w1861 w1922]
                      frame No Error {
                        # "phaseout"
                        n655 = local read "File Base Name"() -> (w1869:string)
                        n656 = local read "Save File"() -> (w1870:bool)
                        n657 = local read "AO output"() -> (w1868:path)
                        n658 = call "image2slopes.vi"("error in (no error)"=w1886, "Image in"=w1885, "HasoEngine in"=w1881, "HasoSlopes in"=w1882) -> ("error out"=w1864:errorcluster, "HasoEngine out"=w1880:refnum<class "HasoEngine.lvclass">, "HasoSlopes out"=w1860:refnum<class "HasoSlopes.lvclass">)  [unwired: 4 in, 1 out]
                        n659 = local read "Filter"() -> (w1876:u8[])
                        n660 = call <userlib>:"LVClass_HasoSlopes Apply Substractor.vi"("HasoSlopes in"=w1861, "HasoSlopes to substract"=w1860, "error in (no error)"=w1864) -> ("HasoSlopes out"=w1865:refnum<class "HasoSlopes.lvclass">, "error out"=w1863:errorcluster)  [unwired: 11 in]
                        n661 = call "slopes2phase.vi"("TypePhase"=WavefrontReconstructionMode."Modal_Zernike", "Number of coefficients"=u8 32, "error in (no error)"=w1863, "Filter"=w1876, "HasoSlopes in"=w1865, "Phase in"=w1879) -> ("error out"=w1872:errorcluster, "HasoSlopes out"=w1873:refnum<class "HasoSlopes.lvclass">, "Phase out"=w1878:refnum<class "Phase.lvclass">)  [unwired: 3 in]
                        n662 = local read "idxType"() -> (w1867:enum16{"Wyant", "ANSI"})
                        n663 = call "slopes2zern.vi"("HasoSlopes in"=w1873, "error in (no error)"=w1872, "idxType"=w1867) -> ("HasoSlopes out"=w1862:refnum<class "HasoSlopes.lvclass">, "Zernike Coefficients"=w1866:dbl[], "error out"=w1871:errorcluster)  [unwired: 3 in, 2 out]
                        n664 = call <userlib>:"LVClass_Pupil ctor from HasoSlopes.vi"("Pupil in"=w1877, "HasoSlopes.lvclass"=w1865, "error in (no error)"=w1871) -> ("Pupil out"=w1887:refnum<class "Pupil.lvclass">, "error out"=w1888:errorcluster)  [unwired: 11 in]
                        n665 = case shown="True" w1870 {
                          tunnel: w1869 -> [_ w1898]
                          tunnel: w1868 -> [_ w1897]
                          tunnel: w1866 -> [_ w1896]
                          tunnel: w1865 -> [_ w1894]
                          tunnel: w1860 -> [_ w1895]
                          frame False {
                          }
                          frame True {
                            n666 = stacked-sequence {
                              tunnel: w1898 -> [w1902 w1909 w1915]
                              tunnel: w1897 -> [w1901 w1908 w1914]
                              tunnel: w1896 -> [_ _ w1913]
                              tunnel: w1895 -> [w1899 _ _]
                              tunnel: w1894 -> [_ w1906 _]
                              frame #0 {
                                n667 = Concatenate Strings(w1902, "_slopesOffset", ".has") -> (w1905:string)
                                n668 = Build Path(base path=w1901, name or relative path=w1905) -> (appended path=w1900:path)
                                n669 = call <userlib>:"LVClass_HasoSlopes Save.vi"("HasoSlopes in"=w1899, "path"=w1900) -> ()  [unwired: 12 in, 2 out]
                              }
                              frame #1 {
                                n670 = Concatenate Strings(w1909, "_slopesNet", ".has") -> (w1912:string)
                                n671 = Build Path(base path=w1908, name or relative path=w1912) -> (appended path=w1907:path)
                                n672 = call <userlib>:"LVClass_HasoSlopes Save.vi"("HasoSlopes in"=w1906, "path"=w1907) -> ()  [unwired: 12 in, 2 out]
                              }
                              frame #2 {
                                n673 = Concatenate Strings(w1915, "_zernCoefNet", ".txt") -> (w1918:string)
                                n674 = Build Path(base path=w1914, name or relative path=w1918) -> (appended path=w1919:path)
                                n675 = Array To Spreadsheet String(array=w1913, 3:"%f") -> (spreadsheet string=w1920:string)  [unwired: 1 in]
                                n676 = Write to Text File(file (use dialog)=w1919, text=w1920) -> ()  [unwired: 2 in, 3 out]
                              }
                            }
                          }
                        }
                        n677 = call <userlib>:"LVClasse_Phase GetStatisticDatas.vi"("Phase in"=w1878, "error in (no error)"=w1888) -> ("Phase out"=w1893:refnum<class "Phase.lvclass">, "StatisticsData"=w1874:T2, "error out"=w1891:errorcluster)  [unwired: 11 in]
                        n678 = local write "Phase statistics"(w1874) -> ()
                        n679 = call <userlib>:"LVClasse_Phase Get Data.vi"("Phase in"=w1893, "Pupil"=w1887, "error in (no error)"=w1891) -> ("Phase out"=w1889:refnum<class "Phase.lvclass">, "data"=w1875:sgl[][], "Pupil (dup)"=w1890:refnum<class "Pupil.lvclass">, "error out"=w1892:errorcluster)  [unwired: 9 in]
                        n680 = local write "Zernike Measured"(w1866) -> ()
                        n681 = local write "Phase values"(w1875) -> ()
                      }
                      frame Error {
                      }
                    }
                    n682 = call <userlib>:"LVClass_HasoSlopes dtor.vi"("HasoSlopes in"=w1820) -> ()  [unwired: 13 in, 2 out]
                  }
                }
              }
            }
            n683 = Unbundle By Name(w1782) -> ("status"=w1783:bool)
          }
        }
      }
      event "Record Batch Zern": Mouse Up {
        n684 = event-data() -> ()  [unwired: 1 in, 8 out]
        n685 = local read "Idx start"() -> (w1941:u32)
        n686 = local read "Idx end"() -> (w1942:u32)
        n687 = Subtract(x=w1942, y=w1941) -> (x-y=w1943:u32)
        n688 = Increment(x=w1943) -> (x+1=w1944:u32)
        n689 = for {
          N: w1944 -> [_]
          tunnel: [w1983] -> w1962
          tunnel: w1956 -> [w1978]
          tunnel: w1955 -> [w1977]
          tunnel: w1954 -> [w1976]
          tunnel: w1953 -> [w1975]
          tunnel: w1950 -> [w1972]
          tunnel: w1949 -> [w1971]
          shift-right: [w1981] -> w1960
          shift-left: w1961 -> [w1982]
          shift-right: [w1979] -> w1957
          shift-left: w1959 -> [w1980]
          shift-right: [w1969] -> w1947
          shift-left: w1952 -> [w1974]
          shift-right: [w1970] -> w1948
          shift-left: w1951 -> [w1973]
          shift-right: [w1967] -> w1945
          shift-left: w1946 -> [w1968]
          tunnel: w1941 -> [w1964]
          i -> [w1965]
          n690 = Add(x=w1964, y=w1965) -> (x+y=w1963:u32)
          n691 = local read "Net Rp"() -> (w1966:bool)
          n692 = stacked-sequence {
            seq-local: [_ _ _ w2279 _] -> [_ _ _ _ w2304]
            seq-local: [_ _ w2144 _ _] -> [_ _ _ w2278 _]
            seq-local: [_ w2013 _ _ _] -> [_ _ w2145 _ _]
            seq-local: [_ _ w2143 _ _] -> [_ _ _ _ w2300]
            tunnel: [_ _ _ _ w2303] -> w1983
            tunnel: w1982 -> [_ w2026 _ _ _]
            tunnel: [_ _ _ _ w2302] -> w1981
            tunnel: w1980 -> [_ w2025 _ w2280 _]
            tunnel: [_ w2023 _ _ _] -> w1979
            tunnel: w1978 -> [_ _ w2157 _ w2312]
            tunnel: w1977 -> [_ _ w2156 _ w2311]
            tunnel: w1976 -> [_ _ w2155 _ w2310]
            tunnel: w1975 -> [_ _ w2154 _ w2309]
            tunnel: w1974 -> [_ _ w2153 _ w2308]
            tunnel: w1973 -> [_ _ w2152 _ _]
            tunnel: w1972 -> [_ _ w2151 _ w2307]
            tunnel: w1968 -> [_ _ w2150 _ w2306]
            tunnel: w1971 -> [_ _ w2149 _ w2305]
            tunnel: [_ _ _ _ w2299] -> w1970
            tunnel: [_ _ w2147 _ _] -> w1969
            tunnel: [_ _ w2146 _ _] -> w1967
            tunnel: w1966 -> [_ _ _ w2277 w2301]
            tunnel: w1963 -> [w1986 w2014 _ _ _]
            frame #0 {
              # "Create output folder path"
              n693 = local read "idxType"() -> (w1990:enum16{"Wyant", "ANSI"})
              n694 = Number To Decimal String(number=w1986) -> (decimal integer string=w1987:string)  [unwired: 1 in]
              n695 = local read "Base Path"() -> (w1984:path)
              n696 = case shown="\"ANSI\"" w1990 {
                tunnel: ["Wyant" "ANSI"] -> w1989
                frame "Wyant", Default {
                }
                frame "ANSI" {
                }
              }
              n697 = local read "Subfolder"() -> (w1996:string)
              n698 = Concatenate Strings(w1989, "_idx_", w1987) -> (w1985:string)
              n699 = Build Path(base path=w1984, name or relative path=w1996) -> (appended path=w1994:path)
              n700 = Build Path(base path=w1994, name or relative path=w1985) -> (appended path=w1991:path)
              n701 = local write "Current status"(w1985) -> ()
              n702 = call <vilib>:"Check if File or Folder Exists.vi"("path"=w1994) -> ("error out"=w1993:errorcluster, "file or folder exists?"=w1995:bool)  [unwired: 8 in, 1 out]
              n703 = case shown="True" w1995 {
                tunnel: w1994 -> [w2003 _]
                tunnel: w1993 -> [w2002 w2004]
                tunnel: [w2001 w2004] -> w1992
                frame False {
                  n704 = Create Folder(path (use dialog)=w2003, error in=w2002) -> (error out=w2001:errorcluster)  [unwired: 1 in, 2 out]
                }
                frame True {
                }
              }
              n705 = call <vilib>:"Check if File or Folder Exists.vi"("error in (no error)"=w1992, "path"=w1991) -> ("error out"=w1997:errorcluster, "file or folder exists?"=w1998:bool)  [unwired: 7 in, 1 out]
              n706 = case shown="False" w1998 {
                tunnel: w1991 -> [w2006 w2010]
                tunnel: w1997 -> [w2005 w2011]
                frame False {
                  n707 = Create Folder(path (use dialog)=w2006, error in=w2005) -> ()  [unwired: 1 in, 3 out]
                }
                frame True {
                  n708 = Delete(path (use dialog)=w2010, entire hierarchy (F)=TRUE, error in=w2011) -> (deleted path=w2008:path, error out=w2007:errorcluster)  [unwired: 2 in, 1 out]
                  n709 = Create Folder(path (use dialog)=w2008, error in=w2007) -> ()  [unwired: 1 in, 3 out]
                }
              }
              n710 = local write "AO output"(w1991) -> ()
            }
            frame #1 {
              # "Delay for DM response"
              # "Apply command to DM"
              n711 = local read "Initial offset"() -> (w2024:bool)
              n712 = case shown="True" w2024 {
                tunnel: [w2112 w2117] -> w2015
                frame False {
                  n713 = Initialize Array(0.0, 52) -> (w2112:dbl[])
                }
                frame True {
                  n714 = local read "Offset command file"() -> (w2116:path)
                  n715 = call-poly <vilib>:"Read From Spreadsheet File.vi"("format (%.3f)"="%.8f", "file path (dialog if empty)"=w2116) -> ("first row"=w2117:dbl[])  [unwired: 5 in, 4 out]
                }
              }
              n716 = local read "Additional Command"() -> (w2030:bool)
              n717 = case shown="True" w2030 {
                tunnel: [w2119 w2142] -> w2016
                tunnel: [w2118 w2141] -> w2027
                tunnel: w2026 -> [w2118 w2140]
                tunnel: w2014 -> [_ w2123]
                frame False {
                  n718 = Initialize Array(0.0, 52) -> (w2119:dbl[])
                }
                frame True {
                  w2124 = 1
                  n719 = local read "Coef value"() -> (w2126:dbl)
                  n720 = local read "Initial haso file"() -> (w2130:path)
                  n721 = Initialize Array(w2123, w2124) -> (w2122:u32[])
                  n722 = Initialize Array(w2126, w2124) -> (w2125:dbl[])
                  n723 = local read "Haso configuration file"() -> (w2131:path)
                  n724 = local read "interaction matrix file"() -> (w2129:path)
                  n725 = local read "idxType"() -> (w2132:enum16{"Wyant", "ANSI"})
                  n726 = call "zern2command.vi"("Haso configuration file"=w2131, "idxType"=w2132, "interaction matrix file"=w2129, "error in (no error)"=w2140, "Zern coef in"=w2125, "Zern index in"=w2122, "Initial haso file"=w2130) -> ("error out"=w2133:errorcluster, "Offset Positions"=w2142:sgl[], "Zern pupil out"=w2134:refnum<class "Pupil.lvclass">, "ModalCoef out"=w2135:refnum<class "ModalCoef.lvclass">)  [unwired: 1 in]
                  n727 = call <userlib>:"LVClass_ModalCoef GetData.vi"("ModalCoef in"=w2135, "Pupil.lvclass"=w2134, "error in (no error)"=w2133) -> ("ModalCoef out"=w2139:refnum<class "ModalCoef.lvclass">, "coef"=w2128:sgl[], "index"=w2127:u32[], "Pupil.lvclass (dup)"=w2138:refnum<class "Pupil.lvclass">, "error out"=w2137:errorcluster)  [unwired: 8 in]
                  n728 = local write "Index out"(w2127) -> ()
                  n729 = call <userlib>:"LVClass_Pupil dtor.vi"("Pupil in"=w2138, "error in (no error)"=w2137) -> ("error out"=w2136:errorcluster)  [unwired: 12 in, 1 out]
                  n730 = local write "Coef out"(w2128) -> ()
                  n731 = call <userlib>:"LVClass_ModalCoef dtor.vi"("ModalCoef in"=w2139, "error in (no error)"=w2136) -> ("error out"=w2141:errorcluster)  [unwired: 12 in, 1 out]
                }
              }
              n732 = local read "File Base Name"() -> (w2017:string)
              n733 = local read "AO output"() -> (w2021:path)
              n734 = local read "Input type"() -> (w2018:T8)
              n735 = local read "Save File"() -> (w2022:bool)
              n736 = local write "Initial Positions"(w2015) -> ()
              n737 = Add(x=w2016, y=w2015) -> (x+y=w2019:dbl[])
              n738 = call <userlib>:"LVClass_WavefrontCorrector Move to Absolute Position.vi"("WavefrontCorrector in"=w2025, "Absolute Positions"=w2019, "error in (no error)"=w2027) -> ("WavefrontCorrector out"=w2028:refnum<class "WavefrontCorrector.lvclass">, "error out"=w2029:errorcluster)  [unwired: 11 in]
              n739 = call <userlib>:"LVClass_WavefrontCorrector Get Current Position.vi"("WavefrontCorrector in"=w2028, "error in (no error)"=w2029) -> ("WavefrontCorrector out"=w2023:refnum<class "WavefrontCorrector.lvclass">, "Wavefront Corrector Position"=w2020:T18, "error out"=w2012:errorcluster)  [unwired: 11 in]
              n740 = case shown="True" w2022 {
                tunnel: w2021 -> [_ w2039]
                tunnel: w2017 -> [_ w2038]
                tunnel: w2015 -> [_ w2037]
                tunnel: w2016 -> [_ w2036]
                tunnel: w2019 -> [_ w2035]
                tunnel: w2018 -> [_ w2034]
                tunnel: w2020 -> [_ w2033]
                frame False {
                }
                frame True {
                  n741 = stacked-sequence {
                    tunnel: w2039 -> [w2044 w2053 w2062 w2071 w2078 w2090 w2102]
                    tunnel: w2038 -> [w2042 w2051 w2060 w2069 w2077 w2089 w2101]
                    tunnel: w2037 -> [w2040 _ _ _ _ _ _]
                    tunnel: w2036 -> [_ w2049 _ _ _ _ _]
                    tunnel: w2035 -> [_ _ w2058 _ _ _ _]
                    tunnel: w2034 -> [_ _ _ _ w2076 w2088 w2100]
                    tunnel: w2033 -> [_ _ _ w2067 _ _ _]
                    frame #0 {
                      n742 = Concatenate Strings(w2042, "_cmdOffset", ".dat") -> (w2045:string)
                      n743 = Build Path(base path=w2044, name or relative path=w2045) -> (appended path=w2046:path)
                      n744 = Array To Spreadsheet String(array=w2040, 3:"%f") -> (spreadsheet string=w2047:string)  [unwired: 1 in]
                      n745 = Write to Text File(file (use dialog)=w2046, text=w2047) -> ()  [unwired: 2 in, 3 out]
                    }
                    frame #1 {
                      n746 = Concatenate Strings(w2051, "_cmdAdd", ".dat") -> (w2054:string)
                      n747 = Build Path(base path=w2053, name or relative path=w2054) -> (appended path=w2055:path)
                      n748 = Array To Spreadsheet String(array=w2049, 3:"%f") -> (spreadsheet string=w2056:string)  [unwired: 1 in]
                      n749 = Write to Text File(file (use dialog)=w2055, text=w2056) -> ()  [unwired: 2 in, 3 out]
                    }
                    frame #2 {
                      n750 = Concatenate Strings(w2060, "_cmdFinal", ".dat") -> (w2063:string)
                      n751 = Build Path(base path=w2062, name or relative path=w2063) -> (appended path=w2064:path)
                      n752 = Array To Spreadsheet String(array=w2058, 3:"%f") -> (spreadsheet string=w2065:string)  [unwired: 1 in]
                      n753 = Write to Text File(file (use dialog)=w2064, text=w2065) -> ()  [unwired: 2 in, 3 out]
                    }
                    frame #3 {
                      n754 = Concatenate Strings(w2069, "_cmdFinalMirror", ".dat") -> (w2072:string)
                      n755 = Build Path(base path=w2071, name or relative path=w2072) -> (appended path=w2073:path)
                      n756 = Array To Spreadsheet String(array=w2067, 3:"%f") -> (spreadsheet string=w2074:string)  [unwired: 1 in]
                      n757 = Write to Text File(file (use dialog)=w2073, text=w2074) -> ()  [unwired: 2 in, 3 out]
                    }
                    frame #4 {
                      n758 = case shown="\"Zernike Coef\", Default" w2076 {
                        tunnel: w2078 -> [_ w2083]
                        tunnel: w2077 -> [_ w2081]
                        frame "Zero Input" {
                        }
                        frame "Zernike Coef", Default {
                          n759 = local read "Zern/DM coef in"() -> (w2079:sgl[])
                          n760 = Concatenate Strings(w2081, "_zernCoef", ".txt") -> (w2084:string)
                          n761 = Build Path(base path=w2083, name or relative path=w2084) -> (appended path=w2085:path)
                          n762 = Array To Spreadsheet String(array=w2079, 3:"%f") -> (spreadsheet string=w2086:string)  [unwired: 1 in]
                          n763 = Write to Text File(file (use dialog)=w2085, text=w2086) -> ()  [unwired: 2 in, 3 out]
                        }
                      }
                    }
                    frame #5 {
                      n764 = case shown="\"Zernike Coef\", Default" w2088 {
                        tunnel: w2090 -> [_ w2095]
                        tunnel: w2089 -> [_ w2093]
                        frame "Zero Input" {
                        }
                        frame "Zernike Coef", Default {
                          n765 = local read "Zern/DM index in"() -> (w2091:i32[])
                          n766 = Concatenate Strings(w2093, "_zernIdx", ".txt") -> (w2096:string)
                          n767 = Build Path(base path=w2095, name or relative path=w2096) -> (appended path=w2097:path)
                          n768 = Array To Spreadsheet String(array=w2091, 3:"%d") -> (spreadsheet string=w2098:string)  [unwired: 1 in]
                          n769 = Write to Text File(file (use dialog)=w2097, text=w2098) -> ()  [unwired: 2 in, 3 out]
                        }
                      }
                    }
                    frame #6 {
                      n770 = case shown="\"Zernike Coef\", Default" w2100 {
                        tunnel: w2102 -> [_ w2107]
                        tunnel: w2101 -> [_ w2105]
                        frame "Zero Input" {
                        }
                        frame "Zernike Coef", Default {
                          n771 = Concatenate Strings(w2105, "_zernCoefWyant", ".txt") -> (w2108:string)
                          n772 = local read "Coef out"() -> (w2103:sgl[])
                          n773 = Build Path(base path=w2107, name or relative path=w2108) -> (appended path=w2109:path)
                          n774 = Array To Spreadsheet String(array=w2103, 3:"%f") -> (spreadsheet string=w2110:string)  [unwired: 1 in]
                          n775 = Write to Text File(file (use dialog)=w2109, text=w2110) -> ()  [unwired: 2 in, 3 out]
                        }
                      }
                    }
                  }
                }
              }
              n776 = local write "Final Positions"(w2019) -> ()
              n777 = local write "DM Actuator Values"(w2020) -> ()
              n778 = flat-sequence {
                tunnel: [w2031] -> w2013
                tunnel: w2012 -> [w2031]
                frame #0 {
                  n779 = Wait (ms)(milliseconds to wait=u32 50) -> ()  [unwired: 1 out]
                }
              }
            }
            frame #2 {
              n780 = local read "HASO ready"() -> (w2148:bool)
              n781 = case shown="True" w2148 {
                tunnel: w2157 -> [_ w2183]
                tunnel: w2155 -> [_ w2182]
                tunnel: w2154 -> [_ w2181]
                tunnel: [w2158 w2180] -> w2144
                tunnel: w2156 -> [_ w2179]
                tunnel: w2149 -> [_ w2166]
                tunnel: w2145 -> [w2158 w2165]
                tunnel: w2152 -> [w2161 w2178]
                tunnel: w2151 -> [w2160 w2177]
                tunnel: [w2161 w2176] -> w2143
                tunnel: [w2160 w2175] -> _
                tunnel: w2153 -> [w2162 w2174]
                tunnel: w2150 -> [w2159 w2173]
                tunnel: [w2162 w2172] -> w2147
                tunnel: [w2159 w2171] -> w2146
                frame False {
                }
                frame True {
                  n782 = property on="nb_images (set)" class="DigNum (strict)"() -> ("Value"=w2184:u32)  [unwired: 2 in, 2 out]
                  n783 = case shown="2, Default" w2184 {
                    tunnel: [w2274 w2276] -> w2164
                    tunnel: w2179 -> [w2273 _]
                    tunnel: w2183 -> [w2274 _]
                    tunnel: [w2273 w2275] -> w2163
                    tunnel: w2182 -> [_ w2276]
                    tunnel: w2181 -> [_ w2275]
                    frame 2, Default {
                    }
                    frame 1 {
                    }
                  }
                  n784 = stacked-sequence {
                    tunnel: w2164 -> [_ w2202]
                    tunnel: w2163 -> [_ w2201]
                    tunnel: [_ w2200] -> w2167
                    tunnel: [_ w2198] -> w2168
                    tunnel: [_ w2197] -> _
                    tunnel: w2166 -> [_ w2194]
                    tunnel: w2165 -> [_ w2193]
                    frame #0 {
                      # "Delay until MD gets stable"
                      n785 = local read "exposure_duration_s (set)"() -> (w2185:dbl)
                      n786 = local read "nb_images (set)"() -> (w2186:u32)
                      n787 = Multiply(x=w2185, y=w2186) -> (x*y=w2187:dbl)
                      n788 = Add(x=w2187, y=3.0) -> (x+y=w2188:dbl)
                      n789 = Multiply(x=w2188, y=1000.0) -> (x*y=w2192:dbl)
                      n790 = To Unsigned Long Integer(number=w2192) -> (unsigned 32bit integer=w2191:u32)
                      n791 = Wait (ms)(milliseconds to wait=w2191) -> ()  [unwired: 1 out]
                    }
                    frame #1 {
                      n792 = while {
                        tunnel: w2194 -> [w2207]
                        tunnel: [w2206] -> w2196
                        tunnel: w2193 -> [w2204]
                        tunnel: [w2203] -> w2195
                        stop <- w2205 stop-if-true
                        n793 = call <userlib>:"LVClass_Camera asynchroneImageReady.vi"("Camera in"=w2207, "error in (no error)"=w2204) -> ("Camera out"=w2206:refnum<class "Camera.lvclass">, "ready"=w2205:bool, "error out"=w2203:errorcluster)  [unwired: 11 in]
                      }
                      n794 = call <userlib>:"LVClass_Camera get image.vi"("Camera in"=w2196, "Image"=w2202, "Image RAW"=w2201, "remove_background"=FALSE, "error in (no error)"=w2195) -> ("Camera out"=w2197:refnum<class "Camera.lvclass">, "Image (dup)"=w2200:refnum<class "Image.lvclass">, "error out"=w2198:errorcluster)  [unwired: 7 in, 1 out]
                    }
                  }
                  n795 = case shown="No Error" w2168 {
                    selector: w2168 -> [w2270 w2271]
                    tunnel: w2167 -> [w2264 w2272]
                    tunnel: [w2267 w2272] -> w2170
                    tunnel: [w2266 w2271] -> w2169
                    frame No Error {
                      # "get image"
                      n796 = call <userlib>:"LVClass_Image get image data.vi"("Image in"=w2264, "error in (no error)"=w2270) -> ("Image out"=w2269:refnum<class "Image.lvclass">, "Image data out"=w2265:u32[][], "error out"=w2268:errorcluster)  [unwired: 11 in]
                      n797 = call <userlib>:"LVClass_Image get image information.vi"("Image in"=w2269, "error in (no error)"=w2268) -> ("Image out"=w2267:refnum<class "Image.lvclass">, "error out"=w2266:errorcluster)  [unwired: 11 in, 1 out]
                      n798 = local write "HASO intensity"(w2265) -> ()
                    }
                    frame Error {
                    }
                  }
                  n799 = case shown="No Error" w2169 {
                    selector: w2169 -> [w2231 w2263]
                    tunnel: [w2237 w2263] -> w2180
                    tunnel: w2170 -> [w2230 _]
                    tunnel: [w2235 w2259] -> w2171
                    tunnel: [w2234 w2262] -> w2172
                    tunnel: w2178 -> [w2227 w2261]
                    tunnel: w2177 -> [w2226 w2260]
                    tunnel: [w2214 w2261] -> w2176
                    tunnel: [w2225 w2260] -> w2175
                    tunnel: w2174 -> [w2223 w2262]
                    tunnel: w2173 -> [w2221 w2259]
                    frame No Error {
                      # "phaseout"
                      n800 = local read "File Base Name"() -> (w2212:string)
                      n801 = local read "Save File"() -> (w2213:bool)
                      n802 = local read "AO output"() -> (w2211:path)
                      n803 = call "image2slopes.vi"("error in (no error)"=w2231, "Image in"=w2230, "HasoEngine in"=w2226, "HasoSlopes in"=w2227) -> ("error out"=w2224:errorcluster, "HasoEngine out"=w2225:refnum<class "HasoEngine.lvclass">, "HasoSlopes out"=w2208:refnum<class "HasoSlopes.lvclass">)  [unwired: 4 in, 1 out]
                      n804 = local read "Filter"() -> (w2220:u8[])
                      n805 = call "slopes2phase.vi"("TypePhase"=WavefrontReconstructionMode."Modal_Zernike", "Number of coefficients"=u8 32, "error in (no error)"=w2224, "Filter"=w2220, "HasoSlopes in"=w2208, "Phase in"=w2223) -> ("error out"=w2216:errorcluster, "HasoSlopes out"=w2217:refnum<class "HasoSlopes.lvclass">, "Phase out"=w2222:refnum<class "Phase.lvclass">)  [unwired: 3 in]
                      n806 = local read "idxType"() -> (w2210:enum16{"Wyant", "ANSI"})
                      n807 = call "slopes2zern.vi"("HasoSlopes in"=w2217, "error in (no error)"=w2216, "idxType"=w2210) -> ("HasoSlopes out"=w2214:refnum<class "HasoSlopes.lvclass">, "Zernike Coefficients"=w2209:dbl[], "error out"=w2215:errorcluster)  [unwired: 3 in, 2 out]
                      n808 = call <userlib>:"LVClass_Pupil ctor from HasoSlopes.vi"("Pupil in"=w2221, "HasoSlopes.lvclass"=w2208, "error in (no error)"=w2215) -> ("Pupil out"=w2232:refnum<class "Pupil.lvclass">, "error out"=w2233:errorcluster)  [unwired: 11 in]
                      n809 = case shown="True" w2213 {
                        tunnel: w2212 -> [_ w2242]
                        tunnel: w2211 -> [_ w2241]
                        tunnel: w2209 -> [_ w2240]
                        tunnel: w2208 -> [_ w2239]
                        frame False {
                        }
                        frame True {
                          n810 = stacked-sequence {
                            tunnel: w2242 -> [w2246 w2252]
                            tunnel: w2241 -> [w2245 w2251]
                            tunnel: w2240 -> [_ w2250]
                            tunnel: w2239 -> [w2243 _]
                            frame #0 {
                              n811 = Concatenate Strings(w2246, "_slopesMeas", ".has") -> (w2249:string)
                              n812 = Build Path(base path=w2245, name or relative path=w2249) -> (appended path=w2244:path)
                              n813 = call <userlib>:"LVClass_HasoSlopes Save.vi"("HasoSlopes in"=w2243, "path"=w2244) -> ()  [unwired: 12 in, 2 out]
                            }
                            frame #1 {
                              n814 = Concatenate Strings(w2252, "_zernCoefMeas", ".txt") -> (w2255:string)
                              n815 = Build Path(base path=w2251, name or relative path=w2255) -> (appended path=w2256:path)
                              n816 = Array To Spreadsheet String(array=w2250, 3:"%f") -> (spreadsheet string=w2257:string)  [unwired: 1 in]
                              n817 = Write to Text File(file (use dialog)=w2256, text=w2257) -> ()  [unwired: 2 in, 3 out]
                            }
                          }
                        }
                      }
                      n818 = call <userlib>:"LVClasse_Phase GetStatisticDatas.vi"("Phase in"=w2222, "error in (no error)"=w2233) -> ("Phase out"=w2238:refnum<class "Phase.lvclass">, "StatisticsData"=w2218:T2, "error out"=w2236:errorcluster)  [unwired: 11 in]
                      n819 = local write "Phase statistics"(w2218) -> ()
                      n820 = call <userlib>:"LVClasse_Phase Get Data.vi"("Phase in"=w2238, "Pupil"=w2232, "error in (no error)"=w2236) -> ("Phase out"=w2234:refnum<class "Phase.lvclass">, "data"=w2219:sgl[][], "Pupil (dup)"=w2235:refnum<class "Pupil.lvclass">, "error out"=w2237:errorcluster)  [unwired: 9 in]
                      n821 = local write "Zernike Measured"(w2209) -> ()
                      n822 = local write "Phase values"(w2219) -> ()
                    }
                    frame Error {
                    }
                  }
                }
              }
            }
            frame #3 {
              # "Apply offset to DM"
              n823 = case shown="True" w2277 {
                tunnel: w2280 -> [_ w2288]
                tunnel: [w2281 w2283] -> w2279
                tunnel: w2278 -> [w2281 w2284]
                frame False {
                }
                frame True {
                  # "Delay for DM response"
                  n824 = local read "Initial offset"() -> (w2287:bool)
                  n825 = case shown="True" w2287 {
                    tunnel: [w2293 w2298] -> w2285
                    frame False {
                      n826 = Initialize Array(0.0, 52) -> (w2293:dbl[])
                    }
                    frame True {
                      n827 = local read "Offset command file"() -> (w2297:path)
                      n828 = call-poly <vilib>:"Read From Spreadsheet File.vi"("format (%.3f)"="%.8f", "file path (dialog if empty)"=w2297) -> ("first row"=w2298:dbl[])  [unwired: 5 in, 4 out]
                    }
                  }
                  n829 = local write "Initial Positions"(w2285) -> ()
                  n830 = call <userlib>:"LVClass_WavefrontCorrector Move to Absolute Position.vi"("WavefrontCorrector in"=w2288, "Absolute Positions"=w2285, "error in (no error)"=w2284) -> ("WavefrontCorrector out"=w2289:refnum<class "WavefrontCorrector.lvclass">, "error out"=w2290:errorcluster)  [unwired: 11 in]
                  n831 = call <userlib>:"LVClass_WavefrontCorrector Get Current Position.vi"("WavefrontCorrector in"=w2289, "error in (no error)"=w2290) -> ("Wavefront Corrector Position"=w2286:T18, "error out"=w2282:errorcluster)  [unwired: 11 in, 1 out]
                  n832 = local write "Initial Positions"(w2286) -> ()
                  n833 = flat-sequence {
                    tunnel: [w2291] -> w2283
                    tunnel: w2282 -> [w2291]
                    frame #0 {
                      n834 = Wait (ms)(milliseconds to wait=u32 50) -> ()  [unwired: 1 out]
                    }
                  }
                }
              }
            }
            frame #4 {
              n835 = case shown="True" w2301 {
                tunnel: w2312 -> [_ w2327]
                tunnel: w2311 -> [_ w2326]
                tunnel: w2310 -> [_ w2325]
                tunnel: w2309 -> [_ w2324]
                tunnel: w2308 -> [_ w2323]
                tunnel: w2300 -> [w2313 w2322]
                tunnel: w2307 -> [_ w2321]
                tunnel: w2306 -> [_ w2320]
                tunnel: w2305 -> [_ w2319]
                tunnel: w2304 -> [w2314 w2317]
                tunnel: [w2314 w2316] -> w2302
                tunnel: [w2313 w2315] -> w2299
                frame False {
                }
                frame True {
                  n836 = local read "HASO ready"() -> (w2318:bool)
                  n837 = case shown="True" w2318 {
                    tunnel: w2327 -> [_ w2355]
                    tunnel: w2325 -> [_ w2354]
                    tunnel: w2324 -> [_ w2353]
                    tunnel: [w2328 w2352] -> w2316
                    tunnel: w2326 -> [_ w2351]
                    tunnel: w2319 -> [_ w2336]
                    tunnel: w2317 -> [w2328 w2335]
                    tunnel: w2322 -> [w2331 w2339]
                    tunnel: w2321 -> [w2330 w2350]
                    tunnel: [w2331 w2341] -> w2315
                    tunnel: [w2330 w2349] -> _
                    tunnel: w2323 -> [w2332 w2348]
                    tunnel: w2320 -> [w2329 w2347]
                    tunnel: [w2332 w2346] -> _
                    tunnel: [w2329 w2345] -> _
                    frame False {
                    }
                    frame True {
                      n838 = property on="nb_images (set)" class="DigNum (strict)"() -> ("Value"=w2356:u32)  [unwired: 2 in, 2 out]
                      n839 = case shown="2, Default" w2356 {
                        tunnel: [w2458 w2460] -> w2338
                        tunnel: w2351 -> [w2457 _]
                        tunnel: w2355 -> [w2458 _]
                        tunnel: [w2457 w2459] -> w2337
                        tunnel: w2354 -> [_ w2460]
                        tunnel: w2353 -> [_ w2459]
                        frame 2, Default {
                        }
                        frame 1 {
                        }
                      }
                      n840 = stacked-sequence {
                        tunnel: w2338 -> [_ w2374]
                        tunnel: w2337 -> [_ w2373]
                        tunnel: [_ w2372] -> w2334
                        tunnel: [_ w2370] -> w2333
                        tunnel: [_ w2369] -> _
                        tunnel: w2336 -> [_ w2366]
                        tunnel: w2335 -> [_ w2365]
                        frame #0 {
                          # "Delay until MD gets stable"
                          n841 = local read "exposure_duration_s (set)"() -> (w2357:dbl)
                          n842 = local read "nb_images (set)"() -> (w2358:u32)
                          n843 = Multiply(x=w2357, y=w2358) -> (x*y=w2359:dbl)
                          n844 = Add(x=w2359, y=3.0) -> (x+y=w2360:dbl)
                          n845 = Multiply(x=w2360, y=1000.0) -> (x*y=w2364:dbl)
                          n846 = To Unsigned Long Integer(number=w2364) -> (unsigned 32bit integer=w2363:u32)
                          n847 = Wait (ms)(milliseconds to wait=w2363) -> ()  [unwired: 1 out]
                        }
                        frame #1 {
                          n848 = while {
                            tunnel: w2366 -> [w2379]
                            tunnel: [w2378] -> w2368
                            tunnel: w2365 -> [w2376]
                            tunnel: [w2375] -> w2367
                            stop <- w2377 stop-if-true
                            n849 = call <userlib>:"LVClass_Camera asynchroneImageReady.vi"("Camera in"=w2379, "error in (no error)"=w2376) -> ("Camera out"=w2378:refnum<class "Camera.lvclass">, "ready"=w2377:bool, "error out"=w2375:errorcluster)  [unwired: 11 in]
                          }
                          n850 = call <userlib>:"LVClass_Camera get image.vi"("Camera in"=w2368, "Image"=w2374, "Image RAW"=w2373, "remove_background"=FALSE, "error in (no error)"=w2367) -> ("Camera out"=w2369:refnum<class "Camera.lvclass">, "Image (dup)"=w2372:refnum<class "Image.lvclass">, "error out"=w2370:errorcluster)  [unwired: 7 in, 1 out]
                        }
                      }
                      n851 = case shown="No Error" w2333 {
                        selector: w2333 -> [w2454 w2455]
                        tunnel: w2334 -> [w2451 w2456]
                        tunnel: [w2450 w2456] -> w2344
                        tunnel: [w2449 w2455] -> w2343
                        frame No Error {
                          # "get image"
                          n852 = call <userlib>:"LVClass_Image get image data.vi"("Image in"=w2451, "error in (no error)"=w2454) -> ("Image out"=w2453:refnum<class "Image.lvclass">, "Image data out"=w2448:u32[][], "error out"=w2452:errorcluster)  [unwired: 11 in]
                          n853 = call <userlib>:"LVClass_Image get image information.vi"("Image in"=w2453, "error in (no error)"=w2452) -> ("Image out"=w2450:refnum<class "Image.lvclass">, "error out"=w2449:errorcluster)  [unwired: 11 in, 1 out]
                          n854 = local write "HASO intensity"(w2448) -> ()
                        }
                        frame Error {
                        }
                      }
                      n855 = case shown="No Error" w2343 {
                        selector: w2343 -> [w2406 w2447]
                        tunnel: [w2412 w2447] -> w2352
                        tunnel: w2344 -> [w2405 _]
                        tunnel: [w2410 w2444] -> w2345
                        tunnel: [w2409 w2446] -> w2346
                        tunnel: refnum<class "HasoSlopes.lvclass"> refnum ("HasoSlopes in") -> [w2402 w2443]
                        tunnel: w2350 -> [w2401 w2445]
                        tunnel: [w2400 w2445] -> w2349
                        tunnel: w2348 -> [w2399 w2446]
                        tunnel: w2347 -> [w2397 w2444]
                        tunnel: [w2382 w2442] -> w2341
                        tunnel: [w2380 w2443] -> w2340
                        tunnel: w2339 -> [w2381 w2442]
                        frame No Error {
                          # "phaseout"
                          n856 = local read "File Base Name"() -> (w2389:string)
                          n857 = local read "Save File"() -> (w2390:bool)
                          n858 = local read "AO output"() -> (w2388:path)
                          n859 = call "image2slopes.vi"("error in (no error)"=w2406, "Image in"=w2405, "HasoEngine in"=w2401, "HasoSlopes in"=w2402) -> ("error out"=w2384:errorcluster, "HasoEngine out"=w2400:refnum<class "HasoEngine.lvclass">, "HasoSlopes out"=w2380:refnum<class "HasoSlopes.lvclass">)  [unwired: 4 in, 1 out]
                          n860 = local read "Filter"() -> (w2396:u8[])
                          n861 = call <userlib>:"LVClass_HasoSlopes Apply Substractor.vi"("HasoSlopes in"=w2381, "HasoSlopes to substract"=w2380, "error in (no error)"=w2384) -> ("HasoSlopes out"=w2385:refnum<class "HasoSlopes.lvclass">, "error out"=w2383:errorcluster)  [unwired: 11 in]
                          n862 = call "slopes2phase.vi"("TypePhase"=WavefrontReconstructionMode."Modal_Zernike", "Number of coefficients"=u8 32, "error in (no error)"=w2383, "Filter"=w2396, "HasoSlopes in"=w2385, "Phase in"=w2399) -> ("error out"=w2392:errorcluster, "HasoSlopes out"=w2393:refnum<class "HasoSlopes.lvclass">, "Phase out"=w2398:refnum<class "Phase.lvclass">)  [unwired: 3 in]
                          n863 = local read "idxType"() -> (w2387:enum16{"Wyant", "ANSI"})
                          n864 = call "slopes2zern.vi"("HasoSlopes in"=w2393, "error in (no error)"=w2392, "idxType"=w2387) -> ("HasoSlopes out"=w2382:refnum<class "HasoSlopes.lvclass">, "Zernike Coefficients"=w2386:dbl[], "error out"=w2391:errorcluster)  [unwired: 3 in, 2 out]
                          n865 = call <userlib>:"LVClass_Pupil ctor from HasoSlopes.vi"("Pupil in"=w2397, "HasoSlopes.lvclass"=w2385, "error in (no error)"=w2391) -> ("Pupil out"=w2407:refnum<class "Pupil.lvclass">, "error out"=w2408:errorcluster)  [unwired: 11 in]
                          n866 = case shown="True" w2390 {
                            tunnel: w2389 -> [_ w2418]
                            tunnel: w2388 -> [_ w2417]
                            tunnel: w2386 -> [_ w2416]
                            tunnel: w2385 -> [_ w2414]
                            tunnel: w2380 -> [_ w2415]
                            frame False {
                            }
                            frame True {
                              n867 = stacked-sequence {
                                tunnel: w2418 -> [w2422 w2429 w2435]
                                tunnel: w2417 -> [w2421 w2428 w2434]
                                tunnel: w2416 -> [_ _ w2433]
                                tunnel: w2415 -> [w2419 _ _]
                                tunnel: w2414 -> [_ w2426 _]
                                frame #0 {
                                n868 = Concatenate Strings(w2422, "_slopesOffset", ".has") -> (w2425:string)
                                n869 = Build Path(base path=w2421, name or relative path=w2425) -> (appended path=w2420:path)
                                n870 = call <userlib>:"LVClass_HasoSlopes Save.vi"("HasoSlopes in"=w2419, "path"=w2420) -> ()  [unwired: 12 in, 2 out]
                                }
                                frame #1 {
                                n871 = Concatenate Strings(w2429, "_slopesNet", ".has") -> (w2432:string)
                                n872 = Build Path(base path=w2428, name or relative path=w2432) -> (appended path=w2427:path)
                                n873 = call <userlib>:"LVClass_HasoSlopes Save.vi"("HasoSlopes in"=w2426, "path"=w2427) -> ()  [unwired: 12 in, 2 out]
                                }
                                frame #2 {
                                n874 = Concatenate Strings(w2435, "_zernCoefNet", ".txt") -> (w2438:string)
                                n875 = Build Path(base path=w2434, name or relative path=w2438) -> (appended path=w2439:path)
                                n876 = Array To Spreadsheet String(array=w2433, 3:"%f") -> (spreadsheet string=w2440:string)  [unwired: 1 in]
                                n877 = Write to Text File(file (use dialog)=w2439, text=w2440) -> ()  [unwired: 2 in, 3 out]
                                }
                              }
                            }
                          }
                          n878 = call <userlib>:"LVClasse_Phase GetStatisticDatas.vi"("Phase in"=w2398, "error in (no error)"=w2408) -> ("Phase out"=w2413:refnum<class "Phase.lvclass">, "StatisticsData"=w2394:T2, "error out"=w2411:errorcluster)  [unwired: 11 in]
                          n879 = local write "Phase statistics"(w2394) -> ()
                          n880 = call <userlib>:"LVClasse_Phase Get Data.vi"("Phase in"=w2413, "Pupil"=w2407, "error in (no error)"=w2411) -> ("Phase out"=w2409:refnum<class "Phase.lvclass">, "data"=w2395:sgl[][], "Pupil (dup)"=w2410:refnum<class "Pupil.lvclass">, "error out"=w2412:errorcluster)  [unwired: 9 in]
                          n881 = local write "Zernike Measured"(w2386) -> ()
                          n882 = local write "Phase values"(w2395) -> ()
                        }
                        frame Error {
                        }
                      }
                      n883 = call <userlib>:"LVClass_HasoSlopes dtor.vi"("HasoSlopes in"=w2340) -> ()  [unwired: 13 in, 2 out]
                    }
                  }
                }
              }
              n884 = Unbundle By Name(w2302) -> ("status"=w2303:bool)
            }
          }
        }
      }
      event "Record Batch Actuator": Mouse Up {
        n885 = event-data() -> ()  [unwired: 1 in, 8 out]
        n886 = local read "Coef value"() -> (w2461:dbl)
        n887 = local read "Idx start"() -> (w2469:u32)
        n888 = Greater Than 0?(x=w2469) -> (x > 0?=w2470:bool)
        n889 = local read "Idx end"() -> (w2467:u32)
        n890 = Less Or Equal?(x=w2467, y=52) -> (x <= y?=w2471:bool)
        n891 = Subtract(x=w2467, y=w2469) -> (x-y=w2472:u32)
        n892 = In Range and Coerce(upper limit=0.8, x=w2461, lower limit=-0.8) -> (In Range?=w2464:bool)  [unwired: 1 out]
        n893 = And(x=w2470, y=w2471) -> (x .and. y?=w2463:bool)
        n894 = Increment(x=w2472) -> (x+1=w2473:u32)
        n895 = And(x=w2463, y=w2464) -> (x .and. y?=w2462:bool)
        n896 = case shown="True" w2462 {
          tunnel: [FALSE w2517] -> w2491
          tunnel: w2490 -> [w2493 w2516]
          tunnel: [w2493 w2515] -> w2489
          tunnel: w2488 -> [w2494 w2514]
          tunnel: [w2494 w2513] -> w2486
          tunnel: w2485 -> [_ w2512]
          tunnel: w2484 -> [_ w2511]
          tunnel: w2483 -> [_ w2510]
          tunnel: w2482 -> [_ w2509]
          tunnel: w2481 -> [w2497 w2508]
          tunnel: w2480 -> [w2496 w2507]
          tunnel: w2479 -> [_ w2506]
          tunnel: w2478 -> [_ w2505]
          tunnel: [w2496 w2504] -> w2477
          tunnel: [w2497 w2503] -> w2476
          tunnel: w2475 -> [w2495 w2502]
          tunnel: [w2495 w2501] -> w2474
          tunnel: w2473 -> [_ w2500]
          tunnel: w2469 -> [_ w2499]
          tunnel: w2461 -> [_ w2498]
          frame False {
          }
          frame True {
            n897 = for {
              N: w2500 -> [_]
              tunnel: [w2539] -> w2517
              tunnel: w2512 -> [w2534]
              tunnel: w2511 -> [w2533]
              tunnel: w2510 -> [w2532]
              tunnel: w2509 -> [w2531]
              tunnel: w2506 -> [w2528]
              tunnel: w2505 -> [w2527]
              shift-right: [w2537] -> w2515
              shift-left: w2516 -> [w2538]
              shift-right: [w2535] -> w2513
              shift-left: w2514 -> [w2536]
              shift-right: [w2526] -> w2503
              shift-left: w2508 -> [w2530]
              shift-right: [w2518] -> w2504
              shift-left: w2507 -> [w2529]
              shift-right: [w2524] -> w2501
              shift-left: w2502 -> [w2525]
              tunnel: w2499 -> [w2522]
              tunnel: w2498 -> [w2520]
              i -> [w2523]
              n898 = Add(x=w2522, y=w2523) -> (x+y=w2521:u32)
              n899 = local read "Net Rp"() -> (w2519:bool)
              n900 = stacked-sequence {
                seq-local: [_ _ _ _ _ _ w3055 _] -> [_ _ _ _ _ _ _ w3078]
                seq-local: [_ _ w2636 _ _ _ _ _] -> [_ _ _ w2770 _ _ _ _]
                seq-local: [_ w2573 _ _ _ _ _ _] -> [_ _ w2637 _ _ _ _ _]
                seq-local: [_ _ w2635 _ _ _ _ _] -> [_ _ _ _ _ w2976 _ _]
                seq-local: [_ _ _ w2769 _ _ _ _] -> [_ _ _ _ w2841 _ _ _]
                seq-local: [_ _ _ _ w2842 _ _ _] -> [_ _ _ _ _ w2974 _ _]
                seq-local: [_ _ _ _ w2840 _ _ _] -> [_ _ _ _ _ w2975 _ _]
                seq-local: [_ _ _ _ _ w2973 _ _] -> [_ _ _ _ _ _ w3053 _]
                tunnel: [_ _ _ _ _ _ _ w3077] -> w2539
                tunnel: w2538 -> [_ w2569 _ _ _ _ _ _]
                tunnel: [_ _ _ _ _ _ _ w3076] -> w2537
                tunnel: w2536 -> [_ w2582 _ w2787 _ _ w3056 _]
                tunnel: [_ w2580 _ _ _ _ _ _] -> w2535
                tunnel: w2534 -> [_ _ w2649 _ w2852 w2984 _ w3086]
                tunnel: w2533 -> [_ _ w2648 _ w2851 w2983 _ w3085]
                tunnel: w2532 -> [_ _ w2647 _ w2850 w2982 _ w3084]
                tunnel: w2531 -> [_ _ w2646 _ w2849 w2981 _ w3083]
                tunnel: w2530 -> [_ _ w2645 _ w2848 w2980 _ w3082]
                tunnel: w2529 -> [_ _ w2644 _ w2847 _ _ _]
                tunnel: w2528 -> [_ _ w2643 _ w2846 _ _ w3081]
                tunnel: w2525 -> [_ _ w2642 _ w2845 w2979 _ w3080]
                tunnel: w2527 -> [_ _ w2641 _ w2844 w2978 _ w3079]
                tunnel: [_ _ w2639 _ _ _ _ _] -> w2526
                tunnel: [_ _ w2638 _ _ _ _ _] -> w2524
                tunnel: w2521 -> [w2542 w2566 _ w2774 _ _ _ _]
                tunnel: w2520 -> [_ w2565 _ w2771 _ _ _ _]
                tunnel: w2519 -> [_ _ _ _ _ _ w3054 w3075]
                tunnel: [_ _ _ _ _ w2972 _ _] -> w2518
                frame #0 {
                  # "Create output folder path"
                  n901 = Number To Decimal String(number=w2542) -> (decimal integer string=w2543:string)  [unwired: 1 in]
                  n902 = local read "Base Path"() -> (w2540:path)
                  n903 = local read "Subfolder"() -> (w2550:string)
                  n904 = Concatenate Strings("A_", w2543) -> (w2541:string)
                  n905 = Build Path(base path=w2540, name or relative path=w2550) -> (appended path=w2548:path)
                  n906 = Build Path(base path=w2548, name or relative path=w2541) -> (appended path=w2545:path)
                  n907 = local write "Current status"(w2541) -> ()
                  n908 = call <vilib>:"Check if File or Folder Exists.vi"("path"=w2548) -> ("error out"=w2547:errorcluster, "file or folder exists?"=w2549:bool)  [unwired: 8 in, 1 out]
                  n909 = case shown="True" w2549 {
                    tunnel: w2548 -> [w2555 _]
                    tunnel: w2547 -> [w2554 w2556]
                    tunnel: [w2553 w2556] -> w2546
                    frame False {
                      n910 = Create Folder(path (use dialog)=w2555, error in=w2554) -> (error out=w2553:errorcluster)  [unwired: 1 in, 2 out]
                    }
                    frame True {
                    }
                  }
                  n911 = call <vilib>:"Check if File or Folder Exists.vi"("error in (no error)"=w2546, "path"=w2545) -> ("error out"=w2551:errorcluster, "file or folder exists?"=w2552:bool)  [unwired: 7 in, 1 out]
                  n912 = case shown="False" w2552 {
                    tunnel: w2545 -> [w2558 w2562]
                    tunnel: w2551 -> [w2557 w2563]
                    frame False {
                      n913 = Create Folder(path (use dialog)=w2558, error in=w2557) -> ()  [unwired: 1 in, 3 out]
                    }
                    frame True {
                      n914 = Delete(path (use dialog)=w2562, entire hierarchy (F)=TRUE, error in=w2563) -> (deleted path=w2560:path, error out=w2559:errorcluster)  [unwired: 2 in, 1 out]
                      n915 = Create Folder(path (use dialog)=w2560, error in=w2559) -> ()  [unwired: 1 in, 3 out]
                    }
                  }
                  n916 = local write "AO output"(w2545) -> ()
                }
                frame #1 {
                  # "Delay for DM response"
                  # "Apply positive command to DM"
                  n917 = local read "Initial offset"() -> (w2581:bool)
                  n918 = case shown="True" w2581 {
                    tunnel: [w2629 w2634] -> w2574
                    frame False {
                      n919 = Initialize Array(0.0, 52) -> (w2629:dbl[])
                    }
                    frame True {
                      n920 = local read "Offset command file"() -> (w2633:path)
                      n921 = call-poly <vilib>:"Read From Spreadsheet File.vi"("format (%.3f)"="%.8f", "file path (dialog if empty)"=w2633) -> ("first row"=w2634:dbl[])  [unwired: 5 in, 4 out]
                    }
                  }
                  n922 = local read "File Base Name"() -> (w2575:string)
                  n923 = local read "AO output"() -> (w2578:path)
                  n924 = Initialize Array(0.0, 52) -> (w2567:dbl[])
                  n925 = local read "Save File"() -> (w2579:bool)
                  n926 = local write "Initial Positions"(w2574) -> ()
                  n927 = Decrement(x=w2566) -> (x-1=w2568:u32)
                  n928 = Replace Array Subset(array=w2567, new element=w2565, index=w2568) -> (w2564:dbl[])
                  n929 = Add(x=w2564, y=w2574) -> (x+y=w2576:dbl[])
                  n930 = call <userlib>:"LVClass_WavefrontCorrector Move to Absolute Position.vi"("WavefrontCorrector in"=w2582, "Absolute Positions"=w2576, "error in (no error)"=w2569) -> ("WavefrontCorrector out"=w2583:refnum<class "WavefrontCorrector.lvclass">, "error out"=w2584:errorcluster)  [unwired: 11 in]
                  n931 = call <userlib>:"LVClass_WavefrontCorrector Get Current Position.vi"("WavefrontCorrector in"=w2583, "error in (no error)"=w2584) -> ("WavefrontCorrector out"=w2580:refnum<class "WavefrontCorrector.lvclass">, "Wavefront Corrector Position"=w2577:T18, "error out"=w2572:errorcluster)  [unwired: 11 in]
                  n932 = case shown="True" w2579 {
                    tunnel: w2578 -> [_ w2592]
                    tunnel: w2575 -> [_ w2591]
                    tunnel: w2574 -> [_ w2590]
                    tunnel: w2564 -> [_ w2589]
                    tunnel: w2576 -> [_ w2588]
                    tunnel: w2577 -> [_ w2587]
                    frame False {
                    }
                    frame True {
                      n933 = stacked-sequence {
                        tunnel: w2592 -> [w2597 w2606 w2615 w2624]
                        tunnel: w2591 -> [w2595 w2604 w2613 w2622]
                        tunnel: w2590 -> [w2593 _ _ _]
                        tunnel: w2589 -> [_ w2602 _ _]
                        tunnel: w2588 -> [_ _ w2611 _]
                        tunnel: w2587 -> [_ _ _ w2620]
                        frame #0 {
                          n934 = Concatenate Strings(w2595, "_cmdOffset_1", ".dat") -> (w2598:string)
                          n935 = Build Path(base path=w2597, name or relative path=w2598) -> (appended path=w2599:path)
                          n936 = Array To Spreadsheet String(array=w2593, 3:"%f") -> (spreadsheet string=w2600:string)  [unwired: 1 in]
                          n937 = Write to Text File(file (use dialog)=w2599, text=w2600) -> ()  [unwired: 2 in, 3 out]
                        }
                        frame #1 {
                          n938 = Concatenate Strings(w2604, "_cmdAdd_1", ".dat") -> (w2607:string)
                          n939 = Build Path(base path=w2606, name or relative path=w2607) -> (appended path=w2608:path)
                          n940 = Array To Spreadsheet String(array=w2602, 3:"%f") -> (spreadsheet string=w2609:string)  [unwired: 1 in]
                          n941 = Write to Text File(file (use dialog)=w2608, text=w2609) -> ()  [unwired: 2 in, 3 out]
                        }
                        frame #2 {
                          n942 = Concatenate Strings(w2613, "_cmdFinal_1", ".dat") -> (w2616:string)
                          n943 = Build Path(base path=w2615, name or relative path=w2616) -> (appended path=w2617:path)
                          n944 = Array To Spreadsheet String(array=w2611, 3:"%f") -> (spreadsheet string=w2618:string)  [unwired: 1 in]
                          n945 = Write to Text File(file (use dialog)=w2617, text=w2618) -> ()  [unwired: 2 in, 3 out]
                        }
                        frame #3 {
                          n946 = Concatenate Strings(w2622, "_cmdFinalMirror_1", ".dat") -> (w2625:string)
                          n947 = Build Path(base path=w2624, name or relative path=w2625) -> (appended path=w2626:path)
                          n948 = Array To Spreadsheet String(array=w2620, 3:"%f") -> (spreadsheet string=w2627:string)  [unwired: 1 in]
                          n949 = Write to Text File(file (use dialog)=w2626, text=w2627) -> ()  [unwired: 2 in, 3 out]
                        }
                      }
                    }
                  }
                  n950 = local write "Final Positions"(w2576) -> ()
                  n951 = local write "DM Actuator Values"(w2577) -> ()
                  n952 = flat-sequence {
                    tunnel: [w2585] -> w2573
                    tunnel: w2572 -> [w2585]
                    frame #0 {
                      n953 = Wait (ms)(milliseconds to wait=u32 50) -> ()  [unwired: 1 out]
                    }
                  }
                }
                frame #2 {
                  n954 = local read "HASO ready"() -> (w2640:bool)
                  n955 = case shown="True" w2640 {
                    tunnel: w2649 -> [_ w2675]
                    tunnel: w2647 -> [_ w2674]
                    tunnel: w2646 -> [_ w2673]
                    tunnel: [w2650 w2672] -> w2636
                    tunnel: w2648 -> [_ w2671]
                    tunnel: w2641 -> [_ w2658]
                    tunnel: w2637 -> [w2650 w2657]
                    tunnel: w2644 -> [w2653 w2670]
                    tunnel: w2643 -> [w2652 w2669]
                    tunnel: [w2653 w2668] -> w2635
                    tunnel: [w2652 w2667] -> _
                    tunnel: w2645 -> [w2654 w2666]
                    tunnel: w2642 -> [w2651 w2665]
                    tunnel: [w2654 w2664] -> w2639
                    tunnel: [w2651 w2663] -> w2638
                    frame False {
                    }
                    frame True {
                      n956 = property on="nb_images (set)" class="DigNum (strict)"() -> ("Value"=w2676:u32)  [unwired: 2 in, 2 out]
                      n957 = case shown="2, Default" w2676 {
                        tunnel: [w2766 w2768] -> w2656
                        tunnel: w2671 -> [w2765 _]
                        tunnel: w2675 -> [w2766 _]
                        tunnel: [w2765 w2767] -> w2655
                        tunnel: w2674 -> [_ w2768]
                        tunnel: w2673 -> [_ w2767]
                        frame 2, Default {
                        }
                        frame 1 {
                        }
                      }
                      n958 = stacked-sequence {
                        tunnel: w2656 -> [_ w2694]
                        tunnel: w2655 -> [_ w2693]
                        tunnel: [_ w2692] -> w2659
                        tunnel: [_ w2690] -> w2660
                        tunnel: [_ w2689] -> _
                        tunnel: w2658 -> [_ w2686]
                        tunnel: w2657 -> [_ w2685]
                        frame #0 {
                          # "Delay until MD gets stable"
                          n959 = local read "exposure_duration_s (set)"() -> (w2677:dbl)
                          n960 = local read "nb_images (set)"() -> (w2678:u32)
                          n961 = Multiply(x=w2677, y=w2678) -> (x*y=w2679:dbl)
                          n962 = Add(x=w2679, y=3.0) -> (x+y=w2680:dbl)
                          n963 = Multiply(x=w2680, y=1000.0) -> (x*y=w2684:dbl)
                          n964 = To Unsigned Long Integer(number=w2684) -> (unsigned 32bit integer=w2683:u32)
                          n965 = Wait (ms)(milliseconds to wait=w2683) -> ()  [unwired: 1 out]
                        }
                        frame #1 {
                          n966 = while {
                            tunnel: w2686 -> [w2699]
                            tunnel: [w2698] -> w2688
                            tunnel: w2685 -> [w2696]
                            tunnel: [w2695] -> w2687
                            stop <- w2697 stop-if-true
                            n967 = call <userlib>:"LVClass_Camera asynchroneImageReady.vi"("Camera in"=w2699, "error in (no error)"=w2696) -> ("Camera out"=w2698:refnum<class "Camera.lvclass">, "ready"=w2697:bool, "error out"=w2695:errorcluster)  [unwired: 11 in]
                          }
                          n968 = call <userlib>:"LVClass_Camera get image.vi"("Camera in"=w2688, "Image"=w2694, "Image RAW"=w2693, "remove_background"=FALSE, "error in (no error)"=w2687) -> ("Camera out"=w2689:refnum<class "Camera.lvclass">, "Image (dup)"=w2692:refnum<class "Image.lvclass">, "error out"=w2690:errorcluster)  [unwired: 7 in, 1 out]
                        }
                      }
                      n969 = case shown="No Error" w2660 {
                        selector: w2660 -> [w2762 w2763]
                        tunnel: w2659 -> [w2756 w2764]
                        tunnel: [w2759 w2764] -> w2662
                        tunnel: [w2758 w2763] -> w2661
                        frame No Error {
                          # "get image"
                          n970 = call <userlib>:"LVClass_Image get image data.vi"("Image in"=w2756, "error in (no error)"=w2762) -> ("Image out"=w2761:refnum<class "Image.lvclass">, "Image data out"=w2757:u32[][], "error out"=w2760:errorcluster)  [unwired: 11 in]
                          n971 = call <userlib>:"LVClass_Image get image information.vi"("Image in"=w2761, "error in (no error)"=w2760) -> ("Image out"=w2759:refnum<class "Image.lvclass">, "error out"=w2758:errorcluster)  [unwired: 11 in, 1 out]
                          n972 = local write "HASO intensity"(w2757) -> ()
                        }
                        frame Error {
                        }
                      }
                      n973 = case shown="No Error" w2661 {
                        selector: w2661 -> [w2723 w2755]
                        tunnel: [w2729 w2755] -> w2672
                        tunnel: w2662 -> [w2722 _]
                        tunnel: [w2727 w2751] -> w2663
                        tunnel: [w2726 w2754] -> w2664
                        tunnel: w2670 -> [w2719 w2753]
                        tunnel: w2669 -> [w2718 w2752]
                        tunnel: [w2706 w2753] -> w2668
                        tunnel: [w2717 w2752] -> w2667
                        tunnel: w2666 -> [w2715 w2754]
                        tunnel: w2665 -> [w2713 w2751]
                        frame No Error {
                          # "phaseout"
                          n974 = local read "File Base Name"() -> (w2704:string)
                          n975 = local read "Save File"() -> (w2705:bool)
                          n976 = local read "AO output"() -> (w2703:path)
                          n977 = call "image2slopes.vi"("error in (no error)"=w2723, "Image in"=w2722, "HasoEngine in"=w2718, "HasoSlopes in"=w2719) -> ("error out"=w2716:errorcluster, "HasoEngine out"=w2717:refnum<class "HasoEngine.lvclass">, "HasoSlopes out"=w2700:refnum<class "HasoSlopes.lvclass">)  [unwired: 4 in, 1 out]
                          n978 = local read "Filter"() -> (w2712:u8[])
                          n979 = call "slopes2phase.vi"("TypePhase"=WavefrontReconstructionMode."Modal_Zernike", "Number of coefficients"=u8 32, "error in (no error)"=w2716, "Filter"=w2712, "HasoSlopes in"=w2700, "Phase in"=w2715) -> ("error out"=w2708:errorcluster, "HasoSlopes out"=w2709:refnum<class "HasoSlopes.lvclass">, "Phase out"=w2714:refnum<class "Phase.lvclass">)  [unwired: 3 in]
                          n980 = local read "idxType"() -> (w2702:enum16{"Wyant", "ANSI"})
                          n981 = call "slopes2zern.vi"("HasoSlopes in"=w2709, "error in (no error)"=w2708, "idxType"=w2702) -> ("HasoSlopes out"=w2706:refnum<class "HasoSlopes.lvclass">, "Zernike Coefficients"=w2701:dbl[], "error out"=w2707:errorcluster)  [unwired: 3 in, 2 out]
                          n982 = call <userlib>:"LVClass_Pupil ctor from HasoSlopes.vi"("Pupil in"=w2713, "HasoSlopes.lvclass"=w2700, "error in (no error)"=w2707) -> ("Pupil out"=w2724:refnum<class "Pupil.lvclass">, "error out"=w2725:errorcluster)  [unwired: 11 in]
                          n983 = case shown="True" w2705 {
                            tunnel: w2704 -> [_ w2734]
                            tunnel: w2703 -> [_ w2733]
                            tunnel: w2701 -> [_ w2732]
                            tunnel: w2700 -> [_ w2731]
                            frame False {
                            }
                            frame True {
                              n984 = stacked-sequence {
                                tunnel: w2734 -> [w2738 w2744]
                                tunnel: w2733 -> [w2737 w2743]
                                tunnel: w2732 -> [_ w2742]
                                tunnel: w2731 -> [w2735 _]
                                frame #0 {
                                n985 = Concatenate Strings(w2738, "_slopesMeas_1", ".has") -> (w2741:string)
                                n986 = Build Path(base path=w2737, name or relative path=w2741) -> (appended path=w2736:path)
                                n987 = call <userlib>:"LVClass_HasoSlopes Save.vi"("HasoSlopes in"=w2735, "path"=w2736) -> ()  [unwired: 12 in, 2 out]
                                }
                                frame #1 {
                                n988 = Concatenate Strings(w2744, "_zernCoefMeas_1", ".txt") -> (w2747:string)
                                n989 = Build Path(base path=w2743, name or relative path=w2747) -> (appended path=w2748:path)
                                n990 = Array To Spreadsheet String(array=w2742, 3:"%f") -> (spreadsheet string=w2749:string)  [unwired: 1 in]
                                n991 = Write to Text File(file (use dialog)=w2748, text=w2749) -> ()  [unwired: 2 in, 3 out]
                                }
                              }
                            }
                          }
                          n992 = call <userlib>:"LVClasse_Phase GetStatisticDatas.vi"("Phase in"=w2714, "error in (no error)"=w2725) -> ("Phase out"=w2730:refnum<class "Phase.lvclass">, "StatisticsData"=w2710:T2, "error out"=w2728:errorcluster)  [unwired: 11 in]
                          n993 = local write "Phase statistics"(w2710) -> ()
                          n994 = call <userlib>:"LVClasse_Phase Get Data.vi"("Phase in"=w2730, "Pupil"=w2724, "error in (no error)"=w2728) -> ("Phase out"=w2726:refnum<class "Phase.lvclass">, "data"=w2711:sgl[][], "Pupil (dup)"=w2727:refnum<class "Pupil.lvclass">, "error out"=w2729:errorcluster)  [unwired: 9 in]
                          n995 = local write "Zernike Measured"(w2701) -> ()
                          n996 = local write "Phase values"(w2711) -> ()
                        }
                        frame Error {
                        }
                      }
                    }
                  }
                }
                frame #3 {
                  # "Delay for DM response"
                  # "Apply negtive command to DM"
                  n997 = local read "Initial offset"() -> (w2786:bool)
                  n998 = case shown="True" w2786 {
                    tunnel: [w2834 w2839] -> w2780
                    frame False {
                      n999 = Initialize Array(0.0, 52) -> (w2834:dbl[])
                    }
                    frame True {
                      n1000 = local read "Offset command file"() -> (w2838:path)
                      n1001 = call-poly <vilib>:"Read From Spreadsheet File.vi"("format (%.3f)"="%.8f", "file path (dialog if empty)"=w2838) -> ("first row"=w2839:dbl[])  [unwired: 5 in, 4 out]
                    }
                  }
                  n1002 = local read "File Base Name"() -> (w2781:string)
                  n1003 = local read "AO output"() -> (w2784:path)
                  n1004 = Initialize Array(0.0, 52) -> (w2775:dbl[])
                  n1005 = local read "Save File"() -> (w2785:bool)
                  n1006 = local write "Initial Positions"(w2780) -> ()
                  n1007 = Negate(x=w2771) -> (-x=w2772:dbl)
                  n1008 = Decrement(x=w2774) -> (x-1=w2776:u32)
                  n1009 = Replace Array Subset(array=w2775, new element=w2772, index=w2776) -> (w2773:dbl[])
                  n1010 = Add(x=w2773, y=w2780) -> (x+y=w2782:dbl[])
                  n1011 = call <userlib>:"LVClass_WavefrontCorrector Move to Absolute Position.vi"("WavefrontCorrector in"=w2787, "Absolute Positions"=w2782, "error in (no error)"=w2770) -> ("WavefrontCorrector out"=w2788:refnum<class "WavefrontCorrector.lvclass">, "error out"=w2789:errorcluster)  [unwired: 11 in]
                  n1012 = call <userlib>:"LVClass_WavefrontCorrector Get Current Position.vi"("WavefrontCorrector in"=w2788, "error in (no error)"=w2789) -> ("Wavefront Corrector Position"=w2783:T18, "error out"=w2779:errorcluster)  [unwired: 11 in, 1 out]
                  n1013 = case shown="True" w2785 {
                    tunnel: w2784 -> [_ w2797]
                    tunnel: w2781 -> [_ w2796]
                    tunnel: w2780 -> [_ w2795]
                    tunnel: w2773 -> [_ w2794]
                    tunnel: w2782 -> [_ w2793]
                    tunnel: w2783 -> [_ w2792]
                    frame False {
                    }
                    frame True {
                      n1014 = stacked-sequence {
                        tunnel: w2797 -> [w2802 w2811 w2820 w2829]
                        tunnel: w2796 -> [w2800 w2809 w2818 w2827]
                        tunnel: w2795 -> [w2798 _ _ _]
                        tunnel: w2794 -> [_ w2807 _ _]
                        tunnel: w2793 -> [_ _ w2816 _]
                        tunnel: w2792 -> [_ _ _ w2825]
                        frame #0 {
                          n1015 = Concatenate Strings(w2800, "_cmdOffset_-1", ".dat") -> (w2803:string)
                          n1016 = Build Path(base path=w2802, name or relative path=w2803) -> (appended path=w2804:path)
                          n1017 = Array To Spreadsheet String(array=w2798, 3:"%f") -> (spreadsheet string=w2805:string)  [unwired: 1 in]
                          n1018 = Write to Text File(file (use dialog)=w2804, text=w2805) -> ()  [unwired: 2 in, 3 out]
                        }
                        frame #1 {
                          n1019 = Concatenate Strings(w2809, "_cmdAdd_-1", ".dat") -> (w2812:string)
                          n1020 = Build Path(base path=w2811, name or relative path=w2812) -> (appended path=w2813:path)
                          n1021 = Array To Spreadsheet String(array=w2807, 3:"%f") -> (spreadsheet string=w2814:string)  [unwired: 1 in]
                          n1022 = Write to Text File(file (use dialog)=w2813, text=w2814) -> ()  [unwired: 2 in, 3 out]
                        }
                        frame #2 {
                          n1023 = Concatenate Strings(w2818, "_cmdFinal_-1", ".dat") -> (w2821:string)
                          n1024 = Build Path(base path=w2820, name or relative path=w2821) -> (appended path=w2822:path)
                          n1025 = Array To Spreadsheet String(array=w2816, 3:"%f") -> (spreadsheet string=w2823:string)  [unwired: 1 in]
                          n1026 = Write to Text File(file (use dialog)=w2822, text=w2823) -> ()  [unwired: 2 in, 3 out]
                        }
                        frame #3 {
                          n1027 = Concatenate Strings(w2827, "_cmdFinalMirror_-1", ".dat") -> (w2830:string)
                          n1028 = Build Path(base path=w2829, name or relative path=w2830) -> (appended path=w2831:path)
                          n1029 = Array To Spreadsheet String(array=w2825, 3:"%f") -> (spreadsheet string=w2832:string)  [unwired: 1 in]
                          n1030 = Write to Text File(file (use dialog)=w2831, text=w2832) -> ()  [unwired: 2 in, 3 out]
                        }
                      }
                    }
                  }
                  n1031 = local write "Final Positions"(w2782) -> ()
                  n1032 = local write "DM Actuator Values"(w2783) -> ()
                  n1033 = flat-sequence {
                    tunnel: [w2790] -> w2769
                    tunnel: w2779 -> [w2790]
                    frame #0 {
                      n1034 = Wait (ms)(milliseconds to wait=u32 50) -> ()  [unwired: 1 out]
                    }
                  }
                }
                frame #4 {
                  n1035 = local read "HASO ready"() -> (w2843:bool)
                  n1036 = case shown="True" w2843 {
                    tunnel: w2852 -> [_ w2878]
                    tunnel: w2850 -> [_ w2877]
                    tunnel: w2849 -> [_ w2876]
                    tunnel: [w2853 w2875] -> w2842
                    tunnel: w2851 -> [_ w2874]
                    tunnel: w2844 -> [_ w2862]
                    tunnel: w2841 -> [w2853 w2861]
                    tunnel: w2847 -> [w2856 _]
                    tunnel: w2846 -> [w2855 w2873]
                    tunnel: [w2856 w2872] -> w2840
                    tunnel: [w2855 w2871] -> _
                    tunnel: w2848 -> [w2857 w2870]
                    tunnel: w2845 -> [w2854 w2869]
                    tunnel: [w2857 w2868] -> _
                    tunnel: [w2854 w2867] -> _
                    frame False {
                    }
                    frame True {
                      n1037 = property on="nb_images (set)" class="DigNum (strict)"() -> ("Value"=w2879:u32)  [unwired: 2 in, 2 out]
                      n1038 = case shown="2, Default" w2879 {
                        tunnel: [w2969 w2971] -> w2860
                        tunnel: w2874 -> [w2968 _]
                        tunnel: w2878 -> [w2969 _]
                        tunnel: [w2968 w2970] -> w2859
                        tunnel: w2877 -> [_ w2971]
                        tunnel: w2876 -> [_ w2970]
                        frame 2, Default {
                        }
                        frame 1 {
                        }
                      }
                      n1039 = stacked-sequence {
                        tunnel: w2860 -> [_ w2897]
                        tunnel: w2859 -> [_ w2896]
                        tunnel: [_ w2895] -> w2863
                        tunnel: [_ w2893] -> w2864
                        tunnel: [_ w2892] -> _
                        tunnel: w2862 -> [_ w2889]
                        tunnel: w2861 -> [_ w2888]
                        frame #0 {
                          # "Delay until MD gets stable"
                          n1040 = local read "exposure_duration_s (set)"() -> (w2880:dbl)
                          n1041 = local read "nb_images (set)"() -> (w2881:u32)
                          n1042 = Multiply(x=w2880, y=w2881) -> (x*y=w2882:dbl)
                          n1043 = Add(x=w2882, y=3.0) -> (x+y=w2883:dbl)
                          n1044 = Multiply(x=w2883, y=1000.0) -> (x*y=w2887:dbl)
                          n1045 = To Unsigned Long Integer(number=w2887) -> (unsigned 32bit integer=w2886:u32)
                          n1046 = Wait (ms)(milliseconds to wait=w2886) -> ()  [unwired: 1 out]
                        }
                        frame #1 {
                          n1047 = while {
                            tunnel: w2889 -> [w2902]
                            tunnel: [w2901] -> w2891
                            tunnel: w2888 -> [w2899]
                            tunnel: [w2898] -> w2890
                            stop <- w2900 stop-if-true
                            n1048 = call <userlib>:"LVClass_Camera asynchroneImageReady.vi"("Camera in"=w2902, "error in (no error)"=w2899) -> ("Camera out"=w2901:refnum<class "Camera.lvclass">, "ready"=w2900:bool, "error out"=w2898:errorcluster)  [unwired: 11 in]
                          }
                          n1049 = call <userlib>:"LVClass_Camera get image.vi"("Camera in"=w2891, "Image"=w2897, "Image RAW"=w2896, "remove_background"=FALSE, "error in (no error)"=w2890) -> ("Camera out"=w2892:refnum<class "Camera.lvclass">, "Image (dup)"=w2895:refnum<class "Image.lvclass">, "error out"=w2893:errorcluster)  [unwired: 7 in, 1 out]
                        }
                      }
                      n1050 = case shown="No Error" w2864 {
                        selector: w2864 -> [w2965 w2966]
                        tunnel: w2863 -> [w2959 w2967]
                        tunnel: [w2962 w2967] -> w2866
                        tunnel: [w2961 w2966] -> w2865
                        frame No Error {
                          # "get image"
                          n1051 = call <userlib>:"LVClass_Image get image data.vi"("Image in"=w2959, "error in (no error)"=w2965) -> ("Image out"=w2964:refnum<class "Image.lvclass">, "Image data out"=w2960:u32[][], "error out"=w2963:errorcluster)  [unwired: 11 in]
                          n1052 = call <userlib>:"LVClass_Image get image information.vi"("Image in"=w2964, "error in (no error)"=w2963) -> ("Image out"=w2962:refnum<class "Image.lvclass">, "error out"=w2961:errorcluster)  [unwired: 11 in, 1 out]
                          n1053 = local write "HASO intensity"(w2960) -> ()
                        }
                        frame Error {
                        }
                      }
                      n1054 = case shown="No Error" w2865 {
                        selector: w2865 -> [w2926 w2958]
                        tunnel: [w2932 w2958] -> w2875
                        tunnel: w2866 -> [w2925 _]
                        tunnel: [w2930 w2954] -> w2867
                        tunnel: [w2929 w2957] -> w2868
                        tunnel: refnum<class "HasoSlopes.lvclass"> refnum ("HasoSlopes in") -> [w2922 w2956]
                        tunnel: w2873 -> [w2921 w2955]
                        tunnel: [w2909 w2956] -> w2872
                        tunnel: [w2920 w2955] -> w2871
                        tunnel: w2870 -> [w2918 w2957]
                        tunnel: w2869 -> [w2916 w2954]
                        frame No Error {
                          # "phaseout"
                          n1055 = local read "File Base Name"() -> (w2907:string)
                          n1056 = local read "Save File"() -> (w2908:bool)
                          n1057 = local read "AO output"() -> (w2906:path)
                          n1058 = call "image2slopes.vi"("error in (no error)"=w2926, "Image in"=w2925, "HasoEngine in"=w2921, "HasoSlopes in"=w2922) -> ("error out"=w2919:errorcluster, "HasoEngine out"=w2920:refnum<class "HasoEngine.lvclass">, "HasoSlopes out"=w2903:refnum<class "HasoSlopes.lvclass">)  [unwired: 4 in, 1 out]
                          n1059 = local read "Filter"() -> (w2915:u8[])
                          n1060 = call "slopes2phase.vi"("TypePhase"=WavefrontReconstructionMode."Modal_Zernike", "Number of coefficients"=u8 32, "error in (no error)"=w2919, "Filter"=w2915, "HasoSlopes in"=w2903, "Phase in"=w2918) -> ("error out"=w2911:errorcluster, "HasoSlopes out"=w2912:refnum<class "HasoSlopes.lvclass">, "Phase out"=w2917:refnum<class "Phase.lvclass">)  [unwired: 3 in]
                          n1061 = local read "idxType"() -> (w2905:enum16{"Wyant", "ANSI"})
                          n1062 = call "slopes2zern.vi"("HasoSlopes in"=w2912, "error in (no error)"=w2911, "idxType"=w2905) -> ("HasoSlopes out"=w2909:refnum<class "HasoSlopes.lvclass">, "Zernike Coefficients"=w2904:dbl[], "error out"=w2910:errorcluster)  [unwired: 3 in, 2 out]
                          n1063 = call <userlib>:"LVClass_Pupil ctor from HasoSlopes.vi"("Pupil in"=w2916, "HasoSlopes.lvclass"=w2903, "error in (no error)"=w2910) -> ("Pupil out"=w2927:refnum<class "Pupil.lvclass">, "error out"=w2928:errorcluster)  [unwired: 11 in]
                          n1064 = case shown="True" w2908 {
                            tunnel: w2907 -> [_ w2937]
                            tunnel: w2906 -> [_ w2936]
                            tunnel: w2904 -> [_ w2935]
                            tunnel: w2903 -> [_ w2934]
                            frame False {
                            }
                            frame True {
                              n1065 = stacked-sequence {
                                tunnel: w2937 -> [w2941 w2947]
                                tunnel: w2936 -> [w2940 w2946]
                                tunnel: w2935 -> [_ w2945]
                                tunnel: w2934 -> [w2938 _]
                                frame #0 {
                                n1066 = Concatenate Strings(w2941, "_slopesMeas_-1", ".has") -> (w2944:string)
                                n1067 = Build Path(base path=w2940, name or relative path=w2944) -> (appended path=w2939:path)
                                n1068 = call <userlib>:"LVClass_HasoSlopes Save.vi"("HasoSlopes in"=w2938, "path"=w2939) -> ()  [unwired: 12 in, 2 out]
                                }
                                frame #1 {
                                n1069 = Concatenate Strings(w2947, "_zernCoefMeas_-1", ".txt") -> (w2950:string)
                                n1070 = Build Path(base path=w2946, name or relative path=w2950) -> (appended path=w2951:path)
                                n1071 = Array To Spreadsheet String(array=w2945, 3:"%f") -> (spreadsheet string=w2952:string)  [unwired: 1 in]
                                n1072 = Write to Text File(file (use dialog)=w2951, text=w2952) -> ()  [unwired: 2 in, 3 out]
                                }
                              }
                            }
                          }
                          n1073 = call <userlib>:"LVClasse_Phase GetStatisticDatas.vi"("Phase in"=w2917, "error in (no error)"=w2928) -> ("Phase out"=w2933:refnum<class "Phase.lvclass">, "StatisticsData"=w2913:T2, "error out"=w2931:errorcluster)  [unwired: 11 in]
                          n1074 = local write "Phase statistics"(w2913) -> ()
                          n1075 = call <userlib>:"LVClasse_Phase Get Data.vi"("Phase in"=w2933, "Pupil"=w2927, "error in (no error)"=w2931) -> ("Phase out"=w2929:refnum<class "Phase.lvclass">, "data"=w2914:sgl[][], "Pupil (dup)"=w2930:refnum<class "Pupil.lvclass">, "error out"=w2932:errorcluster)  [unwired: 9 in]
                          n1076 = local write "Zernike Measured"(w2904) -> ()
                          n1077 = local write "Phase values"(w2914) -> ()
                        }
                        frame Error {
                        }
                      }
                    }
                  }
                }
                frame #5 {
                  n1078 = local read "HASO ready"() -> (w2977:bool)
                  n1079 = case shown="True" w2977 {
                    tunnel: w2984 -> [_ _]
                    tunnel: w2982 -> [_ _]
                    tunnel: w2981 -> [_ _]
                    tunnel: [w2986 w2998] -> w2973
                    tunnel: w2983 -> [_ _]
                    tunnel: w2978 -> [_ _]
                    tunnel: [w2985 w2993] -> w2972
                    tunnel: w2980 -> [w2988 w2997]
                    tunnel: w2979 -> [w2987 w2996]
                    tunnel: [w2988 w2995] -> _
                    tunnel: [w2987 w2994] -> _
                    tunnel: w2976 -> [w2985 w2991]
                    tunnel: w2975 -> [_ w2990]
                    tunnel: w2974 -> [w2986 w2989]
                    frame False {
                    }
                    frame True {
                      n1080 = case shown="No Error" w2989 {
                        selector: w2989 -> [w3000 w3052]
                        tunnel: [w3026 w3052] -> w2998
                        tunnel: [w3024 w3050] -> w2994
                        tunnel: [w3023 w3051] -> w2995
                        tunnel: w2997 -> [w3018 w3051]
                        tunnel: w2996 -> [w3016 w3050]
                        tunnel: [w3002 w3048] -> w2993
                        tunnel: [w2999 w3049] -> w2992
                        tunnel: w2991 -> [w3001 w3048]
                        tunnel: w2990 -> [w2999 w3049]
                        frame No Error {
                          # "phaseout"
                          n1081 = local read "File Base Name"() -> (w3008:string)
                          n1082 = local read "Save File"() -> (w3009:bool)
                          n1083 = local read "AO output"() -> (w3007:path)
                          n1084 = local read "Filter"() -> (w3015:u8[])
                          n1085 = call <userlib>:"LVClass_HasoSlopes Apply Substractor.vi"("HasoSlopes in"=w3001, "HasoSlopes to substract"=w2999, "error in (no error)"=w3000) -> ("HasoSlopes out"=w3004:refnum<class "HasoSlopes.lvclass">, "error out"=w3003:errorcluster)  [unwired: 11 in]
                          n1086 = call "slopes2phase.vi"("TypePhase"=WavefrontReconstructionMode."Modal_Zernike", "Number of coefficients"=u8 32, "error in (no error)"=w3003, "Filter"=w3015, "HasoSlopes in"=w3004, "Phase in"=w3018) -> ("error out"=w3011:errorcluster, "HasoSlopes out"=w3012:refnum<class "HasoSlopes.lvclass">, "Phase out"=w3017:refnum<class "Phase.lvclass">)  [unwired: 3 in]
                          n1087 = local read "idxType"() -> (w3006:enum16{"Wyant", "ANSI"})
                          n1088 = call "slopes2zern.vi"("HasoSlopes in"=w3012, "error in (no error)"=w3011, "idxType"=w3006) -> ("HasoSlopes out"=w3002:refnum<class "HasoSlopes.lvclass">, "Zernike Coefficients"=w3005:dbl[], "error out"=w3010:errorcluster)  [unwired: 3 in, 2 out]
                          n1089 = call <userlib>:"LVClass_Pupil ctor from HasoSlopes.vi"("Pupil in"=w3016, "HasoSlopes.lvclass"=w3004, "error in (no error)"=w3010) -> ("Pupil out"=w3021:refnum<class "Pupil.lvclass">, "error out"=w3022:errorcluster)  [unwired: 11 in]
                          n1090 = case shown="True" w3009 {
                            tunnel: w3008 -> [_ w3031]
                            tunnel: w3007 -> [_ w3030]
                            tunnel: w3005 -> [_ w3029]
                            tunnel: w3004 -> [_ w3028]
                            frame False {
                            }
                            frame True {
                              n1091 = stacked-sequence {
                                tunnel: w3031 -> [w3035 w3041]
                                tunnel: w3030 -> [w3034 w3040]
                                tunnel: w3029 -> [_ w3039]
                                tunnel: w3028 -> [w3032 _]
                                frame #0 {
                                n1092 = Concatenate Strings(w3035, "_slopesNet", ".has") -> (w3038:string)
                                n1093 = Build Path(base path=w3034, name or relative path=w3038) -> (appended path=w3033:path)
                                n1094 = call <userlib>:"LVClass_HasoSlopes Save.vi"("HasoSlopes in"=w3032, "path"=w3033) -> ()  [unwired: 12 in, 2 out]
                                }
                                frame #1 {
                                n1095 = Concatenate Strings(w3041, "_zernCoefNet", ".txt") -> (w3044:string)
                                n1096 = Build Path(base path=w3040, name or relative path=w3044) -> (appended path=w3045:path)
                                n1097 = Array To Spreadsheet String(array=w3039, 3:"%f") -> (spreadsheet string=w3046:string)  [unwired: 1 in]
                                n1098 = Write to Text File(file (use dialog)=w3045, text=w3046) -> ()  [unwired: 2 in, 3 out]
                                }
                              }
                            }
                          }
                          n1099 = call <userlib>:"LVClasse_Phase GetStatisticDatas.vi"("Phase in"=w3017, "error in (no error)"=w3022) -> ("Phase out"=w3027:refnum<class "Phase.lvclass">, "StatisticsData"=w3013:T2, "error out"=w3025:errorcluster)  [unwired: 11 in]
                          n1100 = local write "Phase statistics"(w3013) -> ()
                          n1101 = call <userlib>:"LVClasse_Phase Get Data.vi"("Phase in"=w3027, "Pupil"=w3021, "error in (no error)"=w3025) -> ("Phase out"=w3023:refnum<class "Phase.lvclass">, "data"=w3014:sgl[][], "Pupil (dup)"=w3024:refnum<class "Pupil.lvclass">, "error out"=w3026:errorcluster)  [unwired: 9 in]
                          n1102 = local write "Zernike Measured"(w3005) -> ()
                          n1103 = local write "Phase values"(w3014) -> ()
                        }
                        frame Error {
                        }
                      }
                      n1104 = call <userlib>:"LVClass_HasoSlopes dtor.vi"("HasoSlopes in"=w2992) -> ()  [unwired: 13 in, 2 out]
                    }
                  }
                }
                frame #6 {
                  # "Apply offset to DM"
                  n1105 = case shown="True" w3054 {
                    tunnel: w3056 -> [_ w3064]
                    tunnel: [w3057 w3059] -> w3055
                    tunnel: w3053 -> [w3057 w3060]
                    frame False {
                    }
                    frame True {
                      # "Delay for DM response"
                      n1106 = local read "Initial offset"() -> (w3063:bool)
                      n1107 = case shown="True" w3063 {
                        tunnel: [w3069 w3074] -> w3061
                        frame False {
                          n1108 = Initialize Array(0.0, 52) -> (w3069:dbl[])
                        }
                        frame True {
                          n1109 = local read "Offset command file"() -> (w3073:path)
                          n1110 = call-poly <vilib>:"Read From Spreadsheet File.vi"("format (%.3f)"="%.8f", "file path (dialog if empty)"=w3073) -> ("first row"=w3074:dbl[])  [unwired: 5 in, 4 out]
                        }
                      }
                      n1111 = local write "Initial Positions"(w3061) -> ()
                      n1112 = call <userlib>:"LVClass_WavefrontCorrector Move to Absolute Position.vi"("WavefrontCorrector in"=w3064, "Absolute Positions"=w3061, "error in (no error)"=w3060) -> ("WavefrontCorrector out"=w3065:refnum<class "WavefrontCorrector.lvclass">, "error out"=w3066:errorcluster)  [unwired: 11 in]
                      n1113 = call <userlib>:"LVClass_WavefrontCorrector Get Current Position.vi"("WavefrontCorrector in"=w3065, "error in (no error)"=w3066) -> ("Wavefront Corrector Position"=w3062:T18, "error out"=w3058:errorcluster)  [unwired: 11 in, 1 out]
                      n1114 = local write "Initial Positions"(w3062) -> ()
                      n1115 = flat-sequence {
                        tunnel: [w3067] -> w3059
                        tunnel: w3058 -> [w3067]
                        frame #0 {
                          n1116 = Wait (ms)(milliseconds to wait=u32 50) -> ()  [unwired: 1 out]
                        }
                      }
                    }
                  }
                }
                frame #7 {
                  n1117 = case shown="True" w3075 {
                    tunnel: w3086 -> [_ w3098]
                    tunnel: w3085 -> [_ w3097]
                    tunnel: w3084 -> [_ w3096]
                    tunnel: w3083 -> [_ w3095]
                    tunnel: w3082 -> [_ w3094]
                    tunnel: w3081 -> [_ w3093]
                    tunnel: w3080 -> [_ w3092]
                    tunnel: w3079 -> [_ w3091]
                    tunnel: w3078 -> [w3087 w3089]
                    tunnel: [w3087 w3088] -> w3076
                    frame False {
                    }
                    frame True {
                      n1118 = local read "HASO ready"() -> (w3090:bool)
                      n1119 = case shown="True" w3090 {
                        tunnel: w3098 -> [_ w3123]
                        tunnel: w3096 -> [_ w3122]
                        tunnel: w3095 -> [_ w3121]
                        tunnel: [w3099 w3120] -> w3088
                        tunnel: w3097 -> [_ w3119]
                        tunnel: w3091 -> [_ w3106]
                        tunnel: w3089 -> [w3099 w3105]
                        tunnel: w3093 -> [w3101 w3118]
                        tunnel: [w3101 w3117] -> _
                        tunnel: w3094 -> [w3102 w3116]
                        tunnel: w3092 -> [w3100 w3115]
                        tunnel: [w3102 w3114] -> _
                        tunnel: [w3100 w3113] -> _
                        frame False {
                        }
                        frame True {
                          n1120 = property on="nb_images (set)" class="DigNum (strict)"() -> ("Value"=w3124:u32)  [unwired: 2 in, 2 out]
                          n1121 = case shown="2, Default" w3124 {
                            tunnel: [w3213 w3215] -> w3108
                            tunnel: w3119 -> [w3212 _]
                            tunnel: w3123 -> [w3213 _]
                            tunnel: [w3212 w3214] -> w3107
                            tunnel: w3122 -> [_ w3215]
                            tunnel: w3121 -> [_ w3214]
                            frame 2, Default {
                            }
                            frame 1 {
                            }
                          }
                          n1122 = stacked-sequence {
                            tunnel: w3108 -> [_ w3142]
                            tunnel: w3107 -> [_ w3141]
                            tunnel: [_ w3140] -> w3104
                            tunnel: [_ w3138] -> w3103
                            tunnel: [_ w3137] -> _
                            tunnel: w3106 -> [_ w3134]
                            tunnel: w3105 -> [_ w3133]
                            frame #0 {
                              # "Delay until MD gets stable"
                              n1123 = local read "exposure_duration_s (set)"() -> (w3125:dbl)
                              n1124 = local read "nb_images (set)"() -> (w3126:u32)
                              n1125 = Multiply(x=w3125, y=w3126) -> (x*y=w3127:dbl)
                              n1126 = Add(x=w3127, y=3.0) -> (x+y=w3128:dbl)
                              n1127 = Multiply(x=w3128, y=1000.0) -> (x*y=w3132:dbl)
                              n1128 = To Unsigned Long Integer(number=w3132) -> (unsigned 32bit integer=w3131:u32)
                              n1129 = Wait (ms)(milliseconds to wait=w3131) -> ()  [unwired: 1 out]
                            }
                            frame #1 {
                              n1130 = while {
                                tunnel: w3134 -> [w3147]
                                tunnel: [w3146] -> w3136
                                tunnel: w3133 -> [w3144]
                                tunnel: [w3143] -> w3135
                                stop <- w3145 stop-if-true
                                n1131 = call <userlib>:"LVClass_Camera asynchroneImageReady.vi"("Camera in"=w3147, "error in (no error)"=w3144) -> ("Camera out"=w3146:refnum<class "Camera.lvclass">, "ready"=w3145:bool, "error out"=w3143:errorcluster)  [unwired: 11 in]
                              }
                              n1132 = call <userlib>:"LVClass_Camera get image.vi"("Camera in"=w3136, "Image"=w3142, "Image RAW"=w3141, "remove_background"=FALSE, "error in (no error)"=w3135) -> ("Camera out"=w3137:refnum<class "Camera.lvclass">, "Image (dup)"=w3140:refnum<class "Image.lvclass">, "error out"=w3138:errorcluster)  [unwired: 7 in, 1 out]
                            }
                          }
                          n1133 = case shown="No Error" w3103 {
                            selector: w3103 -> [w3209 w3210]
                            tunnel: w3104 -> [w3206 w3211]
                            tunnel: [w3205 w3211] -> w3112
                            tunnel: [w3204 w3210] -> w3111
                            frame No Error {
                              # "get image"
                              n1134 = call <userlib>:"LVClass_Image get image data.vi"("Image in"=w3206, "error in (no error)"=w3209) -> ("Image out"=w3208:refnum<class "Image.lvclass">, "Image data out"=w3203:u32[][], "error out"=w3207:errorcluster)  [unwired: 11 in]
                              n1135 = call <userlib>:"LVClass_Image get image information.vi"("Image in"=w3208, "error in (no error)"=w3207) -> ("Image out"=w3205:refnum<class "Image.lvclass">, "error out"=w3204:errorcluster)  [unwired: 11 in, 1 out]
                              n1136 = local write "HASO intensity"(w3203) -> ()
                            }
                            frame Error {
                            }
                          }
                          n1137 = case shown="No Error" w3111 {
                            selector: w3111 -> [w3170 w3202]
                            tunnel: [w3176 w3202] -> w3120
                            tunnel: w3112 -> [w3169 _]
                            tunnel: [w3174 w3199] -> w3113
                            tunnel: [w3173 w3201] -> w3114
                            tunnel: refnum<class "HasoSlopes.lvclass"> refnum ("HasoSlopes in") -> [w3166 w3198]
                            tunnel: w3118 -> [w3165 w3200]
                            tunnel: [w3164 w3200] -> w3117
                            tunnel: w3116 -> [w3163 w3201]
                            tunnel: w3115 -> [w3161 w3199]
                            tunnel: [w3148 w3198] -> w3109
                            frame No Error {
                              # "phaseout"
                              n1138 = local read "File Base Name"() -> (w3153:string)
                              n1139 = local read "Save File"() -> (w3154:bool)
                              n1140 = local read "AO output"() -> (w3152:path)
                              n1141 = call "image2slopes.vi"("error in (no error)"=w3170, "Image in"=w3169, "HasoEngine in"=w3165, "HasoSlopes in"=w3166) -> ("error out"=w3149:errorcluster, "HasoEngine out"=w3164:refnum<class "HasoEngine.lvclass">, "HasoSlopes out"=w3148:refnum<class "HasoSlopes.lvclass">)  [unwired: 4 in, 1 out]
                              n1142 = local read "Filter"() -> (w3160:u8[])
                              n1143 = call "slopes2phase.vi"("TypePhase"=WavefrontReconstructionMode."Modal_Zernike", "Number of coefficients"=u8 32, "error in (no error)"=w3149, "Filter"=w3160, "HasoSlopes in"=w3148, "Phase in"=w3163) -> ("error out"=w3156:errorcluster, "HasoSlopes out"=w3157:refnum<class "HasoSlopes.lvclass">, "Phase out"=w3162:refnum<class "Phase.lvclass">)  [unwired: 3 in]
                              n1144 = local read "idxType"() -> (w3151:enum16{"Wyant", "ANSI"})
                              n1145 = call "slopes2zern.vi"("HasoSlopes in"=w3157, "error in (no error)"=w3156, "idxType"=w3151) -> ("Zernike Coefficients"=w3150:dbl[], "error out"=w3155:errorcluster)  [unwired: 3 in, 3 out]
                              n1146 = call <userlib>:"LVClass_Pupil ctor from HasoSlopes.vi"("Pupil in"=w3161, "HasoSlopes.lvclass"=w3148, "error in (no error)"=w3155) -> ("Pupil out"=w3171:refnum<class "Pupil.lvclass">, "error out"=w3172:errorcluster)  [unwired: 11 in]
                              n1147 = case shown="True" w3154 {
                                tunnel: w3153 -> [_ w3181]
                                tunnel: w3152 -> [_ w3180]
                                tunnel: w3150 -> [_ w3179]
                                tunnel: w3148 -> [_ w3178]
                                frame False {
                                }
                                frame True {
                                n1148 = stacked-sequence {
                                tunnel: w3181 -> [w3185 w3191]
                                tunnel: w3180 -> [w3184 w3190]
                                tunnel: w3179 -> [_ w3189]
                                tunnel: w3178 -> [w3182 _]
                                frame #0 {
                                n1149 = Concatenate Strings(w3185, "_slopesOffset", ".has") -> (w3188:string)
                                n1150 = Build Path(base path=w3184, name or relative path=w3188) -> (appended path=w3183:path)
                                n1151 = call <userlib>:"LVClass_HasoSlopes Save.vi"("HasoSlopes in"=w3182, "path"=w3183) -> ()  [unwired: 12 in, 2 out]
                                }
                                frame #1 {
                                n1152 = Concatenate Strings(w3191, "_zernOffset", ".txt") -> (w3194:string)
                                n1153 = Build Path(base path=w3190, name or relative path=w3194) -> (appended path=w3195:path)
                                n1154 = Array To Spreadsheet String(array=w3189, 3:"%f") -> (spreadsheet string=w3196:string)  [unwired: 1 in]
                                n1155 = Write to Text File(file (use dialog)=w3195, text=w3196) -> ()  [unwired: 2 in, 3 out]
                                }
                                }
                                }
                              }
                              n1156 = call <userlib>:"LVClasse_Phase GetStatisticDatas.vi"("Phase in"=w3162, "error in (no error)"=w3172) -> ("Phase out"=w3177:refnum<class "Phase.lvclass">, "StatisticsData"=w3158:T2, "error out"=w3175:errorcluster)  [unwired: 11 in]
                              n1157 = local write "Phase statistics"(w3158) -> ()
                              n1158 = call <userlib>:"LVClasse_Phase Get Data.vi"("Phase in"=w3177, "Pupil"=w3171, "error in (no error)"=w3175) -> ("Phase out"=w3173:refnum<class "Phase.lvclass">, "data"=w3159:sgl[][], "Pupil (dup)"=w3174:refnum<class "Pupil.lvclass">, "error out"=w3176:errorcluster)  [unwired: 9 in]
                              n1159 = local write "Zernike Measured"(w3150) -> ()
                              n1160 = local write "Phase values"(w3159) -> ()
                            }
                            frame Error {
                            }
                          }
                          n1161 = call <userlib>:"LVClass_HasoSlopes dtor.vi"("HasoSlopes in"=w3109) -> ()  [unwired: 13 in, 2 out]
                        }
                      }
                    }
                  }
                  n1162 = Unbundle By Name(w3076) -> ("status"=w3077:bool)
                }
              }
            }
          }
        }
      }
      event "Exit": Value Change {
        # "STOP AND EXIT"
        n1163 = event-data() -> ()  [unwired: 1 in, 4 out]
        n1164 = case shown="False" w3221 {
          tunnel: w3229 -> [w3232 w3235]
          tunnel: [errorcluster {"status"=FALSE, "code"=0, "source"=""} ("error out") w3234] -> w3228
          tunnel: [w3232 w3233] -> w3227
          frame False {
          }
          frame True {
            n1165 = call <userlib>:"LVClass_Camera stop acquisition.vi"("Camera in"=w3235) -> ("Camera out"=w3233:refnum<class "Camera.lvclass">, "error out"=w3234:errorcluster)  [unwired: 13 in]
          }
        }
      }
      event Panel Close? {
        n1166 = event-data() -> ()  [unwired: 1 in, 1 out]
        n1167 = flat-sequence {
          tunnel: w3251 -> [w3257]
          tunnel: w3244 -> [w3254]
          tunnel: [w3256] -> w3237
          tunnel: [w3255] -> w3236
          tunnel: [w3259] -> w3249
          tunnel: [w3260] -> w3250
          tunnel: w3237 -> [w3260]
          tunnel: w3236 -> [w3259]
          frame #0 {
            n1168 = call <userlib>:"LVClass_Camera stop acquisition.vi"("Camera in"=w3257, "error in (no error)"=w3254) -> ("Camera out"=w3256:refnum<class "Camera.lvclass">, "error out"=w3255:errorcluster)  [unwired: 12 in]
          }
          frame #1 {
            n1169 = local write "HASO ready"(FALSE) -> ()
          }
        }
        n1170 = event-data("Discard?"=TRUE) -> ()  [unwired: 1 in, 1 out]
      }
    }
    n1171 = Wait (ms)(milliseconds to wait=u32 250) -> ()  [unwired: 1 out]
  }
  n1172 = invoke class="MG17Motor" method="StopCtrl"(reference=w11) -> ()  [unwired: 2 in, 3 out]
  n1173 = VISA Close(VISA resource name=w10, error in (no error)=w6) -> (error out=w8:errorcluster)
  n1174 = case shown="True" w39 {
    tunnel: w60 -> [w3261 w3268]
    tunnel: w59 -> [_ w3292]
    tunnel: w58 -> [_ w3291]
    tunnel: w57 -> [_ w3290]
    tunnel: w56 -> [_ w3289]
    tunnel: w55 -> [_ w3288]
    tunnel: w54 -> [_ w3287]
    tunnel: w24 -> [_ w3280]
    tunnel: w20 -> [_ w3279]
    tunnel: w19 -> [_ w3278]
    tunnel: w18 -> [_ w3277]
    tunnel: w16 -> [_ w3274]
    tunnel: w17 -> [_ w3269]
    tunnel: [w3261 w3266] -> w9
    tunnel: w5 -> [_ w3262]
    frame False {
    }
    frame True {
      n1175 = local read "Enable EMCCD"() -> (w3263:bool)
      n1176 = And(x=w3262, y=w3263) -> (x .and. y?=w3264:bool)
      n1177 = flat-sequence {
        tunnel: w3292 -> [w3348]
        tunnel: w3268 -> [w3346]
        tunnel: [w3348] -> w3306
        tunnel: w3287 -> [w3347]
        tunnel: [w3347] -> w3305
        tunnel: [w3346] -> w3304
        tunnel: w3291 -> [w3345]
        tunnel: w3290 -> [w3344]
        tunnel: w3289 -> [w3343]
        tunnel: w3288 -> [w3342]
        tunnel: [w3341] -> w3303
        tunnel: [w3340] -> w3302
        tunnel: [w3339] -> w3301
        tunnel: [w3338] -> w3300
        tunnel: [w3331] -> w3285
        tunnel: [w3332] -> w3283
        tunnel: [w3333] -> w3281
        tunnel: w3280 -> [w3337]
        tunnel: w3279 -> [w3336]
        tunnel: w3278 -> [w3335]
        tunnel: w3277 -> [w3334]
        tunnel: [w3330] -> w3275
        tunnel: w3274 -> [w3329]
        tunnel: [w3328] -> w3273
        tunnel: w3269 -> [w3327]
        tunnel: [w3327] -> w3270
        tunnel: w3306 -> [w3363]
        tunnel: w3305 -> [w3362]
        tunnel: w3304 -> [w3360]
        tunnel: [w3362] -> w3299
        tunnel: [w3361] -> w3298
        tunnel: [w3360] -> w3297
        tunnel: w3303 -> [w3359]
        tunnel: [w3359] -> w3296
        tunnel: w3302 -> [w3358]
        tunnel: [w3358] -> w3295
        tunnel: w3301 -> [w3357]
        tunnel: [w3357] -> w3294
        tunnel: w3300 -> [w3356]
        tunnel: [w3356] -> w3293
        tunnel: [w3355] -> w3286
        tunnel: w3285 -> [w3355]
        tunnel: [w3354] -> w3284
        tunnel: w3283 -> [w3354]
        tunnel: [w3353] -> w3282
        tunnel: w3281 -> [w3353]
        tunnel: [w3352] -> w3276
        tunnel: w3275 -> [w3352]
        tunnel: w3273 -> [w3351]
        tunnel: [w3351] -> w3272
        tunnel: [w3350] -> w3271
        tunnel: w3270 -> [w3349]
        tunnel: w3299 -> [w3379]
        tunnel: w3298 -> [w3377]
        tunnel: w3297 -> [w3376]
        tunnel: w3296 -> [w3375]
        tunnel: w3295 -> [w3374]
        tunnel: w3294 -> [w3373]
        tunnel: w3293 -> [w3372]
        tunnel: w3286 -> [w3371]
        tunnel: w3284 -> [w3370]
        tunnel: w3282 -> [w3369]
        tunnel: w3276 -> [w3368]
        tunnel: w3272 -> [w3367]
        tunnel: w3271 -> [w3366]
        tunnel: [w3364] -> w3265
        frame #0 {
          n1178 = call <userlib>:"LVClass_Image dtor.vi"("Image in"=w3344) -> ("error out"=w3340:errorcluster)  [unwired: 13 in, 1 out]
          n1179 = local write "HASO ready"(FALSE) -> ()
          n1180 = call <userlib>:"LVClass_HasoSlopes dtor.vi"("HasoSlopes in"=w3337) -> ("error out"=w3332:errorcluster)  [unwired: 13 in, 1 out]
          n1181 = call <userlib>:"LVClass_Pupil dtor.vi"("Pupil in"=w3334) -> ("error out"=w3330:errorcluster)  [unwired: 13 in, 1 out]
          n1182 = call <userlib>:"LVClass_Image dtor.vi"("Image in"=w3342) -> ("error out"=w3338:errorcluster)  [unwired: 13 in, 1 out]
          n1183 = call <userlib>:"LVClass_WavefrontCorrector dtor.vi"("WavefrontCorrector in"=w3329) -> ("error out"=w3328:errorcluster)  [unwired: 13 in, 1 out]
          n1184 = call <userlib>:"LVClass_Image dtor.vi"("Image in"=w3345) -> ("error out"=w3341:errorcluster)  [unwired: 13 in, 1 out]
          n1185 = call <userlib>:"LVClass_Image dtor.vi"("Image in"=w3343) -> ("error out"=w3339:errorcluster)  [unwired: 13 in, 1 out]
          n1186 = call <userlib>:"LVClass_HasoEngine dtor.vi"("HasoEngine in"=w3335) -> ("error out"=w3331:errorcluster)  [unwired: 13 in, 1 out]
          n1187 = call <userlib>:"LVClasse_Phase dtor.vi"("Phase in"=w3336) -> ("error out"=w3333:errorcluster)  [unwired: 13 in, 1 out]
        }
        frame #1 {
          n1188 = call <userlib>:"LVClass_Camera dtor.vi"("Camera in"=w3363) -> ("error out"=w3361:errorcluster)  [unwired: 13 in, 1 out]
          n1189 = call <userlib>:"LVClass_WavefrontCorrectorSet dtor.vi"("WavefrontCorrectorSet in"=w3349) -> ("error out"=w3350:errorcluster)  [unwired: 13 in, 1 out]
        }
        frame #2 {
          n1190 = call <userlib>:"LVClass_CameraSet dtor.vi"("CameraSet.lvclass"=w3379) -> ("error out"=w3378:errorcluster)  [unwired: 13 in, 1 out]
          n1191 = local write "Current status"("Shut down") -> ()
          n1192 = Merge Errors(w3378, w3377, w3376, w3375, w3374, w3373, w3372, w3369, w3370, w3371, w3368, w3367, w3366) -> (w3364:errorcluster)
        }
      }
      n1193 = case shown="True" w3264 {
        tunnel: w3268 -> [w3307 w3310]
        tunnel: [w3307 w3309] -> w3267
        frame False {
        }
        frame True {
          # "Turn OFF EMCCD"
          n1194 = case shown="True" "TurnOFFCooler" {
            tunnel: w3310 -> [w3312 w3314]
            tunnel: [w3312 w3313] -> w3311
            frame False {
            }
            frame True {
              n1195 = stacked-sequence {
                tunnel: w3314 -> [w3315 w3317]
                tunnel: [_ w3316] -> w3313
                frame #0 {
                  n1196 = call <userlib>:"CoolerOFF.vi"("error in (no error)"=w3315) -> ()  [unwired: 1 in, 2 out]
                }
                frame #1 {
                  n1197 = while {
                    tunnel: w3317 -> [_]
                    tunnel: [w3319] -> w3316
                    stop <- w3321 continue-if-true
                    n1198 = call <userlib>:"GetTemperature.vi"() -> ("error out"=w3319:errorcluster, "temperature"=w3318:i32)  [unwired: 4 in, 2 out]
                    n1199 = local write "Current Temp"(w3318) -> ()
                    n1200 = Wait Until Next ms Multiple(millisecond multiple=u32 500) -> ()  [unwired: 1 out]
                    n1201 = Less?(x=w3318, y=i16 0) -> (x < y?=w3321:bool)
                  }
                }
              }
            }
          }
          n1202 = case shown="No Error" w3311 {
            tunnel: w3311 -> [w3324 w3325]
            tunnel: [w3323 w3325] -> w3309
            frame No Error {
              n1203 = call <userlib>:"ShutDown.vi"("error in (no error)"=w3324) -> ("error out"=w3323:errorcluster)  [unwired: 1 in, 1 out]
            }
            frame Error {
            }
          }
        }
      }
      n1204 = Merge Errors(w3265, w3267) -> (w3266:errorcluster)
    }
  }
  n1205 = Merge Errors(w9, w8) -> (w7:errorcluster)
  n1206 = property on="Current error" class="Clust (strict)"("Value"=w7) -> ()  [unwired: 2 in, 2 out]
